vi "Gestore procedure.vi"() -> ()   [LabVIEW 2019]
uses:
  TypeDef/Operazioni.ctl
  TypeDef/PROCEDURE.ctl
  TypeDef/Control 1.ctl
  TypeDef/Impostazioni elettriche.ctl
  TypeDef/Collegamenti_elettrici.ctl
  TypeDef/Control rotore bloccato.ctl
  cDAQ_PLC Folder/cDAQ/SET ARRAY DO.ctl
  cDAQ_PLC Folder/cDAQ/SET SINGLE DO.ctl
  cDAQ_PLC Folder/cDAQ/DO List.ctl
  cDAQ_PLC Folder/cDAQ/SET ARRAY AO.ctl
  cDAQ_PLC Folder/cDAQ/SET SINGLE AO.ctl
  cDAQ_PLC Folder/cDAQ/AO List.ctl
  TypeDef/Cluster INFO.ctl
  TypeDef/WT SELECTION.ctl
  TypeDef/Definizione linea.ctl
  TypeDef/Control Calcoli.ctl
  Stato comandi freno.vi
  Stato alimentatore 1.vi
  Global FINE AVVIO.vi
  SubVI ELETTROTEST60A Folder/Elettrotest60A/Global_bypass_ResMeter.vi
  Global prova in corso.vi
  Global Trampa 0.vi
  Global stato profilo.vi
  Global Fine procedure.vi
  Global_All_Data.vi
  Global allarmi procedure.vi
panel:
  out "Elements In Queue":T1(array[cluster])
  out "Data":T2
  out "RESISTOMAT":T3
  out "PROCEDURA":string="MISURA RESISTENZA..."
  out "Element":T4
  out "OPERAZIONE IN CORSO":T5=enum."FRENO SET RIF PARTENZA"
  out "Message":string
  out "Stato":string
  out "Rami misura":i32
  out "Vi abilita pot":refnum<vi>
  out "Vi chiudi teler pot":refnum<vi>
  out "TEMPO PROVA ROT BLOCC":dbl
  in  "Cluster Colleg/LInea Elettrica":T6
  in  "AGGIUNGI PROCEDURA Abilita potenza":bool
  in  "AGGIUNGI PROCEDURA \nSTOP":bool
  in  "AGGIUNGI PROCEDURA \nSTART":bool
  in  "Cluster":T7={"MODALITA' BANCO"=enum."ALIMENTATORE E FRENO", "MODALITA' AVVIO MOTORE"=enum."AVVIO A TENSIONE RIDOTTA", "MODALITA' AVVIO FRENO"=enum."MARCIA PRIMA AVVIO", "V avvio[V]"=0.0, "F avvio[Hz]"=0.0, "%V ridotta"=0.0, "C avvio [Nm]"=0.0, "RPM avvio"=0.0, "SERVO AVVIO"=FALSE, "SENSO DI ROTAZIONE"=FALSE}
  out "Operazioni in corso":T5[](array[typedef])
  in  "EXIT":bool
  out "Matrice procedure":T5[][](array[typedef])
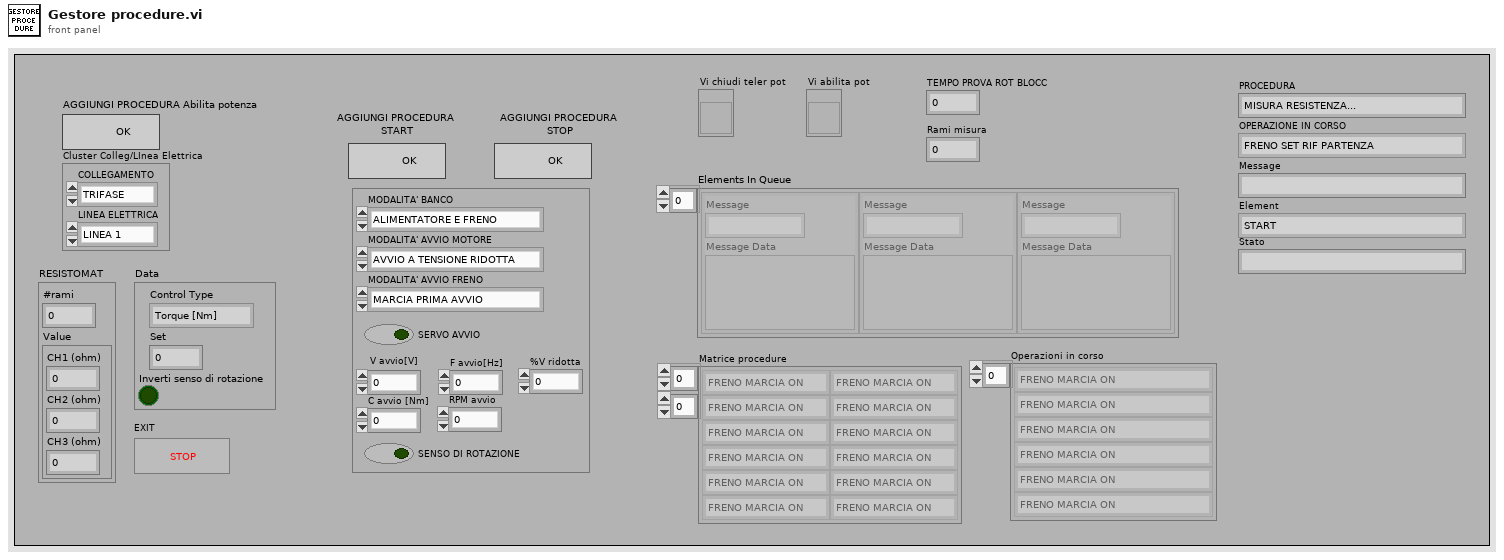
[diagram p1: front panel]
types:
  T1 = cluster{"Message":string, "Message Data":variant}[]
  T2 = cluster{"Control Type":enum32{"Torque [Nm]", "Power [W]", "Speed [RPM]"}, "Set":dbl, "Inverti senso di rotazione":bool}
  T3 = cluster{"#rami":i32, "Value":cluster{"CH1 (ohm)":u16, "CH2 (ohm)":u16, "CH3 (ohm)":u16}}
  T4 = typedef "PROCEDURE.ctl" = enum16{"START", "STOP AUTOMATICO", "STOP FRENO", "ABILITA POTENZA", "DISABILITA POTENZA", "CHIUDI POTENZA", "APRI POTENZA", "MISURA RESISTENZA RESISTOMAT", "PROVA ROTORE BLOCCATO", "MISURA RESISTENZA RES METER", "START AFE ALTERNATORI", "STOP AFE ALTERNATORI", "STOP ALIMENTATORE", "CONFIG CONTROLLO FRENO", "ALLARME", "START PROFILO", "SVUOTA BUFFER PROCEDURE E OPERAZIONI"}
  T5 = typedef "Operazioni.ctl" = enum32{"FINE", "FRENO ABILITA", "FRENO DISABILITA", "FRENO MARCIA ON", "FRENO MARCIA OFF", "FRENO SET RIF PARTENZA", "FRENO FORZA RIF FERMATA", "FRENO SET RIF FERMATA", "FRENO SET RIF A 0", "FRENO FORZA RIF A 0", "FRENO SET CONTROLLO COPPIA", "FRENO SET CONTROLLO VELOCITA'", "FRENO SET SENSO ROTAZIONE", "FRENO SET SENS ROT SEGNO COPPIA", "FRENO CONFIG", "ALIMENTATORE 1 ABILITA", "ALIMENTATORE 1 DISABILITA", "ALIMENTATORE 1 MARCIA ON", "ALIMENTATORE 1 MARCIA OFF", "ALIMENTATORE 1 SET RIF", "ALIMENTATORE 1 SET RIF RIDOTTO", "ALIMENTATORE 1 SET RIF A 0", "ALIMENTATORE 1 RESET ALLARMI", "ALIMENTATORE 1 SCORTA 2", "ALIMENTATORE 1 SCORTA 3", "ALIMENTATORE 2 ABILITA", "ALIMENTATORE 2 DISABILITA", "ALIMENTATORE 2 MARCIA ON", "ALIMENTATORE 2 MARCIA OFF", "ALIMENTATORE 2 SET RIF", "ALIMENTATORE 2 SET RIF RIDOTTO", "ALIMENTATORE 2 SET RIF A 0", "ALIMENTATORE 2 SCORTA 1", "ALIMENTATORE 2 SCORTA 2", "ALIMENTATORE 2 SCORTA 3", "TELERUTTORI CHIUDI POTENZA", "TELERUTTORI APRI POTENZA", "TELERUTTORI ABILITA POTENZA", "TELERUTTORI DISABILITA POTENZA", "TELERUTTORI MISURA RESISTENZA RESISTOMAT", "TELERUTTORI MISURA RESISTENZA RES METER", "PROCEDURA ROTORE BLOCCATO 1", "ATTENDI FERMATA MOTORE", "SEGNALA INIZIO AVVIO", "SEGNALA FINE AVVIO", "SEGNALA INIZIO FERMATA", "SEGNALA FINE FERMATA", "START PROFILO", "ATTENDI FINE RAMPA"}
  T6 = typedef "Control 1.ctl" = cluster{"COLLEGAMENTO":enum16{"TRIFASE", "MONOFASE", "DC MP", "DC"}, "LINEA ELETTRICA":enum16{"LINEA 1", "LINEA 2", "LINEA 3", "LINEA 4", "LINEA 5"}}
  T7 = typedef "Modalità avvio.ctl" = cluster{"MODALITA' BANCO":enum32{"ALIMENTATORE E FRENO", "SOLO ALIMENTATORE", "SOLO FRENO", "GESTIONE MANUALE", "SOLO ACQUISITORE", "VARIAC"}, "MODALITA' AVVIO MOTORE":enum32{"AVVIO A TENSIONE RIDOTTA", "AVVIO IN RAMPA", "AVVIO DIRETTO DA ALIM", "AVVIO DIRETTO DA LINEA"}, "MODALITA' AVVIO FRENO":enum32{"MARCIA DOPO AVVIO MOTORE", "MARCIA PRIMA AVVIO"}, "V avvio[V]":dbl, "F avvio[Hz]":dbl, "%V ridotta":dbl, "C avvio [Nm]":dbl, "RPM avvio":dbl, "SERVO AVVIO":bool, "SENSO DI ROTAZIONE":bool}
  T8 = cluster{"Message":string, "Message Data":variant}
  T9 = typedef "Impostazioni elettriche.ctl" = cluster{"COLLEGAMENTO":T10, "LINEA ELETTRICA":enum16{"LINEA 1", "LINEA 2", "LINEA 3", "LINEA 4", "LINEA 5"}}
  T10 = typedef "Collegamenti_elettrici.ctl" = enum16{"AC TRIFASE", "AC TRIFASE + FRENO", "AC MONOFASE", "DC CON ECCITAZIONE", "DC CON ECCITAZIONE + FRENO", "DC NO ECCITAZIONE", "DC NO ECCITAZIONE + FRENO", "FRENO TRASC + AFE", "SOLO FRENO", "CARICO RESISTIVO", "GENERICO", "SOLO ACQUISITORE", "SCORTA 4", "SCORTA 5", "SCORTA 6"}
  T11 = typedef "Control rotore bloccato.ctl" = cluster{"TEMPO PROVA":dbl}
  T12 = cluster{"Array of elements":cluster{"String":string, "variant":variant}[], "Single element":cluster{"String":string, "variant":variant}, "enque at\nopposite end (F)":bool, "no replications (F)":bool}
  T13 = typedef "SET ARRAY DO.ctl" = T14[]
  T14 = typedef "SET SINGLE DO.ctl" = cluster{"DO":T15, "Value":bool}
  T15 = typedef "DO List.ctl" = enum16{"OFF: ALL DO", "*ABILITA freno 1", "*ABILITA freno 2", "*ABILITA freno 3", "*START freno 1", "*START freno 2", "*START freno 3", "*STOP freno 1", "*STOP freno 3", "*STOP freno 2", "*Senso rot freno 1", "*Senso rot freno 2", "*Senso rot freno 3", "*Ctrl velocità freno 1", "*Ctrl velocità freno 2", "*Ctrl velocità freno 3", "*Ctrl coppia freno 1", "*Ctrl coppia freno 2", "*Ctrl coppia freno 3", "*ABILITA alimentatore 1", "*ABILITA alimentatore 2", "*ABILITA alimentatore 3", "*ABILITA alimentatore 4", "*START alimentatore 1", "*START alimentatore 2", "*START alimentatore 3", "*START alimentatore 4", "*STOP alimentatore 1", "*STOP alimentatore 2", "*STOP alimentatore 3", "*STOP alimentatore 4", "SENSO ROT alimentatore 1", "SENSO ROT alimentatore 2", "Abilita LEM 1000A", "Abilita LEM 300A", "Abilita sensori EXT WT", "B1 Seleziona linea 1", "B1 Seleziona linea 2", "B1 Seleziona linea 3", "B1 Seleziona linea 4", "B1 Seleziona linea 5", "B2 Seleziona linea 1", "B2 Seleziona linea 2", "B2 Seleziona linea 3", "B2 Seleziona linea 4", "B2 Seleziona linea 5", "*Reset allarmi", "*Start potenza AC", "*Stop potenza AC", "*Start potenza DC", "*Stop potenza DC", "*Start potenza DC eccit", "*Stop pontenza DC eccit", "Bypass res meter", "2nd canale res meter", "Enable res meter", "*Abilit teler ramo WT", "*Abil teler ramo princ Resit", "*Abil teler ramo 1 Resist", "*Abil teler ramo 2 Resist", "*Abil teler ramo 3 Resist", "*Abil cortocirc avvolgim", "*Controllo torsiometro B1", "*Controllo Torsiom B2", "*Scala torsiometro B1", "*Scala torsiometro B2", "*Collaudo in corso", "*Allarme presente", "Abilitazione elettroserratura", "Exit", "*Abilita collaudo", "*Abilita potenza trifase", "*Abilita potenza monofase", "*Abilita potenza DC", "*Abilita potenza DC eccit", "*Disabilita teleruttori potenza", "Set teleruttori prova a freddo", "Prova a freddo monofase", "Watchdog", "Forza DO PLC 3", "Forza DO PLC 2", "Forza DO PLC 1", "Forza DO cDAQ", "Scala 2000(T) 200(F) res meter", "Seleziona banco 1", "Seleziona banco 2", "Comando azionam in blocco", "Comando azionam reset", "Sensibilità freno 16 32 nm", "Reset Allarmi", "Carico res - Ramo 1", "Carico res - Ramo 2", "Carico res - Ramo 3", "Carico res - Ramo 4", "Carico res - Ramo 5", "Carico res - Ramo 6", "Carico res - Ramo 7", "Carico res - Ramo 8", "Carico res - Ramo 9", "Carico res - Ramo 10", "Carico res - Ramo 11", "Carico res - Start ventilatore", "Carico res - Stop ventilatore", "Abilita potenza solo freno", "Abilita AFE + freno trasc", "Abilita potenza carico resistivo", "Chiudi potenza AFE", "Apri potenza AFE", "Start AFE", "Config Banco2 TDE", "Misura diretto WT", "Ripristina centralina protezioni", "Abilita Scrittura Dati Keb", "Bench Selection(0-B1,1-B2)", "Select current mode", "Select torque mode", "Select speed mode", "Extenal alarm", "Enable Extenal program ", "Start ", "Stop", "Enable force mode", "Abilita linea 125 A", "Abilita linea 63 A", "Abilita linea 16 A", "Aum Tensione Variac", "Dim Tesnione Variac", "Abilita Ellecto Stractura", "Riprinto Emergenxe ", "Abilita Collaudo", "Disabilita Collaudo", "Abilita Ingresso Variac", "Abilita Uscita Variac", "Abilita ventilatore Variac"}
  T16 = enum32{"Torque [Nm]", "Power [W]", "Speed [RPM]"}
  T17 = typedef "SET ARRAY AO.ctl" = T18[]
  T18 = typedef "SET SINGLE AO.ctl" = cluster{"AO":T19, "Value":dbl}
  T19 = typedef "AO List.ctl" = enum16{"OFF: ALL AO", "RIF VEL FRENO 1", "RIF VEL FRENO 2", "RIF VEL FRENO 3", "RIF COPPIA FRENO", "RIF COPPIA FRENO 1", "RIF COPPIA FRENO 2", "RIF COPPIA FRENO 3", "RIF CORRENTE FRENO 2", "RIF V ALIM 1", "RIF F ALIM 1", "RIF V ALIM 2", "RIF F ALIM 2", "RIF V ALIM 3", "RIF F ALIM 3", "RIF V ALIM 4", "RIF F ALIM 4", "FORZA AO PLC 3", "FORZA AO PLC 2", "FORZA AO PLC 1", "FORZA AO cDAQ", "Configura alimentatore keb", "Tempo rampa keb", "Condensatori", "Exit"}
  T20 = cluster{"N°Acq":i16, "Periodo":dbl, "acq in corso":bool, "Acquisizione":bool, "Slide":u8, "Inserisci Acq.":bool, "Elimina riga":bool, "Acq auto":bool, "Intervallo":dbl}
  T21 = typedef "Cluster INFO.ctl" = cluster{"Scelta wattmetro":cluster{"Wattmetro":T22}, "SET RPM":dbl, "SET TEMP":dbl, "Array banchi":T23[], "Array valvole linee avvio/fermata":cluster{"Valvole avvio":cluster{"Set valvole avvio?":bool, "% valvole avvio":dbl[]}, "Valvole fermata":cluster{"Set valvole fermata?":bool, "% valvole fermata":dbl[]}}[], "banco selezionato":i8, "Nomi valvole prop sistema":string[], "canale-- sensore":string[][], "Attriti B1":dbl[][], "Attriti B2":dbl[][], "Collegamento elettrico":cluster{"ALIMENTAZIONE ELETTRICA":T10, "ID":i16, "#rami freddo\\eq term resmeter":i16, "#rami riscaldamento resmeter":i16, "#rami freddo\\eq term resistomat":i16, "#rami riscaldamento resistomat":i16, "CALCOLI":T24}, "lingua":i16, "Costanti collaudo":cluster{"P [bar]":dbl, "T amb. [°C]":dbl, "Umidità [%]":dbl, "T acqua [°C] 2":dbl}, "OPZIONI MISURE RES":cluster{"MISURA A FREDDO":enum16{"NESSUNO", "RESISTOMAT", "RES METER", "ENTRAMBI"}, "MISURA EQ. TERMICO":enum16{"NESSUNO", "RESISTOMAT", "RES METER", "ENTRAMBI"}, "MISURA DT PROVA IN CORSO":enum16{"NESSUNO", "RESISTOMAT - CON FERMATE", "RES METER - CON FERMATE", "RES METER - CONTINUO"}, "MISURE PRIMA E DOPO":enum16{"NESSUNO", "RESISTOMAT", "RES METER"}, "STRUMENTI PRESENTI":enum16{"NESSUNO", "RESISTOMAT", "RES METER", "ENTRAMBI"}}, "Dati targa motore":cluster{"Vnom":dbl, "Fnom":dbl, "Inom":dbl, "Cnom":dbl, "Npoli":dbl, "Scorta 1":dbl, "Scorta 2":dbl, "Scorta 3":dbl}}
  T22 = typedef "WT SELECTION.ctl" = enum32{"No Selection", "WT230", "WT333", "WT1800", "WT330", "VIW", "APLUS"}
  T23 = typedef "Definizione linea.ctl" = cluster{"Nome":string, "Tors. scala1":i32, "Tors. scala2":i32, "rpm":i32, "TAMB":i32, "Indici Temperature":i16[], "Indice freno":i16, "alimentatore trifase":i16, "alimentatore monofase":i16, "alimentatore dc arm":i16, "alimentatore dc ecc":i16, "alimentatore dc mp":i16}
  T24 = typedef "Control Calcoli.ctl" = enum16{"AC TRIFASE", "AC MONOFASE", "DC ECCITAZIONE", "DC NO ECCITAZIONE", "POMPA TRIFASE", "POMPA MONOFASE", "GENERICO", "TRASFORMATORE", "ALTERNATORE TRASCINATO", "GRUPPO ELETTROGENO"}
  T25 = typedef "Stato inverter selezionato.ctl" = cluster{"Stato comandi freno":T26, "Stato":cluster{"rif C%":dbl, "rif vel%":dbl, "Controllo effettivo":enum32{"Torque [Nm]", "Power [W]", "Speed [RPM]"}, "Controllo desiderato":enum32{"Torque [Nm]", "Power [W]", "Speed [RPM]"}, "Fine rampa C":bool, "Fine rampa RPM":bool, "Senso rotaz":bool, "Start":bool, "C stabile":bool, "P stabile":bool, "RPM stabile":bool}}
  T26 = typedef "Comandi freno.ctl" = cluster{"Control":cluster{"Control Type":enum32{"Torque [Nm]", "Power [W]", "Speed [RPM]", "Corrente [A]"}, "Set":dbl, "Inverti senso di rotazione":bool}, "Start\\stop":cluster{"Start":bool, "STOP":bool}, "Status":cluster{"Ready":bool, "Running":bool, "Regulation":bool}, "PID":bool, "Abilita":cluster{"Abilita":bool}, "Status ref":cluster{"Torque":dbl, "Speed":dbl}}
  T27 = typedef "Comandi_Alimentatore.ctl" = cluster{"RIF 1":dbl, "RIF 2":dbl, "Status":cluster{"Ready":bool, "Running":bool, "Regulation":bool}, "Start\\stop":cluster{"Start":bool, "Stop":bool}, "PID RIF1":bool, "PID RIF2":bool, "Status ref":cluster{"RIF 1":dbl, "RIF 2":dbl}, "Abilita":cluster{"Abilita":bool}}
  T28 = cluster{"RIF 1":dbl, "RIF 2":dbl, "Abilitato":bool, "In marcia":bool, "Fine rampa RIF1":bool, "Fine rampa RIF2":bool, "Vstabile":bool, "F stabile":bool, "PID RIF1":bool, "PID RIF2":bool, "Alimentatore 1":T27}
  T29 = cluster{"rif C%":dbl, "rif vel%":dbl, "Controllo effettivo":enum32{"Torque [Nm]", "Power [W]", "Speed [RPM]"}, "Controllo desiderato":enum32{"Torque [Nm]", "Power [W]", "Speed [RPM]"}, "Fine rampa C":bool, "Fine rampa RPM":bool, "Senso rotaz":bool, "Start":bool, "C stabile":bool, "P stabile":bool, "RPM stabile":bool}
  T30 = enum32{"ALIMENTATORE E FRENO", "SOLO ALIMENTATORE", "SOLO FRENO", "GESTIONE MANUALE", "SOLO ACQUISITORE", "VARIAC"}
  T31 = enum32{"AVVIO A TENSIONE RIDOTTA", "AVVIO IN RAMPA", "AVVIO DIRETTO DA ALIM", "AVVIO DIRETTO DA LINEA"}
  T32 = enum32{"MARCIA DOPO AVVIO MOTORE", "MARCIA PRIMA AVVIO"}
  T33 = cluster{"IN ESECUZIONE":bool, "IN PAUSA":bool, "FINE":bool, "Tstep":dbl}
  T34 = typedef "Cluster MISURE.ctl" = cluster{"MISURE NM":T35, "MISURE ALL":T36}
  T35 = typedef "MISURE NM.ctl" = cluster{"Banco":string, "Anno":string, "Numero":string, "Ntabella":string, "Misura":string, "Tipo Prova":string, "ProgressivoAcq":string, "Descrizione":string, "Data_ora":string, "t. acq [h:m:s]":string, "t. acq [min]":string, "t. acq [s]":string, "n [rpm]":string, "f [Hz]":string, "U1[V]":string, "U2 [V]":string, "U3 [V]":string, "U123_media [V]":string, "I1[A]":string, "I2[A]":string, "I3[A]":string, "I123_media [A]*I":string, "I_123_sbil [%]":string, "Ulin[V]":string, "Uc [V]":string, "Uaux [V]":string, "Ilin[A]*I":string, "Imar[A]":string, "Iaux[A]":string, "Uarm[V]":string, "Uecc[V]":string, "Iarm[A]*I":string, "Iecc[A]":string, "pf":string, "P1 [W]":string, "P1 [kW]":string, "Q [VAR]":string, "Q [kVAR]":string, "S [VA]":string, "S [kVA]":string, "P1arm[W]":string, "P1ecc[W]":string, "Parm[kW]":string, "P1ecc[kW]":string, "Cond[uF]":string, "P1_linea_6fili[W]":string, "P1_linea_6fili[kW]":string, "eta_gr_6fili [%]":string, "eta_inverter_6fili [%]":string, "pf_linea_6fili":string, "U4 [V]":string, "U5 [V]":string, "U6 [V]":string, "U456_media [V]":string, "I4 [A]":string, "I5 [A]":string, "I6 [A]":string, "I456_media [A]":string, "C [Nm]*C":string, "Cric [Nm]":string, "Cric\\Cnom":string, "Iric[A]":string, "Iric\\Inom":string, "P2_mecc [W]":string, "P2_mecc [kW]":string, "eta motore [%]":string, "Scorr[%]":string, "Tamb[°C]":string, "R1[ohm]":string, "R2[ohm]":string, "R3[ohm]":string, "Rmedia[ohm]":string, "DT_R1[°C]":string, "DT_R2[°C]":string, "DT_R3[°C]":string, "DT_media[°C]":string, "R_marcia[ohm]":string, "R_aux[ohm]":string, "DT_marcia[°C]":string, "DT_aux[°C]":string, "R_Arm[ohm]":string, "R_Ecc[ohm]":string, "DT_Arm[°C]":string, "DT_Ecc[°C]":string, "TambFreddo[°C]":string, "R1_freddo[ohm]":string, "R2_freddo[ohm]":string, "R3_freddo[ohm]":string, "Rmedia_freddo[ohm]":string, "R_Marcia_freddo[ohm]":string, "R_Aux_freddo[ohm]":string, "R_Arm_freddo[ohm]":string, "R_Ecc_freddo[ohm]":string, "TC1 [°C]":string, "TC2 [°C]":string, "TC3 [°C]":string, "TC4 [°C]":string, "TC5 [°C]":string, "TC6 [°C]":string, "TC7 [°C]":string, "TC8 [°C]":string, "PT1000_1[°C]":string, "PT1000_2[°C]":string, "PT1000_3[°C]":string, "Vdc eccitatrice[V]":string, "Idc eccitatrice[A]":string, "Vdc rotore[V]":string, "Idc rotore[A]":string, "Vac rotore[V]":string, "Iac rotore[V]":string, "V dinamo[V]":string, "Portata Q":string, "Pressione H":string, "U1'[V]":string, "U2'[V]":string, "U3'[V]":string, "I1'[A]":string, "I2'[A]":string, "I3'[A]":string, "U''R-N":string, "U''S-N":string, "U'' T-N":string, "U''R-S":string, "U''R-T":string, "U''S-T":string, "I1''[A]":string, "I2''[A]":string, "I3''[A]":string, "F''[Hz]":string, "P''[kW]":string, "CosFi''":string, "PT1000_4[°C]":string, "Scorta 3":string}
  T36 = typedef "Cluster misure ALL.ctl" = cluster{"Cluster READ NI":T37, "MISURE WT":T40, "Resistenze Resistomat":T41, "INTERFACCIA":T42, "FREDDO resistomat":cluster{"Res Ch1":dbl, "Res Ch2":dbl, "tAMB":dbl, "Res Ch3":dbl}, "STATO PLC 1":T47, "Res Ch2":dbl, "Res Ch2 2":dbl, "FREDDO res meter":cluster{"Res Ch1":dbl, "Res Ch2":dbl, "tAMB":dbl, "Res Ch3":dbl}, "Resistenze Res Meter":T41, "READ SINUS PENTA":T51, "STATO PLC 2":T52, "STATO PLC 3":T56, "DCREG":T60}
  T37 = typedef "Cluster NI.ctl" = cluster{"AI (0-10V)":cluster{"AI 0":dbl, "AI 1":dbl, "AI 2":dbl, "AI 3":dbl, "AI 4":dbl, "AI 5":dbl, "AI 6":dbl, "AI 7":dbl, "AI 8":dbl, "AI 9":dbl, "AI 10":dbl, "AI 11":dbl, "AI 12":dbl, "AI 13":dbl, "AI 14":dbl, "AI 15":dbl, "AI 16":dbl, "AI 17":dbl, "AI 18":dbl, "AI 19":dbl, "AI 20":dbl, "AI 21":dbl, "AI 22":dbl, "AI 23":dbl, "AI 24":dbl, "AI 25":dbl, "AI 26":dbl, "AI 27":dbl, "AI 28":dbl, "AI 29":dbl, "AI 30":dbl, "AI 31":dbl}, "StatoAO_Cdaq[0-10V]":cluster{"AO 1":dbl, "AO 2":dbl, "AO 3":dbl, "AO 4":dbl}, "Contatori [rpm]":cluster{"RPM 1":dbl, "RPM 2":dbl}, "StatoAO_Cdaq [4-20mA]":T38, "StatoDO_Cdaq":T39, "DI":cluster{"Scorta 0":bool, "Scorta 1":bool, "Scorta 2":bool, "Scorta 3":bool, "Scorta 4":bool, "Scorta 5":bool, "Scorta 6":bool, "Scorta 7":bool, "Scorta 8":bool, "Scorta 9":bool, "Scorta 10":bool, "Scorta 11":bool, "Scorta 12":bool, "Scorta 13":bool, "Scorta 14":bool, "Scorta 15":bool, "Scorta 16":bool, "Scorta 17":bool, "Scorta 18":bool, "Scorta 19":bool, "Scorta 20":bool, "Scorta 21":bool, "Scorta 22":bool, "Scorta 23":bool, "Scorta 24":bool, "Scorta 25":bool, "Scorta 26":bool, "Scorta 27":bool, "Scorta 28":bool, "Scorta 29":bool, "Scorta 30":bool, "Scorta 31":bool}, "AI (4-20mA)":cluster{"AI 0":dbl, "AI 1":dbl, "AI 2":dbl, "AI 3":dbl, "AI 4":dbl, "AI 5":dbl, "AI 6":dbl, "AI 7":dbl, "AI 8":dbl, "AI 9":dbl, "AI 10":dbl, "AI 11":dbl, "AI 12":dbl, "AI 13":dbl, "AI 14":dbl, "AI 15":dbl}, "TC [°C]":cluster{"tc 1":dbl, "tc 2":dbl, "tc 3":dbl, "tc 4":dbl}, "NI Read Values":cluster{"RPM":dbl, "Frequency":dbl, "Mod 1":cluster{"Torsiometro 1":dbl, "Torsiometro 2":dbl, "Strin Gauge 1":dbl, "Strin Gauge 2":dbl}, "Mod 2":cluster{"Termocoppia 1":dbl, "Termocoppia 2":dbl, "Termocoppia 3":dbl, "Termocoppia 4":dbl}, "Mod 3":cluster{"PT 100 1":dbl, "PT 100 2":dbl, "PT 100 3":dbl, "PT 100 4":dbl}}}
  T38 = typedef "StatoAO_cdaq.ctl" = cluster{"Cdaq_AO [0-10V] 0 for Torque":dbl, "Cdaq_AO [0-10V] 1":dbl, "Cdaq_AO [0-10V] 2":dbl, "Cdaq_AO [0-10V] 3":dbl}
  T39 = typedef "statoDO_Cdaq.ctl" = cluster{"Scorta 0":bool, "Scorta 1":bool, "Scorta 2":bool, "Scorta 3":bool, "Scorta 4":bool, "Scorta 5":bool, "Scorta 6":bool, "Scorta 7":bool, "Scorta 8":bool, "Scorta 9":bool, "Scorta 10":bool, "Scorta 11":bool, "Scorta 12":bool, "Scorta 13":bool, "Scorta 14":bool, "Scorta 15":bool, "Scorta 16":bool, "Scorta 17":bool, "Scorta 18":bool, "Scorta 19":bool, "Scorta 20":bool, "Scorta 21":bool, "Scorta 22":bool, "Scorta 23":bool, "Scorta 24":bool, "Scorta 25":bool, "Scorta 26":bool, "Scorta 27":bool, "Scorta 28":bool, "Scorta 29":bool, "Scorta 30":bool, "Scorta 31":bool}
  T40 = typedef "MISURE WT.ctl" = cluster{"URMS 1":dbl, "IRMS 1":dbl, "P 1":dbl, "S 1":dbl, "Q 1":dbl, "LAMBDA 1":dbl, "PHI 1":dbl, "F U 1":dbl, "F I 1":dbl, "NONE 1":dbl, "URMS 2":dbl, "IRMS 2":dbl, "P 2":dbl, "S 2":dbl, "Q 2":dbl, "LAMBDA 2":dbl, "PHI 2":dbl, "F U 2":dbl, "F I 2":dbl, "NONE 2":dbl, "URMS 3":dbl, "IRMS 3":dbl, "P 3":dbl, "S 3":dbl, "Q 3":dbl, "LAMBDA 3":dbl, "PHI 3":dbl, "F U 3":dbl, "F I 3":dbl, "NONE 3":dbl, "URMS SIGMA":dbl, "IRMS SIGMA":dbl, "P SIGMA":dbl, "S SIGMA":dbl, "Q SIGMA":dbl, "LAMBDA SIGMA":dbl, "PHI SIGMA":dbl, "F U SIGMA":dbl, "F I SIGMA":dbl, "NONE 4":dbl}
  T41 = typedef "ClusterRes.ctl" = cluster{"Res Ch1":dbl, "Res Ch2":dbl, "Res Ch3":dbl, "Tamb":dbl}
  T42 = typedef "INTERFACCIA.ctl" = cluster{"AI":cluster{"Portate":T43[], "Pressioni":T43[], "Coppie[Nm]":T43[], "Valvole prop %":T43[], "RPM":T43[], "Livelli":T43[], "Temperature":T43[], "Riferimenti %":T43[], "TENSIONI":T43[], "CORRENTI":T43[]}, "DI (logici)":cluster{"Start da pulsantiera":bool, "Stop da pulsantiera":bool, "Reset da pulsantiera":bool, "Sistema OK":bool, "Collaudo abilitato":bool, "Potenza trifase abilitata":bool, "Potenza monofase abilitata":bool, "Potenza DC abilitata":bool, "Potenza DC ECC abilitata":bool, "Start alimentazione AC":bool, "Start alimentazione DC":bool, "Start DC eccitazione":bool, "Teleruttore WT abilitato":bool, "Teleruttore Resistomat abilitato":bool, "Teleruttore corto fasi":bool, "Ramo 1 resistomat":bool, "Ramo 2 resistomat":bool, "Ramo 3 resistomat":bool, "B1 Scelta linea elettrica 1":bool, "B1 Scelta linea elettrica 2":bool, "B1 Scelta linea elettrica 3":bool, "B1 Scelta linea elettrica 4":bool, "B1 Scelta linea elettrica 5":bool, "B2 Scelta linea elettrica 1":bool, "B2 Scelta linea elettrica 2":bool, "B2 Scelta linea elettrica 3":bool, "B2 Scelta linea elettrica 4":bool, "B2 Scelta linea elettrica 5":bool, "Rotore bloccato 1":bool, "Rotore bloccato 2":bool, "FRENO 1 abilitato":bool, "FRENO 1 run":bool, "FRENO 1 senso rotaz":bool, "FRENO 1 ctrl velocità":bool, "FRENO 2 abilitato":bool, "FRENO 2 run":bool, "FRENO 2 senso rotaz":bool, "FRENO 2 ctrl velocità":bool, "ALIM 1 abilitato":bool, "ALIM 1 run":bool, "ALIM 2 abilitato":bool, "ALIM 2 run":bool, "ALIM 3 abilitato":bool, "ALIM 3 run":bool, "FRENO 1 ctrl coppia":bool, "FRENO 2 ctrl coppia":bool, "FRENO 3 ctrl coppia":bool, "DI (logici) aggiuntivi impianto":cluster{"Solo freno abilitato":bool, "Carico resistivo abilitato":bool, "AFE+freno abilitato":bool, "Protezioni chiuse":bool, "Start potenza AFE":bool, "AFE in marcia":bool}, "Misura corrente diretta WT":bool, "Misura corrente sens ext":bool, "Sens ext abilitati":bool}, "AO non scalati":T45, "AO scalati":T45, "DO (logici)":T46}
  T43 = typedef "ClusterMisura_e_Unità_INPUT.ctl" = cluster{"Misura":dbl, "UM":T44, "Descrizione":string}
  T44 = typedef "UnitàMisura.ctl" = enum16{"V", "mA", "Bar", "RPM", "m3/s", "m3/min", "m3/h", "l/s", "l/min", "in3/min", "ft3/min", "gpm", "igpm", "igph", "%", "°C", "m", "Nm", "A"}
  T45 = typedef "Lista AO sistema.ctl" = cluster{"FRENO1 rif vel":dbl, "FRENO1 rif Coppia":dbl, "FRENO2 rif vel":dbl, "FRENO2 rif Coppia":dbl, "ALIM1 rif V":dbl, "ALIM1 rif F":dbl, "ALIM2 rif V":dbl, "ALIM2 rif F":dbl, "ALIM3 rif V":dbl, "ALIM3 rif F":dbl, "Fnom keb":dbl, "Rpm nom keb":dbl, "Pnom keb":dbl, "Inom keb":dbl, "Vnom keb":dbl, "Rpm max keb":dbl, "Tempo rampa keb":dbl, "Tipo Mot keb":dbl, "FRENO  rif Coppia ":dbl, "FRENO  rif  Corrente":dbl}
  T46 = typedef "DOinterfaccia.ctl" = cluster{"Scelta banco 1":bool, "Scelta banco 2":bool, "Scelta banco 3":bool, "FRENO 1 abilita":bool, "FRENO 1 start":bool, "FRENO 1 senso rotaz":bool, "FRENO 1 ctrl velocità":bool, "FRENO 2 abilita":bool, "FRENO 2 start":bool, "FRENO 2 senso rotaz":bool, "FRENO 2 ctrl velocità":bool, "ALIM 1 abilita":bool, "ALIM 1 start":bool, "ALIM 2 abilita":bool, "ALIM 2 start":bool, "ALIM 3 abilita":bool, "ALIM 3 start":bool, "Abilita linea trifase":bool, "Abilita linea monofase":bool, "Abilita linea dc":bool, "Abilita linea dc eccit":bool, "B1 Linea elettrica 1":bool, "B1 Linea elettrica 2":bool, "B1 Linea elettrica 3":bool, "B1 Linea elettrica 4":bool, "B1 Linea elettrica 5":bool, "B2 Linea elettrica 1":bool, "B2 Linea elettrica 2":bool, "B2 Linea elettrica 3":bool, "B2 Linea elettrica 4":bool, "B2 Linea elettrica 5":bool, "Start potenza AC":bool, "Stop pontenza AC":bool, "Start potenza DC":bool, "Stop potenza DC":bool, "Start potenza eccitaz":bool, "Stop potenza eccitaz":bool, "Reset allarmi":bool, "watchdog":bool, "Scala torsiometro B1":bool, "Controllo torsiom B1":bool, "Scala torsiometro B2":bool, "Controllo torsiom B2":bool, "Teleruttore WT abilita":bool, "Teleruttore Resistomat abilita":bool, "Teleruttore corto fasi":bool, "Ramo 1 resistomat":bool, "Ramo 2 resistomat":bool, "Ramo 3 resistomat":bool, "Collaudo in corso":bool, "Allarme presente":bool, "Enable Res Meter":bool, "Bypass Res Meter":bool, "2nd canale Res Meter":bool, "Scala 200/2000 res meter":bool, "Taratura res meter":bool, "FRENO 1 ctrl coppia":bool, "FRENO 2 ctrl coppia":bool, "FRENO 3 ctrl coppia":bool, "Aggiuntivi impianto":cluster{"Senso rotazione alim 1":bool, "Senso rotazione alim 2":bool}, "ALIM 1 stop":bool, "ALIM 2 stop":bool, "ALIM 3 stop":bool, "FRENO 1 stop":bool, "FRENO 2 stop":bool, "FRENO 3 stop":bool, "B1 configurazione freno B":bool, "B2 configurazione freno B":bool, "Abilita scrittura KEB":bool, "Bench Selection (0-B1,1-B2)":bool, "Select current mode":bool, "Select torque mode":bool, "Select speed mode":bool, "Start":bool, "Stop":bool, "Block":bool, "Enable Force mode":bool, "Abilita linea 125 A":bool, "Abilita linea 63 A":bool, "Abilita linea 16 A":bool, "Aum Tensione Variac":bool, "Dim Tesnione Variac":bool, "Abilita ellectro stractura":bool, "Risprinito Emergence":bool, "Abilita collaudo":bool, "Disabilita collaudo":bool, "External Alaram":bool, "Enable external program":bool, "Reset":bool, "Abilita Ingresso Variac":bool, "Abilita Ventilatore Variac":bool, "Abilita Uscita Variac ":bool}
  T47 = typedef "STATO PLC 1.ctl" = cluster{"USCITE PLC":T48, "Stato DI_PLC":cluster{"Sistema OK":bool, "Rotore bloccato":bool, "Scorta 1":bool, "Prova diretto inverter":bool, "Prova con filtro LC":bool, "Teleruttore WT abilitato":bool, "Alim sinus penta abilitato":bool, "Alim sinus penta in marcia":bool, "Freno abilitato":bool, "Freno in marcia":bool, "Senso rotazione freno":bool, "Potenza abilitata":bool, "Scorta 3":bool, "Scorta 4":bool, "scorta 5":bool, "scorta 6":bool}, "AI plc":cluster{"Allarmi 1":dbl, "Allarmi 2":dbl, "Scorta 1":dbl, "Scorta 2":dbl, "RPM mot prova":dbl, "I mot prova":dbl, "RPM freno":dbl, "I freno":dbl, "Scorta 3":dbl, "Scorta 4":dbl}}
  T48 = typedef "Uscite PLC 1.ctl" = cluster{"AO (real) 2":cluster{"SCORTA 1":dbl, "SCORTA 2":dbl, "SCORTA 3":dbl, "SCORTA 4":dbl, "SCORTA 5":dbl, "SCORTA 6":dbl, "SCORTA 7":dbl, "SCORTA 8":dbl}, "statoAO_PLC out":T49, "DO (bit)":T50}
  T49 = typedef "statoAO_plc_1.ctl" = cluster{"Rif Lim coppia freno [%]":dbl, "Rif rpm freno [%]":dbl, "Rif coppia freno [%]":dbl, "Rif V alimentatore [%]":dbl, "Rif F alimentatore [%]":dbl}
  T50 = typedef "StatoDO_PLC_1.ctl" = cluster{"Scelta banco 1":bool, "Set dati motore freno 2":bool, "Diretto inverter":bool, "Filtro LC":bool, "Marcia ALIM (1s)":bool, "Marcia FRENO (1s)":bool, "Stop AFE (1s)":bool, "Stop freno (1s)":bool, "Reset allarmi":bool, "Watchdog":bool, "Senso rotazione":bool, "Abilita collaudo (1s)":bool, "Disabilita collaudo (1s)":bool, "Abilitazione ALIM":bool, "Abilitazione FRENO":bool, "Teleruttore WT":bool, "Senso rot motore prova":bool, "Scorta 7":bool, "Scorta 8":bool, "Scorta 9":bool, "Scorta 10":bool, "Scorta 11":bool, "Scorta 12":bool, "Scorta 13":bool}
  T51 = typedef "Parametri inverter letti.ctl" = cluster{"Menù Misure motore (M000-M030)":cluster{"Rif vel a regime (int)":u16, "Rif vel a regime (dec)":u16, "Rif vel dopo rampe (int)":u16, "Rif vel dopo rampe (dec)":u16, "RPM motore (int)":u16, "RPM motore (dec)":u16, "FREQout inverter":u16, "Rif coppia a regime(Nm)":u16, "Richiesta di coppia (Nm)":u16, "Coppia generata dal motore(Nm)":u16, "Rif coppia a regime(%)":u16, "Richiesta di coppia (%)":u16, "Coppia generata dal motore(%)":u16, "Coppia max richiesta prima delle rampe(Nm)":u16, "Coppia max richiesta dopo le rampe(Nm)":u16, "Limite di velocità prima delle rampe":u16, "Limite di velocità dopo le rampe":u16, "Coppia max richiesta prima delle rampe(%)":u16, "Coppia max richiesta dopo le rampe(%)":u16, "Rif di flusso":u16, "Corrente di uscita":u16, "Capacità termica del motore":u16, "Tensione di uscita":u16, "Potenza di uscita":u16, "Energia consumata (LSword)":u16, "Energia consumata (MSword)":u16, "Tensione bus DC":u16, "Tensione di rete":u16}, "Menù regolatore PID (M018-M024)":cluster{"Rif PID a regime(%)":u16, "Rif pid dopo rampe(%)":u16, "Retroazione del pid(%)":u16, "Errore del pid(%)":u16, "uscita del pid(%)":u16, "Rif del pid dopo le rampe":u16, "Retroazione del pid":u16}, "Menù ingressi digitali (M031-M036)":cluster{"Ingressi digitali ritardati":u16, "Ingressi digitali istantanei":u16, "Moresettiera comando loc":u16, "Morsett comando da seriale":u16, "Morsett comando bus di campo":u16, "Ing dig ausiliari da morsettiera":u16, "Ing dig ausiliari da seriale":u16}, "Menù riferimenti (M037-M051)":cluster{"Rif analog est REF":u16, "Rif analog est AIN1":u16, "Rif analog est AIN2":u16, "Rif analog est XAIN4":u16, "Rif analog est XAIN5":u16, "Rif velocità da seriale(int)":u16, "Rif velocità bus di campo(int)":u16, "Rif coppia da seriale":u16, "Rif coppia bus di campo":u16, "Rif del PID da seriale":u16, "Rif del PID da bus di campo":u16, "Retroazione del PID da seriale":u16, "Retroazione del PIDda bus di campo":u16, "Rif da encoder":u16, "Rif in frequenza":u16, "Rif velocità da seriale(dec)":u16, "Rif velocità bus di campo(dec)":u16}, "Menù rampe (P009-P033)":cluster{"Tempo di dec rampa di vel 1":u16, "Tempo di acc rampa di vel 2":u16, "Tempo di dec rampa di vel 2":u16, "Tempo di acc rampa di vel 1":u16, "Unità di mis tempi rampe vel 1/2":u16, "Tempo di acc rampa di vel 3":u16, "Tempo di dec rampa di vel 3":u16, "Tempo di acc rampa di vel 4":u16, "Tempo di dec rampa di vel 4":u16, "Unità di mis tempi rampe vel 3/4":u16, "Selettore arrottondam rampe":u16, "Tempo di arrotond iniz rampa acc":u16, "Tempo di arrotond finale rampa acc":u16, "Tempo di arrotond iniz rampa dec":u16, "Tempo di rampa di salita rif coppia":u16, "Tempo di rampa di discesa rif coppia":u16, "Unità di misura rampa coppia":u16, "Tempo rampa acc marcia jog":u16, "Tempo rampa dec marcia jog":u16, "Reset acc ai cambi pendenza":u16, "rampa di acc in fire mode":u16, "rampa di dec in fire mode":u16, "Tempo di arrotond finale rampa dec":u16}, "Menù controllo motore(C008-C128)":cluster{"Numero motori configurati":u16, "Tipo algoritmo di controllo Mot1":u16, "Tipo rif Mot1":u16, "Tensione nominale rete":u16, "Retroaz di vel da encoder Mot1":u16, "Tipo curva V/f Mot1":u16, "Rotazione delle fasi Mot1":u16, "Freq nominale del motore Mot1":u16, "RPM nominali del motore Mot1":u16, "Potenza nominale del motore Mot1":u16, "Corrente nominale del motore Mot1":u16, "Tensione nominale del motore mot1":u16, "Potenza a vuoto del motore Mot1":u16, "Corrente a vuoto del motore Mot1":u16, "Resistenza statorica del motore Mot1":u16, "Induttanza di dispersione Mot1":u16, "Induttanza mutua motore":u16, "Costante di tempo rotorica":u16, "Costante di tempo filtro pb":u16, "Velocità minima motore":u16, "Velocità massima motore":u16}, "Menù configurazione PID":cluster{"Selezione riferimento n.1":u16, "Selezione retroazione n.1":u16, "Modalità di fuzionamento PID":u16, "Termine derivativo calcolato su err o mis":u16, "Proporz moltiplica deriv e integrale":u16, "Azione del PID":u16}, "ID":dbl, "Menù uscite digitali":cluster{"MDO4 Inverter pronto":u16}, "Fcarrier":cluster{"Fcarrier Min (Hz)":u16, "Fcarrier Max (Hz)":u16}, "stato inverter M089":dbl, "Riferimenti":cluster{"Rif tensione":u16, "Rif velocità":u16}, "Comunicazione":bool, "Modalità stop":dbl}
  T52 = typedef "STATO PLC 2.ctl" = cluster{"USCITE PLC":T53, "Stato DI_PLC":cluster{"Sistema ok":bool, "Relè Resistomat abilitato":bool, "Freno abilitato":bool, "Freno in marcia":bool, "scorta b":bool, "scorta a":bool, "scorta 1":bool, "scorta 2":bool, "scorta 3":bool, "scorta 4":bool, "Scorta 5":bool, "Scorta 6":bool, "Scorta 7":bool, "Scorta 8":bool, "Scorta 9":bool, "Scorta 10":bool}, "AI plc":cluster{"Allarmi 1":dbl, "Allarmi 2":dbl, "TC 1":dbl, "TC 2":dbl, "TC 3":dbl, "TC 4":dbl, "TC 5":dbl, "TC 6":dbl, "TC 7":dbl, "TC 8":dbl, "PT1000 1":dbl, "PT1000 2":dbl, "PT1000 3":dbl, "PT1000 4":dbl}}
  T53 = typedef "Uscite PLC 2.ctl" = cluster{"AO (real) 2":cluster{"SCORTA 1":dbl, "SCORTA 2":dbl, "SCORTA 3":dbl, "SCORTA 4":dbl, "SCORTA 5":dbl, "SCORTA 6":dbl, "SCORTA 7":dbl, "SCORTA 8":dbl}, "statoAO_PLC out":T54, "DO (bit)":T55}
  T54 = typedef "statoAO_plc_2.ctl" = cluster{"Condensatori":dbl, "Scorta 1":dbl, "Scorta 2":dbl}
  T55 = typedef "StatoDO_PLC_2.ctl" = cluster{"Relè misura resistomat":bool, "Misura res ramo 1":bool, "Misura res ramo 2":bool, "Misura res ramo 3":bool, "Scelta banco 2":bool, "Scala Torsiometro":bool, "Ctrl torsiometro":bool, "Select current mode":bool, "Select Torque mode":bool, "Select speed mode":bool, "Watchdog":bool, "Scorta":bool, "Scorta 2":bool, "Scorta 3":bool, "Scorta 4":bool, "Scorta 5":bool, "Bench selection":bool, "External alarm":bool, "Enable external program":bool, "Reset allarmi":bool, "Start":bool, "Stop":bool, "Block":bool, "Scorta 6":bool}
  T56 = typedef "STATO PLC 3.ctl" = cluster{"USCITE PLC":T57, "Stato DI_PLC":cluster{"Sistema OK":bool, "Rotore bloccato":bool, "Filtro LC":bool, "Bypass Filtro LC":bool, "Scelta Trasformatore":bool, "Scelta Bypass trasformatore":bool, "Teleruttore wt abilitato":bool, "Alimentatore abilitato":bool, "Alimentatore in marcia":bool, "Scorta 1":bool, "Scorta 2":bool, "Scorta 3":bool, "Potenza abilitata":bool, "Alimentatore in allarme":bool, "Scorta 4":bool, "Conferma dati KEB":bool, "Scorta 5":bool, "Warning Inverter Alimentatore":bool, "Variac Abilitato":bool, "Linea 125 A abilitata":bool, "Linea 63 A abilitata":bool, "Linea 16 A abilitata":bool, "Scorta 6":bool, "Enable force mode":bool}, "AI plc":cluster{"Allarmi 1":dbl, "Allarmi 2":dbl, "RPM motore prova":dbl, "Corrente motore prova":dbl, "RPM freno":dbl, "Corrente freno":dbl, "Tipo motore keb":dbl, "I nom keb":dbl, "RPM nom keb":dbl, "V nom keb":dbl, "F nom keb":dbl, "T rampa keb":dbl, "scorta":dbl, "Scorta 2":dbl}}
  T57 = typedef "Uscite PLC 3.ctl" = cluster{"AO (real) 2":cluster{"SCORTA 1":dbl, "SCORTA 2":dbl, "SCORTA 3":dbl, "SCORTA 4":dbl, "SCORTA 5":dbl, "SCORTA 6":dbl, "SCORTA 7":dbl, "SCORTA 8":dbl}, "statoAO_PLC out":T58, "DO (bit)":T59}
  T58 = typedef "statoAO_plc_3.ctl" = cluster{"Rif velocità alimentatore":dbl, "Scorta":dbl, "Tipo Motore  keb":dbl, "I nom keb":dbl, "RPM nom keb":dbl, "V nom keb":dbl, "F nom keb":dbl, "t rampa keb":dbl}
  T59 = typedef "StatoDO_PLC_3.ctl" = cluster{"Select linea Inverter":bool, "Abilita sense wattmetro":bool, "Bypass filtro LC":bool, "Filtro LC":bool, "Bypass trasformatore":bool, "Trasformatore":bool, "Abilita uscite variac":bool, "Abilita linea 125 A":bool, "Abilita linea 63 A":bool, "Abilita linea 16 A":bool, "Abilita Scrittura Dati Keb":bool, "Abilita alimentatore":bool, "Marcia alimentatore (1s)":bool, "Stop alimentatore (1s)":bool, "Senso rot mot prova":bool, "Watchdog":bool, "Aumenta tensione variac":bool, "Diminuisci tensione variac ":bool, "Blocco elettroserrature":bool, "Ripristino emergence":bool, "Abilita ingresso variac":bool, "Abilita ventilatore variac":bool, "Reset Allarm":bool, "Scorta 1":bool, "Scorta 2":bool, "Scorta 3":bool, "Scorta 4":bool, "Scorta 5":bool, "Scorta 6":bool, "Scorta 7":bool, "Scorta 8":bool, "Scorta 9":bool, "Abilita collaudo":bool, "Disabilita collaudo ":bool, "Scorta 10":bool, "Scorta 11":bool, "Scorta 12":bool, "Scorta 13":bool, "Scorta 14":bool, "Scorta 15":bool}
  T60 = typedef "Parametri DCREG letti.ctl" = cluster{"Parametri di misura":cluster{"M000":dbl, "M001":dbl, "M002":dbl, "M003":dbl, "M004":dbl, "M005":dbl, "M006":dbl, "M007":dbl, "M008":dbl, "M009":dbl, "M010":dbl, "M011":dbl, "M012":dbl, "M013":dbl, "M014":dbl, "M015":dbl, "M016":dbl, "M017":dbl, "M018":dbl, "M019":dbl, "M020":dbl, "M021":dbl, "M022":dbl, "M023":dbl, "M024":dbl, "M025":dbl, "M026":dbl, "M027":dbl, "M028":dbl, "M029":dbl, "M030":dbl, "M031":dbl}, "Parametri di programmazione":cluster{"P000":dbl, "P001":dbl, "P002":dbl, "P003":dbl, "P004":dbl, "P005":dbl, "P006":dbl, "P010":dbl, "P011":dbl, "P012":dbl, "P013":dbl, "P014":dbl, "P015":dbl, "P016":dbl, "P030":dbl, "P031":dbl, "P032":dbl, "P033":dbl, "P034":dbl, "P035":dbl, "P036":dbl, "P037":dbl, "P038":dbl, "P039":dbl, "P040":dbl, "P050":dbl, "P051":dbl, "P052":dbl, "P053":dbl, "P054":dbl, "P055":dbl, "P056":dbl, "P057":dbl, "P058":dbl, "P059":dbl, "P060":dbl, "P061":dbl, "P062":dbl, "P070":dbl, "P071":dbl, "P073":dbl, "P074":dbl, "P076":dbl, "P077":dbl, "P079":dbl, "P080":dbl, "P082":dbl, "P083":dbl, "P084":dbl, "P085":dbl, "P086":dbl, "P087":dbl, "P088":dbl, "P100":dbl, "P101":dbl, "P102":dbl, "P103":dbl, "P104":dbl, "P110":dbl, "P111":dbl, "P120":dbl, "P121":dbl, "P122":dbl, "P123":dbl, "P124":dbl, "P125":dbl, "P126":dbl, "P127":dbl, "P128":dbl, "P129":dbl, "P130":dbl, "P131":dbl, "P132":dbl, "P133":dbl, "P134":dbl, "P150":dbl, "P151":dbl, "P152":dbl, "P153":dbl, "P154":dbl, "P155":dbl, "P156":dbl, "P157":dbl, "P158":dbl, "P170":dbl, "P171":dbl, "P172":dbl, "P173":dbl, "P174":dbl, "P175":dbl, "P176":dbl, "P177":dbl, "P178":dbl, "P179":dbl, "P180":dbl, "P181":dbl, "P182":dbl, "P183":dbl, "P184":dbl, "P185":dbl, "P186":dbl, "P187":dbl, "P188":dbl, "P189":dbl, "P190":dbl, "P191":dbl, "P192":dbl, "P193":dbl, "P194":dbl, "P195":dbl, "P196":dbl, "P197":dbl, "P198":dbl, "P199":dbl, "P211":dbl, "P212":dbl, "P213":dbl, "P214":dbl, "P215":dbl, "P216":dbl, "P217":dbl, "P221":dbl, "P222":dbl, "P223":dbl, "P224":dbl, "P230":dbl, "P231":dbl, "P240":dbl, "P250":dbl, "P251":dbl}, "Parametri di configurazione":cluster{"C000":dbl, "C001":dbl, "C002":dbl, "C010":dbl, "C011":dbl, "C012":dbl, "C014":dbl, "C015":dbl, "C016":dbl, "C017":dbl, "C018":dbl, "C030":dbl, "C050":dbl, "C051":dbl, "C052":dbl, "C060":dbl, "C061":dbl, "C062":dbl, "C063":dbl, "C070":dbl, "C072":dbl, "C074":dbl, "C090":dbl, "C091":dbl, "C092":dbl, "C093":dbl, "C094":dbl, "C100":dbl, "C101":dbl, "C102":dbl, "C103":dbl, "C105":dbl, "C106":dbl, "C107":dbl, "C108":dbl, "C110":dbl, "C111":dbl, "C112":dbl, "C120":dbl, "C121":dbl, "C122":dbl, "C130":dbl, "C131":dbl, "C132":dbl, "C133":dbl, "C134":dbl, "C135":dbl, "C141":dbl, "C142":dbl, "C143":dbl, "C150":dbl, "C151":dbl, "C153":dbl, "C154":dbl, "C155":dbl, "C156":dbl, "C157":dbl, "C158":dbl, "C159":dbl, "C160":dbl, "C161":dbl, "C162":dbl, "C163":dbl, "C164":dbl, "C165":dbl, "C170":dbl}, "Codice allarme":dbl, "Comunicazione":bool}
  T61 = enum32{"Torque [Nm]", "Power [W]", "Speed [RPM]", "Corrente [A]"}
  T62 = enum16{"LINEA 1", "LINEA 2", "LINEA 3", "LINEA 4", "LINEA 5"}
  T63 = cluster{"Start da pulsantiera":bool, "Stop da pulsantiera":bool, "Reset da pulsantiera":bool, "Sistema OK":bool, "Collaudo abilitato":bool, "Potenza trifase abilitata":bool, "Potenza monofase abilitata":bool, "Potenza DC abilitata":bool, "Potenza DC ECC abilitata":bool, "Start alimentazione AC":bool, "Start alimentazione DC":bool, "Start DC eccitazione":bool, "Teleruttore WT abilitato":bool, "Teleruttore Resistomat abilitato":bool, "Teleruttore corto fasi":bool, "Ramo 1 resistomat":bool, "Ramo 2 resistomat":bool, "Ramo 3 resistomat":bool, "B1 Scelta linea elettrica 1":bool, "B1 Scelta linea elettrica 2":bool, "B1 Scelta linea elettrica 3":bool, "B1 Scelta linea elettrica 4":bool, "B1 Scelta linea elettrica 5":bool, "B2 Scelta linea elettrica 1":bool, "B2 Scelta linea elettrica 2":bool, "B2 Scelta linea elettrica 3":bool, "B2 Scelta linea elettrica 4":bool, "B2 Scelta linea elettrica 5":bool, "Rotore bloccato 1":bool, "Rotore bloccato 2":bool, "FRENO 1 abilitato":bool, "FRENO 1 run":bool, "FRENO 1 senso rotaz":bool, "FRENO 1 ctrl velocità":bool, "FRENO 2 abilitato":bool, "FRENO 2 run":bool, "FRENO 2 senso rotaz":bool, "FRENO 2 ctrl velocità":bool, "ALIM 1 abilitato":bool, "ALIM 1 run":bool, "ALIM 2 abilitato":bool, "ALIM 2 run":bool, "ALIM 3 abilitato":bool, "ALIM 3 run":bool, "FRENO 1 ctrl coppia":bool, "FRENO 2 ctrl coppia":bool, "FRENO 3 ctrl coppia":bool, "DI (logici) aggiuntivi impianto":cluster{"Solo freno abilitato":bool, "Carico resistivo abilitato":bool, "AFE+freno abilitato":bool, "Protezioni chiuse":bool, "Start potenza AFE":bool, "AFE in marcia":bool}, "Misura corrente diretta WT":bool, "Misura corrente sens ext":bool, "Sens ext abilitati":bool}
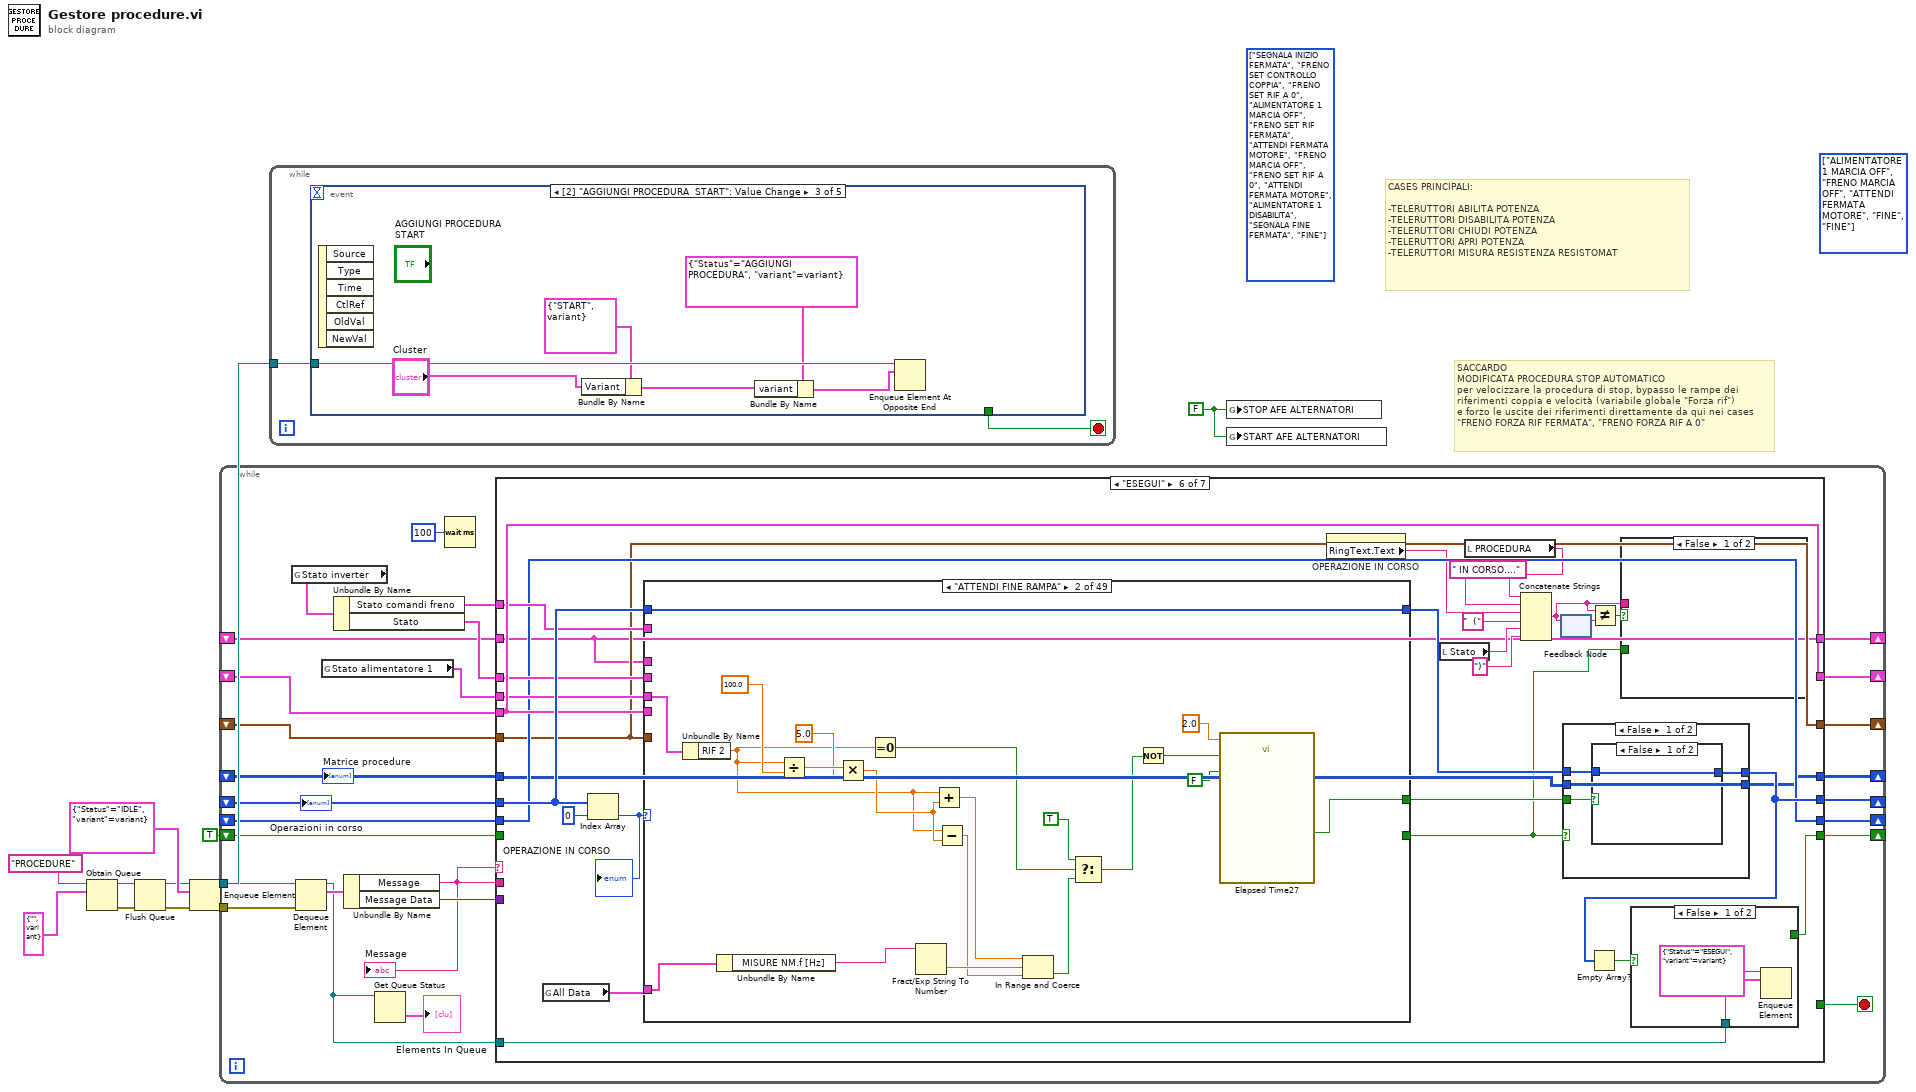
[diagram p0: block diagram]
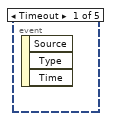
[diagram p2: hidden frame]
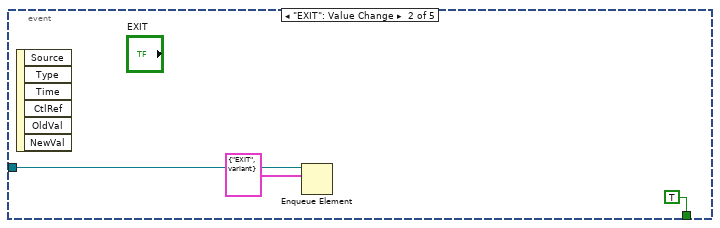
[diagram p3: hidden frame]
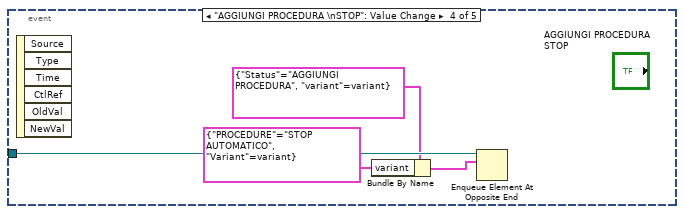
[diagram p4: hidden frame]
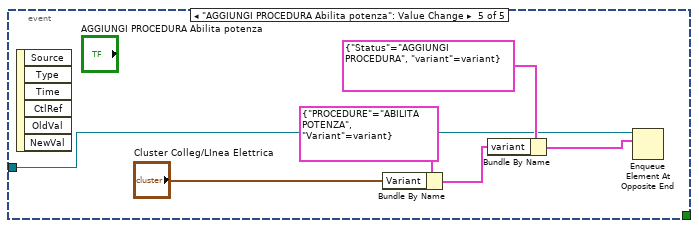
[diagram p5: hidden frame]
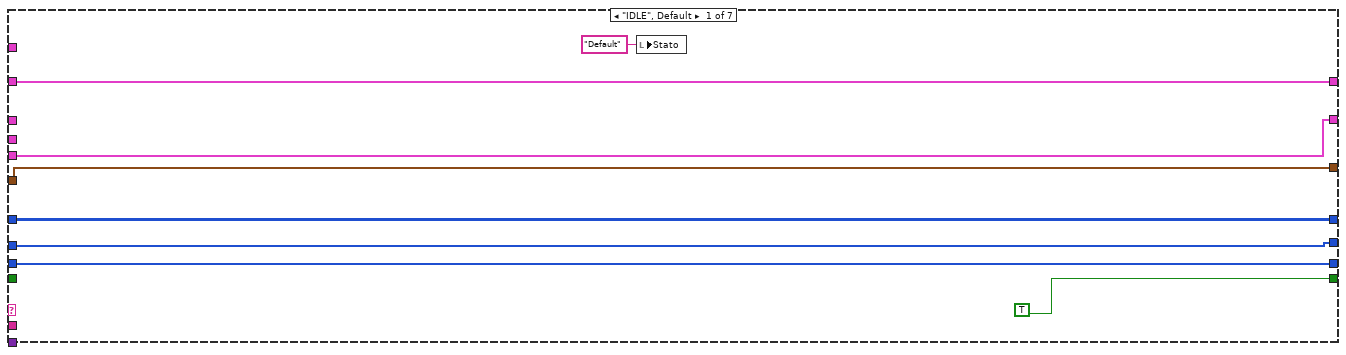
[diagram p6: hidden frame]
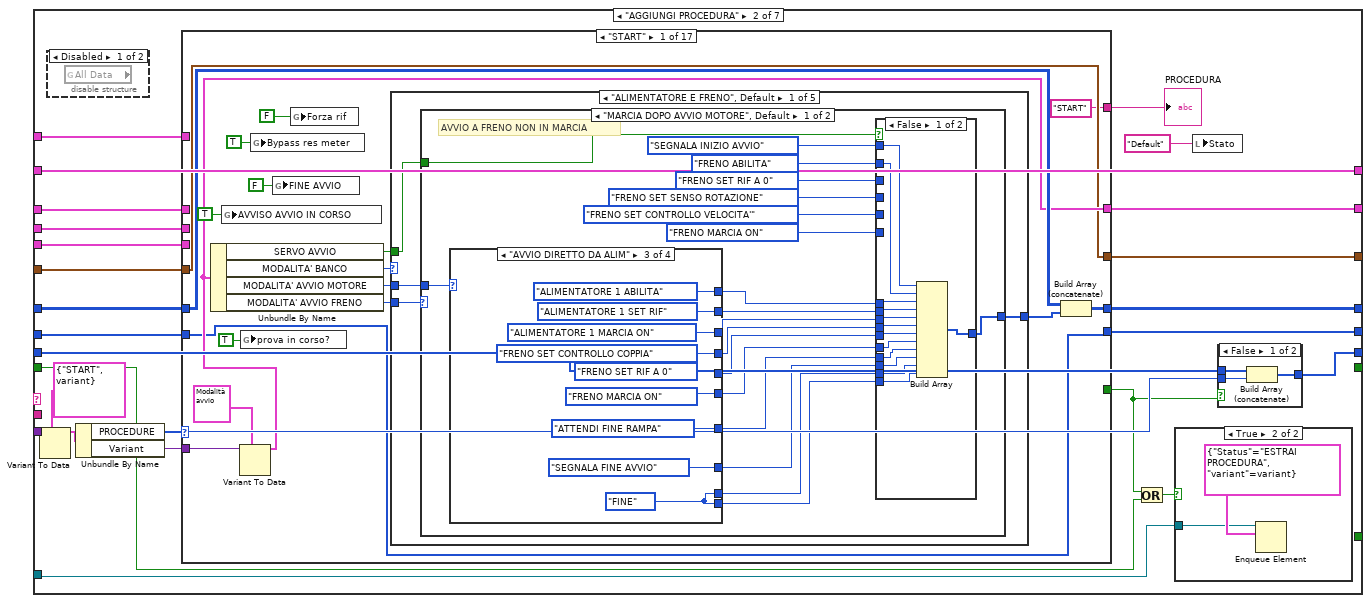
[diagram p7: hidden frame]
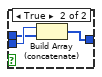
[diagram p9: hidden frame]
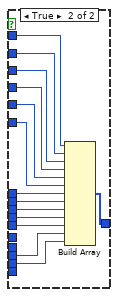
[diagram p11: hidden frame]
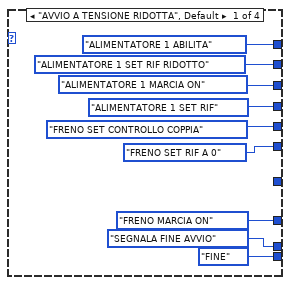
[diagram p12: hidden frame]
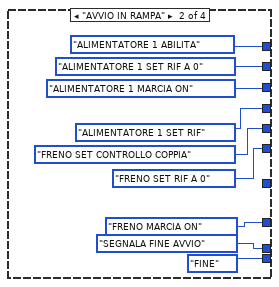
[diagram p13: hidden frame]
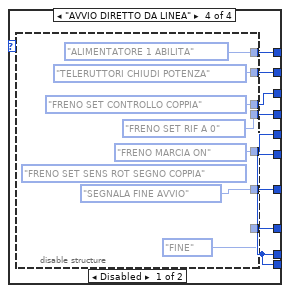
[diagram p14: hidden frame]
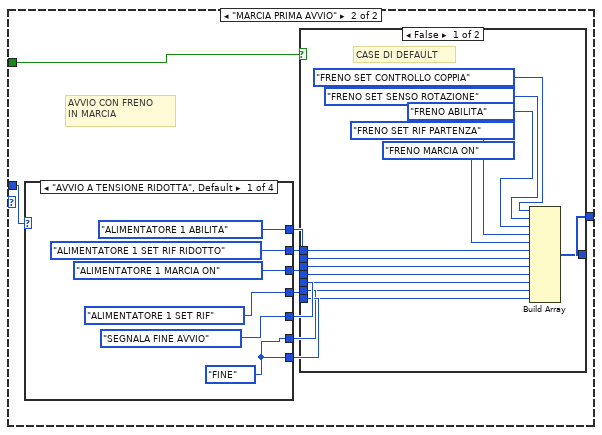
[diagram p16: hidden frame]
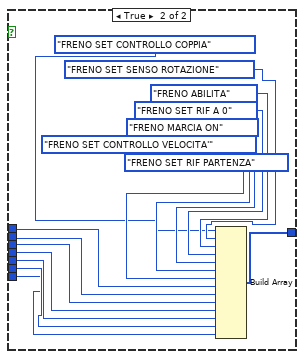
[diagram p17: hidden frame]
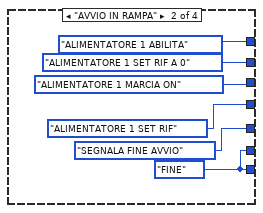
[diagram p18: hidden frame]
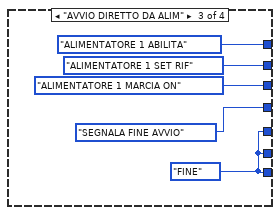
[diagram p19: hidden frame]
diagram:
  (unwired) T5[] [enum."SEGNALA INIZIO FERMATA", enum."FRENO SET CONTROLLO COPPIA", enum."FRENO SET RIF A 0", enum."ALIMENTATORE 1 MARCIA OFF", enum."FRENO SET RIF FERMATA", enum."ATTENDI FERMATA MOTORE", enum."FRENO MARCIA OFF", enum."FRENO SET RIF A 0", enum."ATTENDI FERMATA MOTORE", enum."ALIMENTATORE 1 DISABILITA", enum."SEGNALA FINE FERMATA", enum."FINE"] items=["FINE", "FRENO ABILITA", "FRENO DISABILITA", "FRENO MARCIA ON", "FRENO MARCIA OFF", "FRENO SET RIF PARTENZA", "FRENO FORZA RIF FERMATA", "FRENO SET RIF FERMATA", "FRENO SET RIF A 0", "FRENO FORZA RIF A 0", "FRENO SET CONTROLLO COPPIA", "FRENO SET CONTROLLO VELOCITA'", "FRENO SET SENSO ROTAZIONE", "FRENO SET SENS ROT SEGNO COPPIA", "FRENO CONFIG", "ALIMENTATORE 1 ABILITA", "ALIMENTATORE 1 DISABILITA", "ALIMENTATORE 1 MARCIA ON", "ALIMENTATORE 1 MARCIA OFF", "ALIMENTATORE 1 SET RIF", "ALIMENTATORE 1 SET RIF RIDOTTO", "ALIMENTATORE 1 SET RIF A 0", "ALIMENTATORE 1 RESET ALLARMI", "ALIMENTATORE 1 SCORTA 2", "ALIMENTATORE 1 SCORTA 3", "ALIMENTATORE 2 ABILITA", "ALIMENTATORE 2 DISABILITA", "ALIMENTATORE 2 MARCIA ON", "ALIMENTATORE 2 MARCIA OFF", "ALIMENTATORE 2 SET RIF", "ALIMENTATORE 2 SET RIF RIDOTTO", "ALIMENTATORE 2 SET RIF A 0", "ALIMENTATORE 2 SCORTA 1", "ALIMENTATORE 2 SCORTA 2", "ALIMENTATORE 2 SCORTA 3", "TELERUTTORI CHIUDI POTENZA", "TELERUTTORI APRI POTENZA", "TELERUTTORI ABILITA POTENZA", "TELERUTTORI DISABILITA POTENZA", "TELERUTTORI MISURA RESISTENZA RESISTOMAT", "TELERUTTORI MISURA RESISTENZA RES METER", "PROCEDURA ROTORE BLOCCATO 1", "ATTENDI FERMATA MOTORE", "SEGNALA INIZIO AVVIO", "SEGNALA FINE AVVIO", "SEGNALA INIZIO FERMATA", "SEGNALA FINE FERMATA", "START PROFILO", "ATTENDI FINE RAMPA"] ("appended array")
  (unwired) T5[] [enum."ALIMENTATORE 1 MARCIA OFF", enum."FRENO MARCIA OFF", enum."ATTENDI FERMATA MOTORE", enum."FINE", enum."FINE"] items=["FINE", "FRENO ABILITA", "FRENO DISABILITA", "FRENO MARCIA ON", "FRENO MARCIA OFF", "FRENO SET RIF PARTENZA", "FRENO FORZA RIF FERMATA", "FRENO SET RIF FERMATA", "FRENO SET RIF A 0", "FRENO FORZA RIF A 0", "FRENO SET CONTROLLO COPPIA", "FRENO SET CONTROLLO VELOCITA'", "FRENO SET SENSO ROTAZIONE", "FRENO SET SENS ROT SEGNO COPPIA", "FRENO CONFIG", "ALIMENTATORE 1 ABILITA", "ALIMENTATORE 1 DISABILITA", "ALIMENTATORE 1 MARCIA ON", "ALIMENTATORE 1 MARCIA OFF", "ALIMENTATORE 1 SET RIF", "ALIMENTATORE 1 SET RIF RIDOTTO", "ALIMENTATORE 1 SET RIF A 0", "ALIMENTATORE 1 RESET ALLARMI", "ALIMENTATORE 1 SCORTA 2", "ALIMENTATORE 1 SCORTA 3", "ALIMENTATORE 2 ABILITA", "ALIMENTATORE 2 DISABILITA", "ALIMENTATORE 2 MARCIA ON", "ALIMENTATORE 2 MARCIA OFF", "ALIMENTATORE 2 SET RIF", "ALIMENTATORE 2 SET RIF RIDOTTO", "ALIMENTATORE 2 SET RIF A 0", "ALIMENTATORE 2 SCORTA 1", "ALIMENTATORE 2 SCORTA 2", "ALIMENTATORE 2 SCORTA 3", "TELERUTTORI CHIUDI POTENZA", "TELERUTTORI APRI POTENZA", "TELERUTTORI ABILITA POTENZA", "TELERUTTORI DISABILITA POTENZA", "TELERUTTORI MISURA RESISTENZA RESISTOMAT", "TELERUTTORI MISURA RESISTENZA RES METER", "PROCEDURA ROTORE BLOCCATO 1", "ATTENDI FERMATA MOTORE", "SEGNALA INIZIO AVVIO", "SEGNALA FINE AVVIO", "SEGNALA INIZIO FERMATA", "SEGNALA FINE FERMATA", "START PROFILO", "ATTENDI FINE RAMPA"] ("appended array")
  w1 = FALSE ("AVVISO AVVIO IN CORSO")
  # "SACCARDO\nMODIFICATA PROCEDURA STOP AUTOMATICO\nper velocizzare la procedura di stop, bypasso le rampe dei\nriferimenti coppia e velocità (variabile globale \"Forza rif\")\ne forzo le uscite dei riferimenti direttamente da qui nei cases\n\"FRENO FORZA RIF FERMATA\", \"FRENO FORZA RIF A 0\""
  # "CASES PRINCIPALI:\n\n-TELERUTTORI ABILITA POTENZA\n-TELERUTTORI DISABILITA POTENZA\n-TELERUTTORI CHIUDI POTENZA\n-TELERUTTORI APRI POTENZA\n-TELERUTTORI MISURA RESISTENZA RESISTOMAT"
  n1 = Obtain Queue(name (unnamed)="PROCEDURE", element data type=T8 {"Message"="", "Message Data"=variant} ("Message Cluster")) -> (queue out=w5:refnum<queue>, error out=w3:errorcluster)  [unwired: 3 in, 1 out]
  n2 = Flush Queue(queue=w5, error in (no error)=w3) -> (queue out=w4:refnum<queue>, error out=w2:errorcluster)  [unwired: 1 out]
  n3 = Enqueue Element(queue=w4, element=cluster{"Status":string, "variant":variant} {"Status"="IDLE", "variant"=variant}, error in (no error)=w2) -> (queue out=w7:refnum<queue>, error out=w8:errorcluster)  [unwired: 1 in, 1 out]
  n4 = while {
    shift-right: [w26] -> _
    shift-left: _ -> [w25]
    tunnel: w7 -> [w38]
    tunnel: w8 -> [w37]
    shift-right: [w33] -> _
    shift-left: _ -> [w34]
    shift-right: [w30] -> _
    shift-left: _ -> [w29]
    shift-right: [w28] -> _
    shift-left: TRUE -> [w27]
    shift-right: [w20] -> _
    shift-left: _ -> [w21]
    shift-right: [w19] -> _
    shift-left: _ -> [w18]
    shift-right: [w17] -> _
    shift-left: _ -> [w16]
    stop <- w32 stop-if-true
    n5 = global read "Stato comandi freno.vi" "Stato inverter"() -> (w24:T25)
    n6 = Dequeue Element(queue=w38, error in (no error)=w37) -> (queue out=w14:refnum<queue>, element=w36:T8)  [unwired: 1 in, 2 out]
    n7 = global read "Stato alimentatore 1.vi" "Stato alimentatore 1"() -> (w22:T28)
    n8 = Unbundle By Name(w24) -> ("Stato comandi freno"=w15:T26, "Stato"=w23:T29)
    n9 = Unbundle By Name(w36) -> ("Message"=w31:string, "Message Data"=w35:variant)
    "Message" <- w31
    n10 = Get Queue Status(queue=w14) -> (elements=→"Elements In Queue":T1)  [unwired: 2 in, 7 out]
    n11 = Wait (ms)(milliseconds to wait=u32 100) -> ()  [unwired: 1 out]
    n12 = case shown="\"ESEGUI\"" w31 {
      tunnel: w31 -> [_ _ _ _ _ _ _]
      tunnel: w35 -> [_ w70 _ _ _ _ w1634]
      tunnel: w34 -> [w46 w71 w479 w486 w501 w509 w1631]
      tunnel: [w46 w69 w479 w486 w504 w508 w1631] -> w33
      tunnel: [_ _ _ w481 _ _ _] -> w32
      tunnel: [w45 w47 w478 w485 w502 w532 w1630] -> w30
      tunnel: w29 -> [w45 w50 w478 w485 _ w533 w1630]
      tunnel: w14 -> [_ w49 _ _ w500 w531 _]
      tunnel: [TRUE _ _ _ _ w529 w1628] -> w28
      tunnel: w27 -> [_ w68 _ _ _ _ w1628]
      tunnel: [w44 w63 w477 w484 w496 w528 w1632] -> w26
      tunnel: w25 -> [w44 w62 w477 w484 w496 w528 w1632]
      tunnel: w15 -> [_ w57 _ _ _ w527 _]
      tunnel: w23 -> [_ w54 _ _ _ w525 _]
      tunnel: w22 -> [_ w56 _ _ _ w524 _]
      tunnel: w21 -> [w43 w51 w476 w483 w495 w523 w1629]
      tunnel: [w43 w60 w476 w483 w494 w523 w1629] -> w20
      tunnel: [w42 w59 w475 w482 w489 w520 w1635] -> w19
      tunnel: w18 -> [w42 w58 w475 w482 w489 w520 w1635]
      tunnel: [w40 w53 w474 w480 w487 w510 w1627] -> w17
      tunnel: w16 -> [w40 w53 w474 w480 w487 w510 _]
      frame "IDLE", Default {
        n13 = local write "Stato"("Default" ("Stato")) -> ()
      }
      frame "AGGIUNGI PROCEDURA" {
        n14 = Variant To Data(type=cluster{"PROCEDURE":T4, "Variant":variant} {"PROCEDURE"=enum."START", "Variant"=variant}, Variant=w70) -> (data=w65:cluster{"PROCEDURE":T4, "Variant":variant})  [unwired: 1 in, 1 out]
        n15 = disable-structure shown="Disabled" {
          frame Disabled {
            n16 = global read "Global_All_Data.vi" "All Data"() -> ()  [unwired: 1 out]
          }
          frame Enabled {
          }
        }
        n17 = Unbundle By Name(w65) -> ("PROCEDURE"=w61:T4, "Variant"=w64:variant)
        n18 = case shown="\"START\"" w61 {
          tunnel: w71 -> [w95 w301 w333 w341 w347 w358 w363 w381 w390 w398 _ w420 w434 w444 w452 w462 _]
          tunnel: [w96 w302 w332 w340 w346 w357 w362 w380 w389 w397 w409 w428 w438 w445 w454 w466 _] -> w69
          tunnel: [_ w286 _ _ _ _ _ _ _ _ w411 _ _ _ _ _ _] -> w48
          tunnel: w64 -> [w91 _ _ w342 _ w355 w367 w376 _ _ _ _ _ _ _ w464 _]
          tunnel: [w90 w300 w334 w343 w350 w360 w370 w385 w394 w403 w416 w432 w442 w450 w459 w471 w473] -> w63
          tunnel: w62 -> [_ w300 w334 w343 w350 w360 w370 w385 w394 w403 w416 w432 w442 w450 w459 w471 w473]
          tunnel: [w87 w299 w330 w338 w349 w356 w369 w384 w393 w402 w415 w431 w441 w449 w458 w470 w472] -> w59
          tunnel: w58 -> [w87 w299 w330 _ w349 w356 w369 w384 w393 w402 w415 w431 w441 w449 w458 w470 w472]
          tunnel: w57 -> [_ _ _ _ _ _ _ _ _ _ _ _ _ _ _ _ _]
          tunnel: w56 -> [_ _ _ _ _ _ _ _ _ _ _ _ _ _ _ _ _]
          tunnel: ["START" "STOP AUTOMATICO SISTEMA..." "STOP FRENO..." "ABILITAZIONE POTENZA..." "DISABILITAZIONE POTENZA..." "MISURA RESISTENZA RESISTOMAT..." "MISURA RESISTENZA RES METER..." _ "CHIUSURA TELERUTTORI POTENZA..." "APERTURA TELERUTTORI POTENZA..." "--ALLARME--" _ _ _ "START PROFILO" "CONFIG FRENO" _] -> w55
          tunnel: w54 -> [_ _ _ _ _ _ _ _ _ _ _ _ _ _ _ _ _]
          tunnel: w50 -> [w81 w287 w328 w335 w344 w351 w361 w371 w386 w395 w404 w419 w433 w443 w451 w460 _]
          tunnel: [w81 w287 w328 w335 w344 w351 w361 w371 w386 w395 w404 w419 w433 w443 w451 w460 _] -> w47
          frame "START" {
            n19 = global write "Global FINE AVVIO.vi" "AVVISO AVVIO IN CORSO"(TRUE ("AVVISO AVVIO IN CORSO")) -> ()
            n20 = Variant To Data(type=T7 {"MODALITA' BANCO"=enum."SOLO FRENO", "MODALITA' AVVIO MOTORE"=enum."AVVIO DIRETTO DA LINEA", "MODALITA' AVVIO FRENO"=enum."MARCIA DOPO AVVIO MOTORE", "V avvio[V]"=0.0, "F avvio[Hz]"=0.0, "%V ridotta"=0.0, "C avvio [Nm]"=0.0, "RPM avvio"=0.0, "SERVO AVVIO"=FALSE, "SENSO DI ROTAZIONE"=FALSE} ("Modalità avvio"), Variant=w91) -> (data=w90:T7)  [unwired: 1 in, 1 out]
            n21 = Unbundle By Name(w90) -> ("SERVO AVVIO"=w89:bool, "MODALITA' BANCO"=w94:T30, "MODALITA' AVVIO MOTORE"=w93:T31, "MODALITA' AVVIO FRENO"=w92:T32)
            n22 = global write "Global prova in corso.vi" "prova in corso?"(TRUE ("prova in corso?")) -> ()
            n23 = global write "Global_bypass_ResMeter.vi" "Bypass res meter"(TRUE ("Bypass res meter")) -> ()
            n24 = global write "Global FINE AVVIO.vi" "FINE AVVIO"(FALSE ("FINE AVVIO")) -> ()
            n25 = global write "Global Trampa 0.vi" "Forza rif"(FALSE ("Rampa a 0")) -> ()
            n26 = case shown="\"ALIMENTATORE E FRENO\", Default" w94 {
              tunnel: w93 -> [w101 w254 _ _ _]
              tunnel: w92 -> [w100 _ _ _ _]
              tunnel: [w99 w253 w282 w283 w284] -> w97
              tunnel: w89 -> [w98 _ _ _ _]
              frame "ALIMENTATORE E FRENO", Default {
                n27 = case shown="\"MARCIA DOPO AVVIO MOTORE\", Default" w100 {
                  tunnel: w101 -> [w116 w198]
                  tunnel: [w115 w196] -> w99
                  tunnel: w98 -> [w113 w189]
                  frame "MARCIA DOPO AVVIO MOTORE", Default {
                    # "AVVIO A FRENO NON IN MARCIA"
                    n28 = case shown="\"AVVIO DIRETTO DA ALIM\"" w116 {
                      tunnel: [Operazioni."ALIMENTATORE 1 SET RIF RIDOTTO" ("OPERAZIONI") Operazioni."ALIMENTATORE 1 SET RIF A 0" ("OPERAZIONI") Operazioni."ALIMENTATORE 1 SET RIF" ("OPERAZIONI") w181] -> w120
                      tunnel: [Operazioni."ALIMENTATORE 1 MARCIA ON" ("OPERAZIONI") Operazioni."ALIMENTATORE 1 MARCIA ON" ("OPERAZIONI") Operazioni."ALIMENTATORE 1 MARCIA ON" ("OPERAZIONI") w180] -> w119
                      tunnel: [Operazioni."ALIMENTATORE 1 SET RIF" ("OPERAZIONI") Operazioni."ALIMENTATORE 1 SET RIF" ("OPERAZIONI") Operazioni."FRENO SET CONTROLLO COPPIA" ("OPERAZIONI") w179] -> w118
                      tunnel: [Operazioni."FRENO SET CONTROLLO COPPIA" ("OPERAZIONI") Operazioni."FRENO SET CONTROLLO COPPIA" ("OPERAZIONI") Operazioni."FRENO SET RIF A 0" ("OPERAZIONI") w178] -> w117
                      tunnel: [Operazioni."FRENO MARCIA ON" ("OPERAZIONI") Operazioni."FRENO MARCIA ON" ("OPERAZIONI") Operazioni."SEGNALA FINE AVVIO" ("OPERAZIONI") w176] -> w114
                      tunnel: [Operazioni."SEGNALA FINE AVVIO" ("OPERAZIONI") Operazioni."SEGNALA FINE AVVIO" ("OPERAZIONI") w169 w176] -> w108
                      tunnel: [Operazioni."ALIMENTATORE 1 ABILITA" ("OPERAZIONI") Operazioni."ALIMENTATORE 1 ABILITA" ("OPERAZIONI") Operazioni."ALIMENTATORE 1 ABILITA" ("OPERAZIONI") w177] -> w107
                      tunnel: [Operazioni."FINE" ("OPERAZIONI") Operazioni."FINE" ("OPERAZIONI") w169 w176] -> w105
                      tunnel: [Operazioni."FRENO SET RIF A 0" ("OPERAZIONI") Operazioni."FRENO SET RIF A 0" ("OPERAZIONI") Operazioni."FRENO MARCIA ON" ("OPERAZIONI") w176] -> w104
                      tunnel: [_ _ Operazioni."ATTENDI FINE RAMPA" ("OPERAZIONI") w175] -> w102
                      frame "AVVIO A TENSIONE RIDOTTA", Default {
                      }
                      frame "AVVIO IN RAMPA" {
                      }
                      frame "AVVIO DIRETTO DA ALIM" {
                        w169 = Operazioni."FINE" ("OPERAZIONI")
                      }
                      frame "AVVIO DIRETTO DA LINEA" {
                        n29 = disable-structure shown="Disabled" {
                          disable-tunnel: [Operazioni."TELERUTTORI CHIUDI POTENZA" ("OPERAZIONI") _] -> w181
                          disable-tunnel: [Operazioni."FRENO SET CONTROLLO COPPIA" ("OPERAZIONI") _] -> w180
                          disable-tunnel: [Operazioni."FRENO SET RIF A 0" ("OPERAZIONI") _] -> w179
                          disable-tunnel: [Operazioni."FRENO MARCIA ON" ("OPERAZIONI") _] -> w178
                          disable-tunnel: [Operazioni."ALIMENTATORE 1 ABILITA" ("OPERAZIONI") _] -> w177
                          disable-tunnel: [Operazioni."FINE" ("OPERAZIONI") _] -> w176
                          disable-tunnel: [Operazioni."SEGNALA FINE AVVIO" ("OPERAZIONI") _] -> w175
                          frame Disabled {
                            (unwired) Operazioni."FRENO SET SENS ROT SEGNO COPPIA" ("OPERAZIONI")
                          }
                          frame Enabled {
                          }
                        }
                      }
                    }
                    n30 = case shown="False" w113 {
                      tunnel: w120 -> [w130 w147]
                      tunnel: w119 -> [w131 w146]
                      tunnel: w118 -> [w132 w145]
                      tunnel: w117 -> [w133 w144]
                      tunnel: [w129 w143] -> w115
                      tunnel: w114 -> [w122 w136]
                      tunnel: Operazioni."FRENO MARCIA ON" ("OPERAZIONI") -> [_ w142]
                      tunnel: Operazioni."FRENO SET CONTROLLO VELOCITA'" ("OPERAZIONI") -> [_ w141]
                      tunnel: Operazioni."FRENO SET SENSO ROTAZIONE" ("OPERAZIONI") -> [_ w140]
                      tunnel: Operazioni."FRENO SET RIF A 0" ("OPERAZIONI") -> [_ w139]
                      tunnel: w108 -> [w123 w135]
                      tunnel: w107 -> [w128 w138]
                      tunnel: Operazioni."FRENO ABILITA" ("OPERAZIONI") -> [w125 w137]
                      tunnel: w105 -> [w124 _]
                      tunnel: w104 -> [w127 _]
                      tunnel: Operazioni."SEGNALA INIZIO AVVIO" ("OPERAZIONI") -> [w126 w134]
                      tunnel: w102 -> [w121 _]
                      frame False {
                        n31 = Build Array(w126, w125, w128, w130, w131, w132, w133, w127, w121, w122, w123, w124) -> (w129:T5[])
                      }
                      frame True {
                        n32 = Build Array(w134, w137, w139, w140, w141, w142, w138, w147, w146, w145, w144, w136, w135) -> (w143:T5[])
                      }
                    }
                  }
                  frame "MARCIA PRIMA AVVIO" {
                    # "AVVIO CON FRENO \nIN MARCIA"
                    n33 = case shown="\"AVVIO A TENSIONE RIDOTTA\", Default" w198 {
                      tunnel: [Operazioni."ALIMENTATORE 1 SET RIF RIDOTTO" ("OPERAZIONI") Operazioni."ALIMENTATORE 1 SET RIF A 0" ("OPERAZIONI") Operazioni."ALIMENTATORE 1 SET RIF" ("OPERAZIONI") w244] -> w193
                      tunnel: [Operazioni."ALIMENTATORE 1 MARCIA ON" ("OPERAZIONI") Operazioni."ALIMENTATORE 1 MARCIA ON" ("OPERAZIONI") Operazioni."ALIMENTATORE 1 MARCIA ON" ("OPERAZIONI") w245] -> w197
                      tunnel: [Operazioni."ALIMENTATORE 1 SET RIF" ("OPERAZIONI") Operazioni."ALIMENTATORE 1 SET RIF" ("OPERAZIONI") Operazioni."SEGNALA FINE AVVIO" ("OPERAZIONI") w245] -> w195
                      tunnel: [Operazioni."SEGNALA FINE AVVIO" ("OPERAZIONI") Operazioni."SEGNALA FINE AVVIO" ("OPERAZIONI") w239 w245] -> w194
                      tunnel: [w227 w233 w239 w245] -> w191
                      tunnel: [Operazioni."ALIMENTATORE 1 ABILITA" ("OPERAZIONI") Operazioni."ALIMENTATORE 1 ABILITA" ("OPERAZIONI") Operazioni."ALIMENTATORE 1 ABILITA" ("OPERAZIONI") w246] -> w192
                      tunnel: [w227 w233 w239 w245] -> w190
                      frame "AVVIO A TENSIONE RIDOTTA", Default {
                        w227 = Operazioni."FINE" ("OPERAZIONI")
                      }
                      frame "AVVIO IN RAMPA" {
                        w233 = Operazioni."FINE" ("OPERAZIONI")
                      }
                      frame "AVVIO DIRETTO DA ALIM" {
                        w239 = Operazioni."FINE" ("OPERAZIONI")
                      }
                      frame "AVVIO DIRETTO DA LINEA" {
                        n34 = disable-structure shown="Enabled" {
                          disable-tunnel: [Operazioni."TELERUTTORI CHIUDI POTENZA" ("OPERAZIONI") _] -> w246
                          disable-tunnel: [Operazioni."FINE" ("OPERAZIONI") _] -> w245
                          disable-tunnel: [Operazioni."SEGNALA FINE AVVIO" ("OPERAZIONI") _] -> w244
                          frame Disabled {
                          }
                          frame Enabled {
                          }
                        }
                      }
                    }
                    n35 = case shown="False" w189 {
                      tunnel: w197 -> [w211 w226]
                      tunnel: [w210 w224] -> w196
                      tunnel: w195 -> [w209 w215]
                      tunnel: w194 -> [w208 w214]
                      tunnel: w193 -> [w207 w225]
                      tunnel: w192 -> [w206 w218]
                      tunnel: w191 -> [w205 w212]
                      tunnel: w190 -> [w204 w213]
                      frame False {
                        # "CASE DI DEFAULT"
                        n36 = Build Array(Operazioni."FRENO SET CONTROLLO COPPIA" ("OPERAZIONI"), Operazioni."FRENO SET SENSO ROTAZIONE" ("OPERAZIONI"), Operazioni."FRENO ABILITA" ("OPERAZIONI"), Operazioni."FRENO SET RIF PARTENZA" ("OPERAZIONI"), Operazioni."FRENO MARCIA ON" ("OPERAZIONI"), w206, w207, w211, w209, w208, w204, w205) -> (w210:T5[])
                      }
                      frame True {
                        n37 = Build Array(Operazioni."FRENO SET CONTROLLO COPPIA" ("OPERAZIONI"), Operazioni."FRENO SET SENSO ROTAZIONE" ("OPERAZIONI"), Operazioni."FRENO ABILITA" ("OPERAZIONI"), Operazioni."FRENO SET RIF A 0" ("OPERAZIONI"), Operazioni."FRENO MARCIA ON" ("OPERAZIONI"), Operazioni."FRENO SET CONTROLLO VELOCITA'" ("OPERAZIONI"), Operazioni."FRENO SET RIF PARTENZA" ("OPERAZIONI"), w218, w225, w226, w215, w214, w213, w212) -> (w224:T5[])
                      }
                    }
                  }
                }
              }
              frame "SOLO ALIMENTATORE" {
                n38 = case shown="\"AVVIO A TENSIONE RIDOTTA\", Default" w254 {
                  tunnel: [Operazioni."ALIMENTATORE 1 SET RIF RIDOTTO" ("OPERAZIONI") Operazioni."ALIMENTATORE 1 SET RIF A 0" ("OPERAZIONI") Operazioni."ALIMENTATORE 1 SET RIF" ("OPERAZIONI") w276] -> w258
                  tunnel: [Operazioni."ALIMENTATORE 1 MARCIA ON" ("OPERAZIONI") Operazioni."ALIMENTATORE 1 MARCIA ON" ("OPERAZIONI") Operazioni."ALIMENTATORE 1 MARCIA ON" ("OPERAZIONI") w277] -> w257
                  tunnel: [Operazioni."ALIMENTATORE 1 SET RIF" ("OPERAZIONI") Operazioni."ALIMENTATORE 1 SET RIF" ("OPERAZIONI") Operazioni."SEGNALA FINE AVVIO" ("OPERAZIONI") w277] -> w256
                  tunnel: [Operazioni."SEGNALA FINE AVVIO" ("OPERAZIONI") Operazioni."SEGNALA FINE AVVIO" ("OPERAZIONI") w271 w277] -> w255
                  tunnel: [w259 w265 w271 w277] -> w251
                  tunnel: [Operazioni."ALIMENTATORE 1 ABILITA" ("OPERAZIONI") Operazioni."ALIMENTATORE 1 ABILITA" ("OPERAZIONI") Operazioni."ALIMENTATORE 1 ABILITA" ("OPERAZIONI") w278] -> w252
                  tunnel: [w259 w265 w271 w277] -> w250
                  frame "AVVIO A TENSIONE RIDOTTA", Default {
                    w259 = Operazioni."FINE" ("OPERAZIONI")
                  }
                  frame "AVVIO IN RAMPA" {
                    w265 = Operazioni."FINE" ("OPERAZIONI")
                  }
                  frame "AVVIO DIRETTO DA ALIM" {
                    w271 = Operazioni."FINE" ("OPERAZIONI")
                  }
                  frame "AVVIO DIRETTO DA LINEA" {
                    n39 = disable-structure shown="Disabled" {
                      disable-tunnel: [Operazioni."TELERUTTORI CHIUDI POTENZA" ("OPERAZIONI") _] -> w278
                      disable-tunnel: [Operazioni."FINE" ("OPERAZIONI") _] -> w277
                      disable-tunnel: [Operazioni."SEGNALA FINE AVVIO" ("OPERAZIONI") _] -> w276
                      frame Disabled {
                      }
                      frame Enabled {
                      }
                    }
                  }
                }
                n40 = Build Array(w252, w258, w257, w256, w255, w250, w251) -> (w253:T5[])
              }
              frame "SOLO FRENO" {
                w282 = T5[] [enum."FRENO ABILITA", enum."FRENO SET RIF A 0", enum."FRENO SET CONTROLLO COPPIA", enum."FRENO SET RIF PARTENZA", enum."FRENO MARCIA ON", enum."SEGNALA FINE AVVIO", enum."FINE"] items=["FINE", "FRENO ABILITA", "FRENO DISABILITA", "FRENO MARCIA ON", "FRENO MARCIA OFF", "FRENO SET RIF PARTENZA", "FRENO FORZA RIF FERMATA", "FRENO SET RIF FERMATA", "FRENO SET RIF A 0", "FRENO FORZA RIF A 0", "FRENO SET CONTROLLO COPPIA", "FRENO SET CONTROLLO VELOCITA'", "FRENO SET SENSO ROTAZIONE", "FRENO SET SENS ROT SEGNO COPPIA", "FRENO CONFIG", "ALIMENTATORE 1 ABILITA", "ALIMENTATORE 1 DISABILITA", "ALIMENTATORE 1 MARCIA ON", "ALIMENTATORE 1 MARCIA OFF", "ALIMENTATORE 1 SET RIF", "ALIMENTATORE 1 SET RIF RIDOTTO", "ALIMENTATORE 1 SET RIF A 0", "ALIMENTATORE 1 RESET ALLARMI", "ALIMENTATORE 1 SCORTA 2", "ALIMENTATORE 1 SCORTA 3", "ALIMENTATORE 2 ABILITA", "ALIMENTATORE 2 DISABILITA", "ALIMENTATORE 2 MARCIA ON", "ALIMENTATORE 2 MARCIA OFF", "ALIMENTATORE 2 SET RIF", "ALIMENTATORE 2 SET RIF RIDOTTO", "ALIMENTATORE 2 SET RIF A 0", "ALIMENTATORE 2 SCORTA 1", "ALIMENTATORE 2 SCORTA 2", "ALIMENTATORE 2 SCORTA 3", "TELERUTTORI CHIUDI POTENZA", "TELERUTTORI APRI POTENZA", "TELERUTTORI ABILITA POTENZA", "TELERUTTORI DISABILITA POTENZA", "TELERUTTORI MISURA RESISTENZA RESISTOMAT", "TELERUTTORI MISURA RESISTENZA RES METER", "PROCEDURA ROTORE BLOCCATO 1", "ATTENDI FERMATA MOTORE", "SEGNALA INIZIO AVVIO", "SEGNALA FINE AVVIO", "SEGNALA INIZIO FERMATA", "SEGNALA FINE FERMATA", "START PROFILO", "ATTENDI FINE RAMPA"] ("appended array")
              }
              frame "SOLO ACQUISITORE" {
                w283 = T5[] [enum."FINE"] items=["FINE", "FRENO ABILITA", "FRENO DISABILITA", "FRENO MARCIA ON", "FRENO MARCIA OFF", "FRENO SET RIF PARTENZA", "FRENO FORZA RIF FERMATA", "FRENO SET RIF FERMATA", "FRENO SET RIF A 0", "FRENO FORZA RIF A 0", "FRENO SET CONTROLLO COPPIA", "FRENO SET CONTROLLO VELOCITA'", "FRENO SET SENSO ROTAZIONE", "FRENO SET SENS ROT SEGNO COPPIA", "FRENO CONFIG", "ALIMENTATORE 1 ABILITA", "ALIMENTATORE 1 DISABILITA", "ALIMENTATORE 1 MARCIA ON", "ALIMENTATORE 1 MARCIA OFF", "ALIMENTATORE 1 SET RIF", "ALIMENTATORE 1 SET RIF RIDOTTO", "ALIMENTATORE 1 SET RIF A 0", "ALIMENTATORE 1 RESET ALLARMI", "ALIMENTATORE 1 SCORTA 2", "ALIMENTATORE 1 SCORTA 3", "ALIMENTATORE 2 ABILITA", "ALIMENTATORE 2 DISABILITA", "ALIMENTATORE 2 MARCIA ON", "ALIMENTATORE 2 MARCIA OFF", "ALIMENTATORE 2 SET RIF", "ALIMENTATORE 2 SET RIF RIDOTTO", "ALIMENTATORE 2 SET RIF A 0", "ALIMENTATORE 2 SCORTA 1", "ALIMENTATORE 2 SCORTA 2", "ALIMENTATORE 2 SCORTA 3", "TELERUTTORI CHIUDI POTENZA", "TELERUTTORI APRI POTENZA", "TELERUTTORI ABILITA POTENZA", "TELERUTTORI DISABILITA POTENZA", "TELERUTTORI MISURA RESISTENZA RESISTOMAT", "TELERUTTORI MISURA RESISTENZA RES METER", "PROCEDURA ROTORE BLOCCATO 1", "ATTENDI FERMATA MOTORE", "SEGNALA INIZIO AVVIO", "SEGNALA FINE AVVIO", "SEGNALA INIZIO FERMATA", "SEGNALA FINE FERMATA", "START PROFILO", "ATTENDI FINE RAMPA"] ("appended array")
                # "SOLO ACQUISITORE\nNESSUNA PROCEDURA DI START"
              }
              frame "GESTIONE MANUALE" {
                w284 = T5[] [enum."FINE"] items=["FINE", "FRENO ABILITA", "FRENO DISABILITA", "FRENO MARCIA ON", "FRENO MARCIA OFF", "FRENO SET RIF PARTENZA", "FRENO FORZA RIF FERMATA", "FRENO SET RIF FERMATA", "FRENO SET RIF A 0", "FRENO FORZA RIF A 0", "FRENO SET CONTROLLO COPPIA", "FRENO SET CONTROLLO VELOCITA'", "FRENO SET SENSO ROTAZIONE", "FRENO SET SENS ROT SEGNO COPPIA", "FRENO CONFIG", "ALIMENTATORE 1 ABILITA", "ALIMENTATORE 1 DISABILITA", "ALIMENTATORE 1 MARCIA ON", "ALIMENTATORE 1 MARCIA OFF", "ALIMENTATORE 1 SET RIF", "ALIMENTATORE 1 SET RIF RIDOTTO", "ALIMENTATORE 1 SET RIF A 0", "ALIMENTATORE 1 RESET ALLARMI", "ALIMENTATORE 1 SCORTA 2", "ALIMENTATORE 1 SCORTA 3", "ALIMENTATORE 2 ABILITA", "ALIMENTATORE 2 DISABILITA", "ALIMENTATORE 2 MARCIA ON", "ALIMENTATORE 2 MARCIA OFF", "ALIMENTATORE 2 SET RIF", "ALIMENTATORE 2 SET RIF RIDOTTO", "ALIMENTATORE 2 SET RIF A 0", "ALIMENTATORE 2 SCORTA 1", "ALIMENTATORE 2 SCORTA 2", "ALIMENTATORE 2 SCORTA 3", "TELERUTTORI CHIUDI POTENZA", "TELERUTTORI APRI POTENZA", "TELERUTTORI ABILITA POTENZA", "TELERUTTORI DISABILITA POTENZA", "TELERUTTORI MISURA RESISTENZA RESISTOMAT", "TELERUTTORI MISURA RESISTENZA RES METER", "PROCEDURA ROTORE BLOCCATO 1", "ATTENDI FERMATA MOTORE", "SEGNALA INIZIO AVVIO", "SEGNALA FINE AVVIO", "SEGNALA INIZIO FERMATA", "SEGNALA FINE FERMATA", "START PROFILO", "ATTENDI FINE RAMPA"]
              }
            }
            n41 = Build Array (concatenate)(w95, w97) -> (w96:T5[][])
          }
          frame "STOP AUTOMATICO", Default {
            w286 = TRUE  # Priorità
            # "STOP GENERICO"
            n42 = global read "Stato comandi freno.vi" "Stato inverter"() -> (w289:T25)
            n43 = global read "Stato alimentatore 1.vi" "Stato alimentatore 1"() -> (w290:T28)
            n44 = Unbundle By Name(w289) -> ("Stato.Controllo effettivo"=w285:T16, "Stato.Start"=w296:bool)
            n45 = flat-sequence {
              tunnel: [w304] -> w288
              frame #0 {
                n46 = global read "Global stato profilo.vi" "STATO PROFILO"() -> (w305:T33)
                n47 = Unbundle By Name(w305) -> ("IN ESECUZIONE"=w303:bool)
                n48 = case shown="True" w303 {
                  tunnel: [_ w306] -> w304
                  frame False {
                  }
                  frame True {
                    n49 = Obtain Queue(name (unnamed)="GESTORE PROFILI", element data type=T8 {"Message"="", "Message Data"=variant} ("Message Cluster")) -> (queue out=w309:refnum<queue>, error out=w308:errorcluster)  [unwired: 3 in, 1 out]
                    n50 = Enqueue Element(queue=w309, element=cluster{"Status":string, "variant":variant} {"Status"="PAUSA PROFILO", "variant"=variant}, error in (no error)=w308) -> (error out=w306:errorcluster)  [unwired: 1 in, 2 out]
                  }
                }
              }
            }
            n51 = Unbundle By Name(w290) -> ("In marcia"=w295:bool)
            n52 = Build Array(w296, w295) -> (w294:bool[])
            n53 = Boolean Array To Number(Boolean array=w294) -> (number=w293:u32)
            n54 = case shown="3" w293 {
              tunnel: [w312 w313 w314 w316] -> w292
              tunnel: w288 -> [_ _ _ _]
              tunnel: w285 -> [_ _ _ w315]
              frame 0, Default {
                w312 = T5[] [enum."SEGNALA INIZIO FERMATA", enum."ALIMENTATORE 1 MARCIA OFF", enum."FRENO MARCIA OFF", enum."SEGNALA FINE FERMATA", enum."FINE"] items=["FINE", "FRENO ABILITA", "FRENO DISABILITA", "FRENO MARCIA ON", "FRENO MARCIA OFF", "FRENO SET RIF PARTENZA", "FRENO FORZA RIF FERMATA", "FRENO SET RIF FERMATA", "FRENO SET RIF A 0", "FRENO FORZA RIF A 0", "FRENO SET CONTROLLO COPPIA", "FRENO SET CONTROLLO VELOCITA'", "FRENO SET SENSO ROTAZIONE", "FRENO SET SENS ROT SEGNO COPPIA", "FRENO CONFIG", "ALIMENTATORE 1 ABILITA", "ALIMENTATORE 1 DISABILITA", "ALIMENTATORE 1 MARCIA ON", "ALIMENTATORE 1 MARCIA OFF", "ALIMENTATORE 1 SET RIF", "ALIMENTATORE 1 SET RIF RIDOTTO", "ALIMENTATORE 1 SET RIF A 0", "ALIMENTATORE 1 RESET ALLARMI", "ALIMENTATORE 1 SCORTA 2", "ALIMENTATORE 1 SCORTA 3", "ALIMENTATORE 2 ABILITA", "ALIMENTATORE 2 DISABILITA", "ALIMENTATORE 2 MARCIA ON", "ALIMENTATORE 2 MARCIA OFF", "ALIMENTATORE 2 SET RIF", "ALIMENTATORE 2 SET RIF RIDOTTO", "ALIMENTATORE 2 SET RIF A 0", "ALIMENTATORE 2 SCORTA 1", "ALIMENTATORE 2 SCORTA 2", "ALIMENTATORE 2 SCORTA 3", "TELERUTTORI CHIUDI POTENZA", "TELERUTTORI APRI POTENZA", "TELERUTTORI ABILITA POTENZA", "TELERUTTORI DISABILITA POTENZA", "TELERUTTORI MISURA RESISTENZA RESISTOMAT", "TELERUTTORI MISURA RESISTENZA RES METER", "PROCEDURA ROTORE BLOCCATO 1", "ATTENDI FERMATA MOTORE", "SEGNALA INIZIO AVVIO", "SEGNALA FINE AVVIO", "SEGNALA INIZIO FERMATA", "SEGNALA FINE FERMATA", "START PROFILO", "ATTENDI FINE RAMPA"] ("appended array")
                # "nessuno in marcia"
              }
              frame 1 {
                w313 = T5[] [enum."SEGNALA INIZIO FERMATA", enum."FRENO SET CONTROLLO COPPIA", enum."FRENO SET RIF FERMATA", enum."ATTENDI FERMATA MOTORE", enum."FRENO MARCIA OFF", enum."ATTENDI FERMATA MOTORE", enum."SEGNALA FINE FERMATA", enum."FRENO SET RIF A 0", enum."FINE"] items=["FINE", "FRENO ABILITA", "FRENO DISABILITA", "FRENO MARCIA ON", "FRENO MARCIA OFF", "FRENO SET RIF PARTENZA", "FRENO FORZA RIF FERMATA", "FRENO SET RIF FERMATA", "FRENO SET RIF A 0", "FRENO FORZA RIF A 0", "FRENO SET CONTROLLO COPPIA", "FRENO SET CONTROLLO VELOCITA'", "FRENO SET SENSO ROTAZIONE", "FRENO SET SENS ROT SEGNO COPPIA", "FRENO CONFIG", "ALIMENTATORE 1 ABILITA", "ALIMENTATORE 1 DISABILITA", "ALIMENTATORE 1 MARCIA ON", "ALIMENTATORE 1 MARCIA OFF", "ALIMENTATORE 1 SET RIF", "ALIMENTATORE 1 SET RIF RIDOTTO", "ALIMENTATORE 1 SET RIF A 0", "ALIMENTATORE 1 RESET ALLARMI", "ALIMENTATORE 1 SCORTA 2", "ALIMENTATORE 1 SCORTA 3", "ALIMENTATORE 2 ABILITA", "ALIMENTATORE 2 DISABILITA", "ALIMENTATORE 2 MARCIA ON", "ALIMENTATORE 2 MARCIA OFF", "ALIMENTATORE 2 SET RIF", "ALIMENTATORE 2 SET RIF RIDOTTO", "ALIMENTATORE 2 SET RIF A 0", "ALIMENTATORE 2 SCORTA 1", "ALIMENTATORE 2 SCORTA 2", "ALIMENTATORE 2 SCORTA 3", "TELERUTTORI CHIUDI POTENZA", "TELERUTTORI APRI POTENZA", "TELERUTTORI ABILITA POTENZA", "TELERUTTORI DISABILITA POTENZA", "TELERUTTORI MISURA RESISTENZA RESISTOMAT", "TELERUTTORI MISURA RESISTENZA RES METER", "PROCEDURA ROTORE BLOCCATO 1", "ATTENDI FERMATA MOTORE", "SEGNALA INIZIO AVVIO", "SEGNALA FINE AVVIO", "SEGNALA INIZIO FERMATA", "SEGNALA FINE FERMATA", "START PROFILO", "ATTENDI FINE RAMPA"] ("appended array")
                # "solo freno in marcia"
              }
              frame 2 {
                w314 = T5[] [enum."SEGNALA INIZIO FERMATA", enum."ALIMENTATORE 1 MARCIA OFF", enum."ATTENDI FERMATA MOTORE", enum."ATTENDI FERMATA MOTORE", enum."ALIMENTATORE 1 DISABILITA", enum."SEGNALA FINE FERMATA", enum."FINE"] items=["FINE", "FRENO ABILITA", "FRENO DISABILITA", "FRENO MARCIA ON", "FRENO MARCIA OFF", "FRENO SET RIF PARTENZA", "FRENO FORZA RIF FERMATA", "FRENO SET RIF FERMATA", "FRENO SET RIF A 0", "FRENO FORZA RIF A 0", "FRENO SET CONTROLLO COPPIA", "FRENO SET CONTROLLO VELOCITA'", "FRENO SET SENSO ROTAZIONE", "FRENO SET SENS ROT SEGNO COPPIA", "FRENO CONFIG", "ALIMENTATORE 1 ABILITA", "ALIMENTATORE 1 DISABILITA", "ALIMENTATORE 1 MARCIA ON", "ALIMENTATORE 1 MARCIA OFF", "ALIMENTATORE 1 SET RIF", "ALIMENTATORE 1 SET RIF RIDOTTO", "ALIMENTATORE 1 SET RIF A 0", "ALIMENTATORE 1 RESET ALLARMI", "ALIMENTATORE 1 SCORTA 2", "ALIMENTATORE 1 SCORTA 3", "ALIMENTATORE 2 ABILITA", "ALIMENTATORE 2 DISABILITA", "ALIMENTATORE 2 MARCIA ON", "ALIMENTATORE 2 MARCIA OFF", "ALIMENTATORE 2 SET RIF", "ALIMENTATORE 2 SET RIF RIDOTTO", "ALIMENTATORE 2 SET RIF A 0", "ALIMENTATORE 2 SCORTA 1", "ALIMENTATORE 2 SCORTA 2", "ALIMENTATORE 2 SCORTA 3", "TELERUTTORI CHIUDI POTENZA", "TELERUTTORI APRI POTENZA", "TELERUTTORI ABILITA POTENZA", "TELERUTTORI DISABILITA POTENZA", "TELERUTTORI MISURA RESISTENZA RESISTOMAT", "TELERUTTORI MISURA RESISTENZA RES METER", "PROCEDURA ROTORE BLOCCATO 1", "ATTENDI FERMATA MOTORE", "SEGNALA INIZIO AVVIO", "SEGNALA FINE AVVIO", "SEGNALA INIZIO FERMATA", "SEGNALA FINE FERMATA", "START PROFILO", "ATTENDI FINE RAMPA"] ("appended array")
                # "solo alimentatore in marcia"
              }
              frame 3 {
                # "alimentatore e freno in marcia"
                n55 = disable-structure shown="Enabled" {
                  disable-tunnel: [w317 w319] -> w316
                  disable-tunnel: w315 -> [_ w318]
                  frame Disabled {
                    w317 = T5[] [enum."SEGNALA INIZIO FERMATA", enum."ALIMENTATORE 1 MARCIA OFF", enum."FRENO SET CONTROLLO COPPIA", enum."FRENO SET RIF FERMATA", enum."ATTENDI FERMATA MOTORE", enum."FRENO MARCIA OFF", enum."FRENO SET RIF A 0", enum."ATTENDI FERMATA MOTORE", enum."ALIMENTATORE 1 DISABILITA", enum."SEGNALA FINE FERMATA", enum."FINE"] items=["FINE", "FRENO ABILITA", "FRENO DISABILITA", "FRENO MARCIA ON", "FRENO MARCIA OFF", "FRENO SET RIF PARTENZA", "FRENO FORZA RIF FERMATA", "FRENO SET RIF FERMATA", "FRENO SET RIF A 0", "FRENO FORZA RIF A 0", "FRENO SET CONTROLLO COPPIA", "FRENO SET CONTROLLO VELOCITA'", "FRENO SET SENSO ROTAZIONE", "FRENO SET SENS ROT SEGNO COPPIA", "FRENO CONFIG", "ALIMENTATORE 1 ABILITA", "ALIMENTATORE 1 DISABILITA", "ALIMENTATORE 1 MARCIA ON", "ALIMENTATORE 1 MARCIA OFF", "ALIMENTATORE 1 SET RIF", "ALIMENTATORE 1 SET RIF RIDOTTO", "ALIMENTATORE 1 SET RIF A 0", "ALIMENTATORE 1 RESET ALLARMI", "ALIMENTATORE 1 SCORTA 2", "ALIMENTATORE 1 SCORTA 3", "ALIMENTATORE 2 ABILITA", "ALIMENTATORE 2 DISABILITA", "ALIMENTATORE 2 MARCIA ON", "ALIMENTATORE 2 MARCIA OFF", "ALIMENTATORE 2 SET RIF", "ALIMENTATORE 2 SET RIF RIDOTTO", "ALIMENTATORE 2 SET RIF A 0", "ALIMENTATORE 2 SCORTA 1", "ALIMENTATORE 2 SCORTA 2", "ALIMENTATORE 2 SCORTA 3", "TELERUTTORI CHIUDI POTENZA", "TELERUTTORI APRI POTENZA", "TELERUTTORI ABILITA POTENZA", "TELERUTTORI DISABILITA POTENZA", "TELERUTTORI MISURA RESISTENZA RESISTOMAT", "TELERUTTORI MISURA RESISTENZA RES METER", "PROCEDURA ROTORE BLOCCATO 1", "ATTENDI FERMATA MOTORE", "SEGNALA INIZIO AVVIO", "SEGNALA FINE AVVIO", "SEGNALA INIZIO FERMATA", "SEGNALA FINE FERMATA", "START PROFILO", "ATTENDI FINE RAMPA"] ("appended array")
                  }
                  frame Enabled {
                    n56 = case shown="\"Torque [Nm]\", \"Power [W]\", Default" w318 {
                      tunnel: [w320 w321] -> w319
                      frame "Torque [Nm]", "Power [W]", Default {
                        w320 = T5[] [enum."SEGNALA INIZIO FERMATA", enum."FRENO FORZA RIF A 0", enum."ALIMENTATORE 1 MARCIA OFF", enum."FRENO FORZA RIF FERMATA", enum."ATTENDI FERMATA MOTORE", enum."FRENO SET CONTROLLO COPPIA", enum."FRENO SET RIF A 0", enum."FRENO MARCIA OFF", enum."ALIMENTATORE 1 DISABILITA", enum."FRENO SET RIF A 0", enum."SEGNALA FINE FERMATA", enum."FINE"] items=["FINE", "FRENO ABILITA", "FRENO DISABILITA", "FRENO MARCIA ON", "FRENO MARCIA OFF", "FRENO SET RIF PARTENZA", "FRENO FORZA RIF FERMATA", "FRENO SET RIF FERMATA", "FRENO SET RIF A 0", "FRENO FORZA RIF A 0", "FRENO SET CONTROLLO COPPIA", "FRENO SET CONTROLLO VELOCITA'", "FRENO SET SENSO ROTAZIONE", "FRENO SET SENS ROT SEGNO COPPIA", "FRENO CONFIG", "ALIMENTATORE 1 ABILITA", "ALIMENTATORE 1 DISABILITA", "ALIMENTATORE 1 MARCIA ON", "ALIMENTATORE 1 MARCIA OFF", "ALIMENTATORE 1 SET RIF", "ALIMENTATORE 1 SET RIF RIDOTTO", "ALIMENTATORE 1 SET RIF A 0", "ALIMENTATORE 1 RESET ALLARMI", "ALIMENTATORE 1 SCORTA 2", "ALIMENTATORE 1 SCORTA 3", "ALIMENTATORE 2 ABILITA", "ALIMENTATORE 2 DISABILITA", "ALIMENTATORE 2 MARCIA ON", "ALIMENTATORE 2 MARCIA OFF", "ALIMENTATORE 2 SET RIF", "ALIMENTATORE 2 SET RIF RIDOTTO", "ALIMENTATORE 2 SET RIF A 0", "ALIMENTATORE 2 SCORTA 1", "ALIMENTATORE 2 SCORTA 2", "ALIMENTATORE 2 SCORTA 3", "TELERUTTORI CHIUDI POTENZA", "TELERUTTORI APRI POTENZA", "TELERUTTORI ABILITA POTENZA", "TELERUTTORI DISABILITA POTENZA", "TELERUTTORI MISURA RESISTENZA RESISTOMAT", "TELERUTTORI MISURA RESISTENZA RES METER", "PROCEDURA ROTORE BLOCCATO 1", "ATTENDI FERMATA MOTORE", "SEGNALA INIZIO AVVIO", "SEGNALA FINE AVVIO", "SEGNALA INIZIO FERMATA", "SEGNALA FINE FERMATA", "START PROFILO", "ATTENDI FINE RAMPA"] ("appended array")
                      }
                      frame "Speed [RPM]" {
                        w321 = T5[] [enum."SEGNALA INIZIO FERMATA", enum."ALIMENTATORE 1 MARCIA OFF", enum."FRENO FORZA RIF A 0", enum."FRENO FORZA RIF FERMATA", enum."ATTENDI FERMATA MOTORE", enum."FRENO SET CONTROLLO COPPIA", enum."FRENO SET RIF A 0", enum."FRENO MARCIA OFF", enum."ALIMENTATORE 1 DISABILITA", enum."FRENO SET RIF A 0", enum."SEGNALA FINE FERMATA", enum."FINE"] items=["FINE", "FRENO ABILITA", "FRENO DISABILITA", "FRENO MARCIA ON", "FRENO MARCIA OFF", "FRENO SET RIF PARTENZA", "FRENO FORZA RIF FERMATA", "FRENO SET RIF FERMATA", "FRENO SET RIF A 0", "FRENO FORZA RIF A 0", "FRENO SET CONTROLLO COPPIA", "FRENO SET CONTROLLO VELOCITA'", "FRENO SET SENSO ROTAZIONE", "FRENO SET SENS ROT SEGNO COPPIA", "FRENO CONFIG", "ALIMENTATORE 1 ABILITA", "ALIMENTATORE 1 DISABILITA", "ALIMENTATORE 1 MARCIA ON", "ALIMENTATORE 1 MARCIA OFF", "ALIMENTATORE 1 SET RIF", "ALIMENTATORE 1 SET RIF RIDOTTO", "ALIMENTATORE 1 SET RIF A 0", "ALIMENTATORE 1 RESET ALLARMI", "ALIMENTATORE 1 SCORTA 2", "ALIMENTATORE 1 SCORTA 3", "ALIMENTATORE 2 ABILITA", "ALIMENTATORE 2 DISABILITA", "ALIMENTATORE 2 MARCIA ON", "ALIMENTATORE 2 MARCIA OFF", "ALIMENTATORE 2 SET RIF", "ALIMENTATORE 2 SET RIF RIDOTTO", "ALIMENTATORE 2 SET RIF A 0", "ALIMENTATORE 2 SCORTA 1", "ALIMENTATORE 2 SCORTA 2", "ALIMENTATORE 2 SCORTA 3", "TELERUTTORI CHIUDI POTENZA", "TELERUTTORI APRI POTENZA", "TELERUTTORI ABILITA POTENZA", "TELERUTTORI DISABILITA POTENZA", "TELERUTTORI MISURA RESISTENZA RESISTOMAT", "TELERUTTORI MISURA RESISTENZA RES METER", "PROCEDURA ROTORE BLOCCATO 1", "ATTENDI FERMATA MOTORE", "SEGNALA INIZIO AVVIO", "SEGNALA FINE AVVIO", "SEGNALA INIZIO FERMATA", "SEGNALA FINE FERMATA", "START PROFILO", "ATTENDI FINE RAMPA"] ("appended array")
                      }
                    }
                  }
                }
              }
            }
            n57 = global write "Global FINE AVVIO.vi" "FINE AVVIO"(FALSE ("FINE AVVIO")) -> ()
            n58 = global write "Global prova in corso.vi" "prova in corso?"(FALSE ("prova in corso?")) -> ()
            n59 = case shown="True" w286 {
              tunnel: [w324 w326] -> w302
              tunnel: w301 -> [w323 _]
              tunnel: w292 -> [w322 w327]
              frame False {
                n60 = Build Array (concatenate)(w323, w322) -> (w324:T5[][])
              }
              frame True {
                w325 = T5[] [] items=["FINE", "FRENO ABILITA", "FRENO DISABILITA", "FRENO MARCIA ON", "FRENO MARCIA OFF", "FRENO SET RIF PARTENZA", "FRENO FORZA RIF FERMATA", "FRENO SET RIF FERMATA", "FRENO SET RIF A 0", "FRENO FORZA RIF A 0", "FRENO SET CONTROLLO COPPIA", "FRENO SET CONTROLLO VELOCITA'", "FRENO SET SENSO ROTAZIONE", "FRENO SET SENS ROT SEGNO COPPIA", "FRENO CONFIG", "ALIMENTATORE 1 ABILITA", "ALIMENTATORE 1 DISABILITA", "ALIMENTATORE 1 MARCIA ON", "ALIMENTATORE 1 MARCIA OFF", "ALIMENTATORE 1 SET RIF", "ALIMENTATORE 1 SET RIF RIDOTTO", "ALIMENTATORE 1 SET RIF A 0", "ALIMENTATORE 1 RESET ALLARMI", "ALIMENTATORE 1 SCORTA 2", "ALIMENTATORE 1 SCORTA 3", "ALIMENTATORE 2 ABILITA", "ALIMENTATORE 2 DISABILITA", "ALIMENTATORE 2 MARCIA ON", "ALIMENTATORE 2 MARCIA OFF", "ALIMENTATORE 2 SET RIF", "ALIMENTATORE 2 SET RIF RIDOTTO", "ALIMENTATORE 2 SET RIF A 0", "ALIMENTATORE 2 SCORTA 1", "ALIMENTATORE 2 SCORTA 2", "ALIMENTATORE 2 SCORTA 3", "TELERUTTORI CHIUDI POTENZA", "TELERUTTORI APRI POTENZA", "TELERUTTORI ABILITA POTENZA", "TELERUTTORI DISABILITA POTENZA", "TELERUTTORI MISURA RESISTENZA RESISTOMAT", "TELERUTTORI MISURA RESISTENZA RES METER", "PROCEDURA ROTORE BLOCCATO 1", "ATTENDI FERMATA MOTORE", "SEGNALA INIZIO AVVIO", "SEGNALA FINE AVVIO", "SEGNALA INIZIO FERMATA", "SEGNALA FINE FERMATA", "START PROFILO", "ATTENDI FINE RAMPA"] ("element")
                n61 = Build Array(w327, w325) -> (w326:T5[][])
              }
            }
          }
          frame "STOP FRENO" {
            w331 = T5[] [enum."FRENO SET CONTROLLO COPPIA", enum."FRENO SET RIF A 0", enum."FRENO MARCIA OFF", enum."FINE"] items=["FINE", "FRENO ABILITA", "FRENO DISABILITA", "FRENO MARCIA ON", "FRENO MARCIA OFF", "FRENO SET RIF PARTENZA", "FRENO FORZA RIF FERMATA", "FRENO SET RIF FERMATA", "FRENO SET RIF A 0", "FRENO FORZA RIF A 0", "FRENO SET CONTROLLO COPPIA", "FRENO SET CONTROLLO VELOCITA'", "FRENO SET SENSO ROTAZIONE", "FRENO SET SENS ROT SEGNO COPPIA", "FRENO CONFIG", "ALIMENTATORE 1 ABILITA", "ALIMENTATORE 1 DISABILITA", "ALIMENTATORE 1 MARCIA ON", "ALIMENTATORE 1 MARCIA OFF", "ALIMENTATORE 1 SET RIF", "ALIMENTATORE 1 SET RIF RIDOTTO", "ALIMENTATORE 1 SET RIF A 0", "ALIMENTATORE 1 RESET ALLARMI", "ALIMENTATORE 1 SCORTA 2", "ALIMENTATORE 1 SCORTA 3", "ALIMENTATORE 2 ABILITA", "ALIMENTATORE 2 DISABILITA", "ALIMENTATORE 2 MARCIA ON", "ALIMENTATORE 2 MARCIA OFF", "ALIMENTATORE 2 SET RIF", "ALIMENTATORE 2 SET RIF RIDOTTO", "ALIMENTATORE 2 SET RIF A 0", "ALIMENTATORE 2 SCORTA 1", "ALIMENTATORE 2 SCORTA 2", "ALIMENTATORE 2 SCORTA 3", "TELERUTTORI CHIUDI POTENZA", "TELERUTTORI APRI POTENZA", "TELERUTTORI ABILITA POTENZA", "TELERUTTORI DISABILITA POTENZA", "TELERUTTORI MISURA RESISTENZA RESISTOMAT", "TELERUTTORI MISURA RESISTENZA RES METER", "PROCEDURA ROTORE BLOCCATO 1", "ATTENDI FERMATA MOTORE", "SEGNALA INIZIO AVVIO", "SEGNALA FINE AVVIO", "SEGNALA INIZIO FERMATA", "SEGNALA FINE FERMATA", "START PROFILO", "ATTENDI FINE RAMPA"] ("appended array")
            # "STOP SOLO FRENO, SE L'ALIMENTATORE IN PROVA è ALIMENTATO"
            n62 = Build Array (concatenate)(w333, w331) -> (w332:T5[][])
          }
          frame "ABILITA POTENZA" {
            w339 = T5[] [enum."TELERUTTORI ABILITA POTENZA", enum."FINE"] items=["FINE", "FRENO ABILITA", "FRENO DISABILITA", "FRENO MARCIA ON", "FRENO MARCIA OFF", "FRENO SET RIF PARTENZA", "FRENO FORZA RIF FERMATA", "FRENO SET RIF FERMATA", "FRENO SET RIF A 0", "FRENO FORZA RIF A 0", "FRENO SET CONTROLLO COPPIA", "FRENO SET CONTROLLO VELOCITA'", "FRENO SET SENSO ROTAZIONE", "FRENO SET SENS ROT SEGNO COPPIA", "FRENO CONFIG", "ALIMENTATORE 1 ABILITA", "ALIMENTATORE 1 DISABILITA", "ALIMENTATORE 1 MARCIA ON", "ALIMENTATORE 1 MARCIA OFF", "ALIMENTATORE 1 SET RIF", "ALIMENTATORE 1 SET RIF RIDOTTO", "ALIMENTATORE 1 SET RIF A 0", "ALIMENTATORE 1 RESET ALLARMI", "ALIMENTATORE 1 SCORTA 2", "ALIMENTATORE 1 SCORTA 3", "ALIMENTATORE 2 ABILITA", "ALIMENTATORE 2 DISABILITA", "ALIMENTATORE 2 MARCIA ON", "ALIMENTATORE 2 MARCIA OFF", "ALIMENTATORE 2 SET RIF", "ALIMENTATORE 2 SET RIF RIDOTTO", "ALIMENTATORE 2 SET RIF A 0", "ALIMENTATORE 2 SCORTA 1", "ALIMENTATORE 2 SCORTA 2", "ALIMENTATORE 2 SCORTA 3", "TELERUTTORI CHIUDI POTENZA", "TELERUTTORI APRI POTENZA", "TELERUTTORI ABILITA POTENZA", "TELERUTTORI DISABILITA POTENZA", "TELERUTTORI MISURA RESISTENZA RESISTOMAT", "TELERUTTORI MISURA RESISTENZA RES METER", "PROCEDURA ROTORE BLOCCATO 1", "ATTENDI FERMATA MOTORE", "SEGNALA INIZIO AVVIO", "SEGNALA FINE AVVIO", "SEGNALA INIZIO FERMATA", "SEGNALA FINE FERMATA", "START PROFILO", "ATTENDI FINE RAMPA"] ("appended array")
            n63 = Variant To Data(type=T9 {"COLLEGAMENTO"=enum."AC TRIFASE", "LINEA ELETTRICA"=enum."LINEA 1"} ("Impostazioni elettriche 2"), Variant=w342) -> (data=w338:T9)  [unwired: 1 in, 1 out]
            n64 = Build Array (concatenate)(w341, w339) -> (w340:T5[][])
          }
          frame "DISABILITA POTENZA" {
            w348 = T5[] [enum."TELERUTTORI DISABILITA POTENZA", enum."FINE"] items=["FINE", "FRENO ABILITA", "FRENO DISABILITA", "FRENO MARCIA ON", "FRENO MARCIA OFF", "FRENO SET RIF PARTENZA", "FRENO FORZA RIF FERMATA", "FRENO SET RIF FERMATA", "FRENO SET RIF A 0", "FRENO FORZA RIF A 0", "FRENO SET CONTROLLO COPPIA", "FRENO SET CONTROLLO VELOCITA'", "FRENO SET SENSO ROTAZIONE", "FRENO SET SENS ROT SEGNO COPPIA", "FRENO CONFIG", "ALIMENTATORE 1 ABILITA", "ALIMENTATORE 1 DISABILITA", "ALIMENTATORE 1 MARCIA ON", "ALIMENTATORE 1 MARCIA OFF", "ALIMENTATORE 1 SET RIF", "ALIMENTATORE 1 SET RIF RIDOTTO", "ALIMENTATORE 1 SET RIF A 0", "ALIMENTATORE 1 RESET ALLARMI", "ALIMENTATORE 1 SCORTA 2", "ALIMENTATORE 1 SCORTA 3", "ALIMENTATORE 2 ABILITA", "ALIMENTATORE 2 DISABILITA", "ALIMENTATORE 2 MARCIA ON", "ALIMENTATORE 2 MARCIA OFF", "ALIMENTATORE 2 SET RIF", "ALIMENTATORE 2 SET RIF RIDOTTO", "ALIMENTATORE 2 SET RIF A 0", "ALIMENTATORE 2 SCORTA 1", "ALIMENTATORE 2 SCORTA 2", "ALIMENTATORE 2 SCORTA 3", "TELERUTTORI CHIUDI POTENZA", "TELERUTTORI APRI POTENZA", "TELERUTTORI ABILITA POTENZA", "TELERUTTORI DISABILITA POTENZA", "TELERUTTORI MISURA RESISTENZA RESISTOMAT", "TELERUTTORI MISURA RESISTENZA RES METER", "PROCEDURA ROTORE BLOCCATO 1", "ATTENDI FERMATA MOTORE", "SEGNALA INIZIO AVVIO", "SEGNALA FINE AVVIO", "SEGNALA INIZIO FERMATA", "SEGNALA FINE FERMATA", "START PROFILO", "ATTENDI FINE RAMPA"] ("appended array")
            n65 = Build Array (concatenate)(w347, w348) -> (w346:T5[][])
          }
          frame "MISURA RESISTENZA RESISTOMAT" {
            w359 = T5[] [enum."TELERUTTORI MISURA RESISTENZA RESISTOMAT", enum."FINE"] items=["FINE", "FRENO ABILITA", "FRENO DISABILITA", "FRENO MARCIA ON", "FRENO MARCIA OFF", "FRENO SET RIF PARTENZA", "FRENO FORZA RIF FERMATA", "FRENO SET RIF FERMATA", "FRENO SET RIF A 0", "FRENO FORZA RIF A 0", "FRENO SET CONTROLLO COPPIA", "FRENO SET CONTROLLO VELOCITA'", "FRENO SET SENSO ROTAZIONE", "FRENO SET SENS ROT SEGNO COPPIA", "FRENO CONFIG", "ALIMENTATORE 1 ABILITA", "ALIMENTATORE 1 DISABILITA", "ALIMENTATORE 1 MARCIA ON", "ALIMENTATORE 1 MARCIA OFF", "ALIMENTATORE 1 SET RIF", "ALIMENTATORE 1 SET RIF RIDOTTO", "ALIMENTATORE 1 SET RIF A 0", "ALIMENTATORE 1 RESET ALLARMI", "ALIMENTATORE 1 SCORTA 2", "ALIMENTATORE 1 SCORTA 3", "ALIMENTATORE 2 ABILITA", "ALIMENTATORE 2 DISABILITA", "ALIMENTATORE 2 MARCIA ON", "ALIMENTATORE 2 MARCIA OFF", "ALIMENTATORE 2 SET RIF", "ALIMENTATORE 2 SET RIF RIDOTTO", "ALIMENTATORE 2 SET RIF A 0", "ALIMENTATORE 2 SCORTA 1", "ALIMENTATORE 2 SCORTA 2", "ALIMENTATORE 2 SCORTA 3", "TELERUTTORI CHIUDI POTENZA", "TELERUTTORI APRI POTENZA", "TELERUTTORI ABILITA POTENZA", "TELERUTTORI DISABILITA POTENZA", "TELERUTTORI MISURA RESISTENZA RESISTOMAT", "TELERUTTORI MISURA RESISTENZA RES METER", "PROCEDURA ROTORE BLOCCATO 1", "ATTENDI FERMATA MOTORE", "SEGNALA INIZIO AVVIO", "SEGNALA FINE AVVIO", "SEGNALA INIZIO FERMATA", "SEGNALA FINE FERMATA", "START PROFILO", "ATTENDI FINE RAMPA"] ("appended array")
            n66 = Variant To Data(type=T3 {"#rami"=0, "Value"={"CH1 (ohm)"=0, "CH2 (ohm)"=0, "CH3 (ohm)"=0}} ("output cluster"), Variant=w355) -> (data=→"RESISTOMAT":T3)  [unwired: 1 in, 1 out]
            n67 = Build Array (concatenate)(w358, w359) -> (w357:T5[][])
          }
          frame "MISURA RESISTENZA RES METER" {
            w364 = T5[] [enum."TELERUTTORI MISURA RESISTENZA RES METER", enum."FINE"] items=["FINE", "FRENO ABILITA", "FRENO DISABILITA", "FRENO MARCIA ON", "FRENO MARCIA OFF", "FRENO SET RIF PARTENZA", "FRENO FORZA RIF FERMATA", "FRENO SET RIF FERMATA", "FRENO SET RIF A 0", "FRENO FORZA RIF A 0", "FRENO SET CONTROLLO COPPIA", "FRENO SET CONTROLLO VELOCITA'", "FRENO SET SENSO ROTAZIONE", "FRENO SET SENS ROT SEGNO COPPIA", "FRENO CONFIG", "ALIMENTATORE 1 ABILITA", "ALIMENTATORE 1 DISABILITA", "ALIMENTATORE 1 MARCIA ON", "ALIMENTATORE 1 MARCIA OFF", "ALIMENTATORE 1 SET RIF", "ALIMENTATORE 1 SET RIF RIDOTTO", "ALIMENTATORE 1 SET RIF A 0", "ALIMENTATORE 1 RESET ALLARMI", "ALIMENTATORE 1 SCORTA 2", "ALIMENTATORE 1 SCORTA 3", "ALIMENTATORE 2 ABILITA", "ALIMENTATORE 2 DISABILITA", "ALIMENTATORE 2 MARCIA ON", "ALIMENTATORE 2 MARCIA OFF", "ALIMENTATORE 2 SET RIF", "ALIMENTATORE 2 SET RIF RIDOTTO", "ALIMENTATORE 2 SET RIF A 0", "ALIMENTATORE 2 SCORTA 1", "ALIMENTATORE 2 SCORTA 2", "ALIMENTATORE 2 SCORTA 3", "TELERUTTORI CHIUDI POTENZA", "TELERUTTORI APRI POTENZA", "TELERUTTORI ABILITA POTENZA", "TELERUTTORI DISABILITA POTENZA", "TELERUTTORI MISURA RESISTENZA RESISTOMAT", "TELERUTTORI MISURA RESISTENZA RES METER", "PROCEDURA ROTORE BLOCCATO 1", "ATTENDI FERMATA MOTORE", "SEGNALA INIZIO AVVIO", "SEGNALA FINE AVVIO", "SEGNALA INIZIO FERMATA", "SEGNALA FINE FERMATA", "START PROFILO", "ATTENDI FINE RAMPA"] ("appended array")
            n68 = Variant To Data(type=0 ("#rami misura"), Variant=w367) -> (data=→"Rami misura":i32)  [unwired: 1 in, 1 out]
            n69 = Build Array (concatenate)(w363, w364) -> (w362:T5[][])
          }
          frame "PROVA ROTORE BLOCCATO" {
            n70 = Variant To Data(type=T11 {"TEMPO PROVA"=3.0} ("Rotore bloccato"), Variant=w376) -> (data=w374:T11)  [unwired: 1 in, 1 out]
            n71 = Unbundle By Name(w374) -> ("TEMPO PROVA"=→"TEMPO PROVA ROT BLOCC":dbl)
            n72 = global write "Global prova in corso.vi" "prova in corso?"(TRUE ("prova in corso?")) -> ()
            n73 = Build Array(Operazioni."ALIMENTATORE 1 MARCIA ON" ("OPERAZIONI"), Operazioni."PROCEDURA ROTORE BLOCCATO 1" ("OPERAZIONI"), Operazioni."ALIMENTATORE 1 MARCIA OFF" ("OPERAZIONI"), Operazioni."FINE" ("element")) -> (w379:T5[])
            n74 = Build Array (concatenate)(w381, w379) -> (w380:T5[][])
          }
          frame "CHIUDI POTENZA" {
            n75 = Build Array(Operazioni."TELERUTTORI CHIUDI POTENZA" ("OPERAZIONI"), Operazioni."FINE" ("OPERAZIONI")) -> (w388:T5[])
            n76 = Build Array (concatenate)(w390, w388) -> (w389:T5[][])
          }
          frame "APRI POTENZA" {
            n77 = Build Array(Operazioni."TELERUTTORI APRI POTENZA" ("OPERAZIONI"), Operazioni."FINE" ("OPERAZIONI")) -> (w399:T5[])
            n78 = Build Array (concatenate)(w398, w399) -> (w397:T5[][])
          }
          frame "ALLARME" {
            w411 = TRUE  # Priorità
            n79 = local read "Vi chiudi teler pot"() -> (w407:refnum<vi>)
            n80 = local read "Vi abilita pot"() -> (w406:refnum<vi>)
            n81 = Build Array(w406, w407) -> (w408:refnum<vi>[])
            n82 = for {
              tunnel: w408 -> [w418] mode=indexing
              n83 = invoke class="VI" method="FP.Close"(reference=w418) -> (error out=w417:errorcluster)  [unwired: 2 in, 2 out]
              n84 = call <vilib>:"Clear Errors.vi"("error in (no error)"=w417) -> ()  [unwired: 5 in, 2 out]
            }
            n85 = Build Array(Operazioni."ALIMENTATORE 1 MARCIA OFF" ("OPERAZIONI"), Operazioni."FRENO MARCIA OFF" ("OPERAZIONI"), Operazioni."FINE" ("element")) -> (w410:T5[])
            n86 = Build Array(w410) -> (w409:T5[][])
          }
          frame "START AFE ALTERNATORI" {
            n87 = global write "Global FINE AVVIO.vi" "START AFE ALTERNATORI"(TRUE ("AVVISO AVVIO IN CORSO")) -> ()
            n88 = Build Array(Operazioni."ALIMENTATORE 1 DISABILITA" ("OPERAZIONI"), Operazioni."ALIMENTATORE 1 SET RIF A 0" ("OPERAZIONI"), Operazioni."ALIMENTATORE 1 RESET ALLARMI" ("OPERAZIONI"), Operazioni."ALIMENTATORE 1 ABILITA" ("OPERAZIONI"), Operazioni."ALIMENTATORE 1 RESET ALLARMI" ("element"), Operazioni."ALIMENTATORE 1 MARCIA ON" ("element"), Operazioni."FINE" ("element")) -> (w429:T5[])
            n89 = Build Array (concatenate)(w420, w429) -> (w428:T5[][])
          }
          frame "STOP AFE ALTERNATORI" {
            n90 = Build Array(Operazioni."ALIMENTATORE 1 SET RIF A 0" ("OPERAZIONI"), Operazioni."ALIMENTATORE 1 MARCIA OFF" ("OPERAZIONI"), Operazioni."FINE" ("element")) -> (w440:T5[])
            n91 = global write "Global FINE AVVIO.vi" "STOP AFE ALTERNATORI"(TRUE ("AVVISO AVVIO IN CORSO")) -> ()
            n92 = Build Array (concatenate)(w434, w440) -> (w438:T5[][])
          }
          frame "STOP ALIMENTATORE" {
            n93 = Build Array(Operazioni."ALIMENTATORE 1 MARCIA OFF" ("OPERAZIONI"), Operazioni."FINE" ("element")) -> (w448:T5[])
            n94 = Build Array (concatenate)(w444, w448) -> (w445:T5[][])
          }
          frame "START PROFILO" {
            n95 = Build Array(Operazioni."START PROFILO" ("OPERAZIONI"), Operazioni."FINE" ("element")) -> (w457:T5[])
            n96 = Build Array (concatenate)(w452, w457) -> (w454:T5[][])
          }
          frame "CONFIG CONTROLLO FRENO" {
            n97 = Variant To Data(type=T2 {"Control Type"=enum."Torque [Nm]", "Set"=0.0, "Inverti senso di rotazione"=FALSE} ("Stato comandi freno.Control"), Variant=w464) -> (data=→"Data":T2)  [unwired: 1 in, 1 out]
            n98 = Build Array(Operazioni."FRENO CONFIG" ("OPERAZIONI"), Operazioni."FINE" ("element")) -> (w469:T5[])
            n99 = Build Array (concatenate)(w462, w469) -> (w466:T5[][])
          }
          frame "SVUOTA BUFFER PROCEDURE E OPERAZIONI" {
          }
        }
        "PROCEDURA" <- w55
        n100 = Or(x=w48, y=w68) -> (x .or. y?=w67:bool)
        n101 = case shown="True" w67 {
          tunnel: w49 -> [_ w78]
          frame False {
          }
          frame True {
            n102 = Enqueue Element(queue=w78, element=cluster{"Status":string, "variant":variant} {"Status"="ESTRAI PROCEDURA", "variant"=variant}) -> ()  [unwired: 2 in, 3 out]
          }
        }
        n103 = local write "Stato"("Default" ("Stato")) -> ()
        n104 = case shown="False" w48 {
          tunnel: w61 -> [w74 w77]
          tunnel: [w73 w75] -> w60
          tunnel: w51 -> [w72 w76]
          frame False {
            n105 = Build Array (concatenate)(w72, w74) -> (w73:T4[])
          }
          frame True {
            n106 = Build Array (concatenate)(w77, w76) -> (w75:T4[])
          }
        }
      }
      frame "AGGIORNA CONDIZIONI DI AVVIO" {
      }
      frame "EXIT" {
        w481 = TRUE
        n107 = property on="EXIT" class="Bool (strict)"("Val(Sgnl)"=w481) -> ()  [unwired: 2 in, 2 out]
      }
      frame "ESTRAI PROCEDURA" {
        n108 = Empty Array?(array=w501) -> (empty?=w488:bool)
        n109 = Select(t=T8 {"Message"="IDLE", "Message Data"=variant} ("element"), s=w488, f=T8 {"Message"="ESEGUI", "Message Data"=variant} ("element")) -> (s? t:f=w497:T8)
        n110 = case shown="True" w488 {
          frame False {
          }
          frame True {
            n111 = flat-sequence {
              frame #0 {
                n112 = global write "Global Fine procedure.vi" "Fine procedure?"(TRUE ("Fine procedure?")) -> ()
              }
              frame #1 {
                n113 = Wait (ms)(milliseconds to wait=u32 1000) -> ()  [unwired: 1 out]
              }
            }
          }
        }
        n114 = Enqueue Element(queue=w500, element=w497) -> ()  [unwired: 2 in, 3 out]
        n115 = Delete From Array(array=w501, index (row)=0) -> (deleted portion=w502:T5[], array with subset deleted=w504:T5[][])  [unwired: 2 in]
        n116 = Delete From Array(array=w495, length=1, index=0) -> (deleted portion=w491:T4[], array with subset deleted=w494:T4[])
        n117 = Index Array(array=w491) -> (element=→"Element":T4)  [unwired: 1 in]
      }
      frame "ESEGUI" {
        n118 = global read "Global_All_Data.vi" "All Data"() -> (w522:T34)
        n119 = Index Array(array=w533, index=0) -> (element=w534:T5)
        "OPERAZIONE IN CORSO" <- w534
        n120 = case shown="\"ATTENDI FINE RAMPA\"" w534 {
          tunnel: [w565 w616 w621 w652 w684 w717 w771 w814 w867 w899 w933 w964 w1013 w1085 w1116 w1146 w1177 TRUE w1216 w1245 w1278 w1307 _ _ w1328 w1334 w1455 w1473 w1526 _ _ _ _ _ _ _ _ _ w1546 _ _ TRUE TRUE TRUE TRUE w1571 w1609 TRUE ("Time has Elapsed") TRUE] -> w526
          tunnel: w533 -> [w568 w620 w624 w655 w687 w721 w774 w817 w869 w902 w936 w965 w1017 w1087 w1118 w1148 w1179 w1210 w1221 w1254 w1280 w1310 w1322 w1323 w1330 w1340 w1458 w1475 w1530 _ w1535 w1536 w1537 w1538 w1539 w1540 w1541 w1542 w1549 w1550 w1551 w1556 w1561 w1566 w1570 w1572 w1615 w1622 w1624]
          tunnel: [w568 w620 w624 w655 w687 w721 w774 w817 w869 w902 w936 w965 w1017 w1087 w1118 w1148 w1179 w1210 w1221 w1254 w1280 w1310 w1322 w1323 w1330 w1340 w1458 w1475 w1530 w1534 w1535 w1536 w1537 w1538 w1539 w1540 w1541 w1542 w1549 w1550 w1551 w1556 w1561 w1566 w1570 w1572 w1615 w1622 w1624] -> w521
          tunnel: w528 -> [_ _ _ _ _ w718 _ _ _ _ w932 _ _ _ _ _ _ _ w1220 w1253 _ _ _ _ _ _ _ _ _ _ _ _ _ _ _ _ _ _ _ _ _ _ _ _ _ _ _ _ _]
          tunnel: w527 -> [w567 _ w623 w654 w686 w720 w773 w816 w866 w901 w935 _ w1016 _ _ _ _ _ _ _ _ _ _ _ _ w1332 _ _ w1528 _ _ _ _ _ _ _ _ _ w1547 _ _ _ _ _ _ _ _ _ _]
          tunnel: w525 -> [w566 _ w622 w653 w685 w719 w772 w815 w868 w900 w934 _ w1015 _ _ _ _ _ _ _ _ _ _ _ _ _ _ _ _ _ _ _ _ _ _ _ _ _ _ _ _ _ _ _ _ _ _ _ _]
          tunnel: w524 -> [_ w614 _ _ _ _ _ _ _ _ _ _ _ w1086 w1117 w1147 w1178 _ w1219 w1248 w1279 _ _ _ _ w1331 _ _ w1527 _ _ _ _ _ _ _ _ _ w1548 _ _ _ _ _ _ _ _ _ _]
          tunnel: w520 -> [_ _ _ _ _ _ _ _ _ _ _ _ _ _ _ _ _ _ _ _ _ _ _ _ w1329 w1336 w1457 _ _ _ _ _ _ _ _ _ _ _ _ _ _ _ _ _ _ _ _ _ _]
          tunnel: w522 -> [_ w615 _ _ _ _ _ _ _ _ _ _ _ _ _ _ _ _ _ _ _ _ _ _ w1327 w1335 w1456 w1474 w1529 _ _ _ _ _ _ _ _ _ _ _ _ _ _ _ _ _ w1614 _ _]
          tunnel: w510 -> [_ _ _ _ _ _ _ _ _ _ _ _ _ _ _ _ _ _ _ _ _ _ _ _ _ _ w1453 w1472 _ _ _ _ _ _ _ _ _ _ _ _ _ _ _ _ _ _ w1603 _ _]
          tunnel: [_ _ _ _ _ _ _ _ _ _ _ _ _ _ _ _ _ _ _ _ _ _ _ _ _ _ _ _ w1522 _ _ _ _ _ _ _ _ _ _ _ _ _ _ _ _ _ _ _ _] -> w507
          frame "FRENO MARCIA ON", Default {
            n121 = while {
              tunnel: [w575] -> w565
              tunnel: w566 -> [w574]
              shift-right: [w571] -> _
              shift-left: _ -> [w570]
              tunnel: w567 -> [w569]
              stop <- TRUE stop-if-true
              n122 = local read "Stato"() -> (w573:string)
              n123 = case shown="\"Marcia\"" w573 {
                selector: w573 -> [w580 _ _ _]
                tunnel: [w579 "Reset OFF" ("t") "Marcia" ("t") "wait"] -> w572
                tunnel: [w577 _ _ _] -> w575
                tunnel: w574 -> [w585 _ _ _]
                tunnel: [_ _ _ TRUE] -> w571
                tunnel: w570 -> [w584 _ _ _]
                tunnel: w569 -> [_ _ _ w592]
                frame "wait" {
                  n124 = Unbundle By Name(w585) -> ("Start"=w577:bool)
                  n125 = call "Elapsed Time2"("Time Target (s)"=5.0, "Reset"=w584, "Auto Reset"=FALSE) -> ("Time has Elapsed"=w581:bool)  [unwired: 9 in, 7 out]
                  n126 = Select(t="Default", s=w581, f=w580) -> (s? t:f=w579:string)
                }
                frame "Reset ON", Default {
                  n127 = disable-structure shown="Disabled" {
                    frame Disabled {
                      n128 = call "Set DO.vi"("Cluster SET DO"=T13 [{"DO"=enum."Comando azionam in blocco", "Value"=FALSE}, {"DO"=enum."Comando azionam reset", "Value"=TRUE}]) -> ()  [unwired: 10 in, 1 out]
                    }
                    frame Enabled {
                    }
                  }
                }
                frame "Reset OFF" {
                  n129 = disable-structure shown="Disabled" {
                    frame Disabled {
                      n130 = call "Set DO.vi"("Cluster SET DO"=T13 [{"DO"=enum."Comando azionam in blocco", "Value"=FALSE}, {"DO"=enum."Comando azionam reset", "Value"=FALSE}]) -> ()  [unwired: 10 in, 1 out]
                    }
                    frame Enabled {
                    }
                  }
                }
                frame "Marcia" {
                  n131 = Bundle By Name(cluster=w592, "Start\\stop.Start"=TRUE ("Command.Start"), "Start\\stop.STOP"=FALSE ("Start\\stop.Stop")) -> (w595:T26)
                  n132 = Obtain Queue(name (unnamed)="FRENI", element data type=T8 {"Message"="", "Message Data"=variant} ("Message Cluster")) -> (queue out=w599:refnum<queue>)  [unwired: 3 in, 2 out]
                  n133 = Bundle By Name(cluster=cluster{"Status":string, "variant":variant} {"Status"="AGGIORNA COMANDI FRENO", "variant"=variant}, "variant"=w595) -> (w596:cluster{"Status":string, "variant":variant})
                  n134 = Enqueue Element(queue=w599, element=w596) -> ()  [unwired: 2 in, 3 out]
                }
              }
              n135 = local write "Stato"(w572) -> ()
            }
          }
          frame "ATTENDI FINE RAMPA" {
            n136 = Unbundle By Name(w614) -> ("RIF 2"=w605:dbl)
            n137 = Unbundle By Name(w615) -> ("MISURE NM.f [Hz]"=w613:string)
            n138 = Divide(x=w605, y=100.0) -> (x/y=w610:dbl)
            n139 = Multiply(x=w610, y=5.0) -> (x*y=w608:dbl)
            n140 = Equal To 0?(x=w605) -> (x = 0?=w604:bool)
            n141 = Fract/Exp String To Number(string=w613) -> (number=w612:dbl)  [unwired: 3 in, 1 out]
            n142 = Add(x=w605, y=w608) -> (x+y=w607:dbl)
            n143 = Subtract(x=w605, y=w608) -> (x-y=w606:dbl)
            n144 = In Range and Coerce(upper limit=w607, x=w612, lower limit=w606) -> (In Range?=w602:bool)  [unwired: 1 out]
            n145 = Select(t=TRUE ("Auto Reset"), s=w604, f=w602) -> (s? t:f=w601:bool)
            n146 = Not(x=w601) -> (.not. x?=w619:bool)
            n147 = call "Elapsed Time27"("Time Target (s)"=2.0, "Reset"=w619, "Auto Reset"=FALSE) -> ("Time has Elapsed"=w616:bool)  [unwired: 9 in, 7 out]
          }
          frame "FRENO ABILITA" {
            n148 = while {
              tunnel: [w631] -> w621
              tunnel: w622 -> [w630]
              shift-right: [w627] -> _
              shift-left: _ -> [w626]
              tunnel: w623 -> [w625]
              stop <- TRUE stop-if-true
              n149 = local read "Stato"() -> (w629:string)
              n150 = case shown="\"True\", Default" w629 {
                selector: w629 -> [w637 _]
                tunnel: [w636 "wait"] -> w628
                tunnel: [w634 _] -> w631
                tunnel: w630 -> [_ _]
                tunnel: [_ TRUE] -> w627
                tunnel: w626 -> [w641 _]
                tunnel: w625 -> [w633 w643]
                frame "wait" {
                  n151 = Unbundle By Name(w633) -> ("Status.Ready"=w634:bool)
                  n152 = call "Elapsed Time14"("Time Target (s)"=5.0, "Reset"=w641, "Auto Reset"=FALSE) -> ("Time has Elapsed"=w638:bool)  [unwired: 9 in, 7 out]
                  n153 = Select(t="Default", s=w638, f=w637) -> (s? t:f=w636:string)
                }
                frame "True", Default {
                  n154 = Bundle By Name(cluster=w643, "Abilita.Abilita"=TRUE ("Command.Start")) -> (w646:T26)
                  n155 = Obtain Queue(name (unnamed)="FRENI", element data type=T8 {"Message"="", "Message Data"=variant} ("Message Cluster")) -> (queue out=w650:refnum<queue>)  [unwired: 3 in, 2 out]
                  n156 = Bundle By Name(cluster=cluster{"Status":string, "variant":variant} {"Status"="AGGIORNA COMANDI FRENO", "variant"=variant}, "variant"=w646) -> (w647:cluster{"Status":string, "variant":variant})
                  n157 = Enqueue Element(queue=w650, element=w647) -> ()  [unwired: 2 in, 3 out]
                }
              }
              n158 = local write "Stato"(w628) -> ()
            }
          }
          frame "FRENO DISABILITA" {
            n159 = while {
              tunnel: [w662] -> w652
              tunnel: w653 -> [w661]
              shift-right: [w658] -> _
              shift-left: _ -> [w657]
              tunnel: w654 -> [w656]
              stop <- TRUE stop-if-true
              n160 = local read "Stato"() -> (w660:string)
              n161 = case shown="\"True\", Default" w660 {
                selector: w660 -> [w669 _]
                tunnel: [w668 "wait"] -> w659
                tunnel: [w664 _] -> w662
                tunnel: w661 -> [_ _]
                tunnel: [_ TRUE] -> w658
                tunnel: w657 -> [w673 _]
                tunnel: w656 -> [w665 w675]
                frame "wait" {
                  n162 = Unbundle By Name(w665) -> ("Status.Ready"=w666:bool)
                  n163 = call "Elapsed Time15"("Time Target (s)"=5.0, "Reset"=w673, "Auto Reset"=FALSE) -> ("Time has Elapsed"=w670:bool)  [unwired: 9 in, 7 out]
                  n164 = Not(x=w666) -> (.not. x?=w664:bool)
                  n165 = Select(t="Default", s=w670, f=w669) -> (s? t:f=w668:string)
                }
                frame "True", Default {
                  n166 = Bundle By Name(cluster=w675, "Abilita.Abilita"=FALSE ("Command.Start")) -> (w678:T26)
                  n167 = Obtain Queue(name (unnamed)="FRENI", element data type=T8 {"Message"="", "Message Data"=variant} ("Message Cluster")) -> (queue out=w682:refnum<queue>)  [unwired: 3 in, 2 out]
                  n168 = Bundle By Name(cluster=cluster{"Status":string, "variant":variant} {"Status"="AGGIORNA COMANDI FRENO", "variant"=variant}, "variant"=w678) -> (w679:cluster{"Status":string, "variant":variant})
                  n169 = Enqueue Element(queue=w682, element=w679) -> ()  [unwired: 2 in, 3 out]
                }
              }
              n170 = local write "Stato"(w659) -> ()
            }
          }
          frame "FRENO MARCIA OFF" {
            n171 = while {
              tunnel: [w694] -> w684
              tunnel: w685 -> [w693]
              shift-right: [w690] -> _
              shift-left: _ -> [w689]
              tunnel: w686 -> [w688]
              stop <- TRUE stop-if-true
              n172 = local read "Stato"() -> (w692:string)
              n173 = case shown="\"True\", Default" w692 {
                selector: w692 -> [w700 _]
                tunnel: [w699 "wait"] -> w691
                tunnel: [w696 _] -> w694
                tunnel: w693 -> [w705 _]
                tunnel: [_ TRUE] -> w690
                tunnel: w689 -> [w704 _]
                tunnel: w688 -> [_ w708]
                frame "wait" {
                  n174 = Unbundle By Name(w705) -> ("Start"=w697:bool)
                  n175 = call "Elapsed Time3"("Time Target (s)"=5.0, "Reset"=w704, "Auto Reset"=FALSE) -> ("Time has Elapsed"=w701:bool)  [unwired: 9 in, 7 out]
                  n176 = Not(x=w697) -> (.not. x?=w696:bool)
                  n177 = Select(t="Default", s=w701, f=w700) -> (s? t:f=w699:string)
                }
                frame "True", Default {
                  n178 = Bundle By Name(cluster=w708, "Start\\stop.Start"=FALSE ("Command.Start"), "Start\\stop.STOP"=TRUE ("Start\\stop.Stop")) -> (w711:T26)
                  n179 = Obtain Queue(name (unnamed)="FRENI", element data type=T8 {"Message"="", "Message Data"=variant} ("Message Cluster")) -> (queue out=w715:refnum<queue>)  [unwired: 3 in, 2 out]
                  n180 = Bundle By Name(cluster=cluster{"Status":string, "variant":variant} {"Status"="AGGIORNA COMANDI FRENO", "variant"=variant}, "variant"=w711) -> (w712:cluster{"Status":string, "variant":variant})
                  n181 = Enqueue Element(queue=w715, element=w712) -> ()  [unwired: 2 in, 3 out]
                }
              }
              n182 = local write "Stato"(w691) -> ()
            }
          }
          frame "FRENO SET RIF PARTENZA" {
            n183 = while {
              tunnel: [w729] -> w717
              tunnel: w719 -> [w728]
              shift-right: [w725] -> _
              shift-left: _ -> [w724]
              tunnel: w720 -> [w723]
              tunnel: w718 -> [w722]
              stop <- TRUE stop-if-true
              n184 = local read "Stato"() -> (w727:string)
              n185 = case shown="\"True\", Default" w727 {
                selector: w727 -> [w736 _]
                tunnel: [w735 "wait"] -> w726
                tunnel: [w731 _] -> w729
                tunnel: w728 -> [w741 _]
                tunnel: [_ TRUE] -> w725
                tunnel: w724 -> [w740 _]
                tunnel: w723 -> [w733 w749]
                tunnel: w722 -> [_ w748]
                frame "wait" {
                  n186 = Unbundle By Name(w733) -> ("Control.Control Type"=w732:T61)
                  n187 = case shown="\"Torque [Nm]\", Default" w732 {
                    tunnel: w741 -> [w743 w745 w747]
                    tunnel: [w742 w744 w746] -> w731
                    frame "Torque [Nm]", Default {
                      n188 = Unbundle By Name(w743) -> ("Fine rampa C"=w742:bool)
                    }
                    frame "Power [W]" {
                      n189 = Unbundle By Name(w745) -> ("Fine rampa C"=w744:bool)
                    }
                    frame "Speed [RPM]" {
                      n190 = Unbundle By Name(w747) -> ("Fine rampa RPM"=w746:bool)
                    }
                  }
                  n191 = call "Elapsed Time4"("Time Target (s)"=5.0, "Reset"=w740, "Auto Reset"=FALSE) -> ("Time has Elapsed"=w737:bool)  [unwired: 9 in, 7 out]
                  n192 = Select(t="Default", s=w737, f=w736) -> (s? t:f=w735:string)
                }
                frame "True", Default {
                  n193 = Unbundle By Name(w749) -> ("Control.Control Type"=w750:T61)
                  n194 = Unbundle By Name(w748) -> ("C avvio [Nm]"=w751:dbl, "RPM avvio"=w752:dbl)
                  n195 = case shown="\"Torque [Nm]\", Default" w750 {
                    tunnel: w751 -> [w755 _ _]
                    tunnel: w752 -> [_ w763 _]
                    tunnel: w749 -> [w757 w765 _]
                    frame "Torque [Nm]", Default {
                      n196 = Bundle By Name(cluster=w757, "Control.Set"=w755) -> (w756:T26)
                      n197 = Obtain Queue(name (unnamed)="FRENI", element data type=T8 {"Message"="", "Message Data"=variant} ("Message Cluster")) -> (queue out=w761:refnum<queue>)  [unwired: 3 in, 2 out]
                      n198 = Bundle By Name(cluster=cluster{"Status":string, "variant":variant} {"Status"="AGGIORNA COMANDI FRENO", "variant"=variant}, "variant"=w756) -> (w758:cluster{"Status":string, "variant":variant})
                      n199 = Enqueue Element(queue=w761, element=w758) -> ()  [unwired: 2 in, 3 out]
                    }
                    frame "Speed [RPM]" {
                      n200 = Bundle By Name(cluster=w765, "Control.Set"=w763) -> (w764:T26)
                      n201 = Obtain Queue(name (unnamed)="FRENI", element data type=T8 {"Message"="", "Message Data"=variant} ("Message Cluster")) -> (queue out=w769:refnum<queue>)  [unwired: 3 in, 2 out]
                      n202 = Bundle By Name(cluster=cluster{"Status":string, "variant":variant} {"Status"="AGGIORNA COMANDI FRENO", "variant"=variant}, "variant"=w764) -> (w766:cluster{"Status":string, "variant":variant})
                      n203 = Enqueue Element(queue=w769, element=w766) -> ()  [unwired: 2 in, 3 out]
                    }
                    frame "Power [W]" {
                    }
                  }
                }
              }
              n204 = local write "Stato"(w726) -> ()
            }
          }
          frame "FRENO SET RIF FERMATA" {
            # "QUI IL FRENO è GIà IN CONTROL TYPE \"COPPIA\" (PROCEDURA \"STOP AUTOMATICO\"). in caso contrario esci"
            n205 = while {
              tunnel: [w781] -> w771
              tunnel: w772 -> [w780]
              shift-right: [w777] -> _
              shift-left: _ -> [w776]
              tunnel: w773 -> [w775]
              stop <- TRUE stop-if-true
              n206 = local read "Stato"() -> (w779:string)
              n207 = case shown="\"True\", Default" w779 {
                selector: w779 -> [w788 _]
                tunnel: [w787 "wait"] -> w778
                tunnel: [w783 _] -> w781
                tunnel: w780 -> [w793 _]
                tunnel: [_ TRUE] -> w777
                tunnel: w776 -> [w792 _]
                tunnel: w775 -> [w785 w799]
                frame "wait" {
                  n208 = Unbundle By Name(w785) -> ("Control.Control Type"=w784:T61)
                  n209 = case shown="\"Power [W]\"" w784 {
                    tunnel: w793 -> [w795 _ _]
                    tunnel: [w794 TRUE TRUE ("Fine rampa C")] -> w783
                    frame "Torque [Nm]", Default {
                      n210 = Unbundle By Name(w795) -> ("Fine rampa C"=w794:bool)
                    }
                    frame "Power [W]" {
                    }
                    frame "Speed [RPM]" {
                    }
                  }
                  n211 = call "Elapsed Time10"("Time Target (s)"=5.0, "Reset"=w792, "Auto Reset"=FALSE) -> ("Time has Elapsed"=w789:bool)  [unwired: 9 in, 7 out]
                  n212 = Select(t="Default", s=w789, f=w788) -> (s? t:f=w787:string)
                }
                frame "True", Default {
                  w798 = 10.0  # C FERMATA [Nm]
                  n213 = Unbundle By Name(w799) -> ("Control.Control Type"=w800:T61)
                  n214 = case shown="\"Torque [Nm]\", Default" w800 {
                    tunnel: w798 -> [w803 _ _]
                    tunnel: w799 -> [w804 _ _]
                    frame "Torque [Nm]", Default {
                      n215 = stacked-sequence {
                        tunnel: w804 -> [w807 _]
                        tunnel: w803 -> [w805 _]
                        frame #0 {
                          n216 = Bundle By Name(cluster=w807, "Control.Set"=w805) -> (w806:T26)
                          n217 = Obtain Queue(name (unnamed)="FRENI", element data type=T8 {"Message"="", "Message Data"=variant} ("Message Cluster")) -> (queue out=w811:refnum<queue>)  [unwired: 3 in, 2 out]
                          n218 = Bundle By Name(cluster=cluster{"Status":string, "variant":variant} {"Status"="AGGIORNA COMANDI FRENO", "variant"=variant}, "variant"=w806) -> (w808:cluster{"Status":string, "variant":variant})
                          n219 = Enqueue Element(queue=w811, element=w808) -> ()  [unwired: 2 in, 3 out]
                        }
                        frame #1 {
                          n220 = Wait (ms)(milliseconds to wait=u32 3000) -> ()  [unwired: 1 out]
                        }
                      }
                    }
                    frame "Speed [RPM]" {
                    }
                    frame "Power [W]" {
                    }
                  }
                }
              }
              n221 = local write "Stato"(w778) -> ()
            }
          }
          frame "FRENO SET RIF A 0" {
            n222 = while {
              tunnel: [w824] -> w814
              tunnel: w815 -> [w823]
              shift-right: [w820] -> _
              shift-left: _ -> [w819]
              tunnel: w816 -> [w818]
              stop <- TRUE stop-if-true
              n223 = local read "Stato"() -> (w822:string)
              n224 = case shown="\"True\", Default" w822 {
                selector: w822 -> [w831 _]
                tunnel: [w830 "wait"] -> w821
                tunnel: [w826 _] -> w824
                tunnel: w823 -> [w836 _]
                tunnel: [_ TRUE] -> w820
                tunnel: w819 -> [w835 _]
                tunnel: w818 -> [w828 w843]
                frame "wait" {
                  n225 = Unbundle By Name(w828) -> ("Control.Control Type"=w827:T61)
                  n226 = case shown="\"Torque [Nm]\", Default" w827 {
                    tunnel: w836 -> [w838 w840 w842]
                    tunnel: [TRUE w839 w841] -> w826
                    frame "Torque [Nm]", Default {
                      (unwired) FALSE ("Fine rampa RPM")
                      n227 = Unbundle By Name(w838) -> ()  [unwired: 1 out]
                    }
                    frame "Power [W]" {
                      n228 = Unbundle By Name(w840) -> ("Fine rampa C"=w839:bool)
                    }
                    frame "Speed [RPM]" {
                      n229 = Unbundle By Name(w842) -> ("Fine rampa RPM"=w841:bool)
                    }
                  }
                  n230 = call "Elapsed Time5"("Time Target (s)"=5.0, "Reset"=w835, "Auto Reset"=FALSE) -> ("Time has Elapsed"=w832:bool)  [unwired: 9 in, 7 out]
                  n231 = Select(t="Default", s=w832, f=w831) -> (s? t:f=w830:string)
                }
                frame "True", Default {
                  n232 = flat-sequence {
                    tunnel: w843 -> [w847]
                    frame #0 {
                      n233 = Unbundle By Name(w847) -> ("Control.Control Type"=w848:T61)
                      n234 = case shown="\"Torque [Nm]\", Default" w848 {
                        tunnel: w847 -> [w851 w859 _]
                        tunnel: 0.0 -> [w849 w857 _]
                        frame "Torque [Nm]", Default {
                          n235 = Bundle By Name(cluster=w851, "Control.Set"=w849) -> (w850:T26)
                          n236 = Obtain Queue(name (unnamed)="FRENI", element data type=T8 {"Message"="", "Message Data"=variant} ("Message Cluster")) -> (queue out=w855:refnum<queue>)  [unwired: 3 in, 2 out]
                          n237 = Bundle By Name(cluster=cluster{"Status":string, "variant":variant} {"Status"="AGGIORNA COMANDI FRENO", "variant"=variant}, "variant"=w850) -> (w852:cluster{"Status":string, "variant":variant})
                          n238 = Enqueue Element(queue=w855, element=w852) -> ()  [unwired: 2 in, 3 out]
                        }
                        frame "Speed [RPM]" {
                          n239 = Bundle By Name(cluster=w859, "Control.Set"=w857) -> (w858:T26)
                          n240 = Obtain Queue(name (unnamed)="FRENI", element data type=T8 {"Message"="", "Message Data"=variant} ("Message Cluster")) -> (queue out=w863:refnum<queue>)  [unwired: 3 in, 2 out]
                          n241 = Bundle By Name(cluster=cluster{"Status":string, "variant":variant} {"Status"="AGGIORNA COMANDI FRENO", "variant"=variant}, "variant"=w858) -> (w860:cluster{"Status":string, "variant":variant})
                          n242 = Enqueue Element(queue=w863, element=w860) -> ()  [unwired: 2 in, 3 out]
                        }
                        frame "Power [W]" {
                        }
                      }
                    }
                    frame #1 {
                      n243 = Wait (ms)(milliseconds to wait=u32 500) -> ()  [unwired: 1 out]
                    }
                  }
                }
              }
              n244 = local write "Stato"(w821) -> ()
            }
          }
          frame "FRENO SET CONTROLLO COPPIA" {
            n245 = while {
              tunnel: [w876] -> w867
              tunnel: w868 -> [w875]
              shift-right: [w872] -> _
              shift-left: _ -> [w871]
              tunnel: w866 -> [w870]
              stop <- TRUE stop-if-true
              n246 = local read "Stato"() -> (w874:string)
              n247 = case shown="\"True\", Default" w874 {
                selector: w874 -> [w880 _]
                tunnel: [w879 "wait"] -> w873
                tunnel: [w886 _] -> w876
                tunnel: w875 -> [w885 _]
                tunnel: [_ TRUE] -> w872
                tunnel: w871 -> [w884 _]
                tunnel: w870 -> [_ w889]
                frame "wait" {
                  n248 = Unbundle By Name(w885) -> ("Controllo effettivo"=w887:T16)
                  n249 = call "Elapsed Time"("Time Target (s)"=5.0, "Reset"=w884, "Auto Reset"=FALSE) -> ("Time has Elapsed"=w881:bool)  [unwired: 9 in, 7 out]
                  n250 = Equal?(x=w887, y=T16."Torque [Nm]") -> (x = y?=w886:bool)
                  n251 = Select(t="Default", s=w881, f=w880) -> (s? t:f=w879:string)
                }
                frame "True", Default {
                  n252 = Bundle By Name(cluster=w889, "Control.Control Type"=T16."Torque [Nm]") -> (w892:T26)
                  n253 = Obtain Queue(name (unnamed)="FRENI", element data type=T8 {"Message"="", "Message Data"=variant} ("Message Cluster")) -> (queue out=w896:refnum<queue>)  [unwired: 3 in, 2 out]
                  n254 = Bundle By Name(cluster=cluster{"Status":string, "variant":variant} {"Status"="AGGIORNA COMANDI FRENO", "variant"=variant}, "variant"=w892) -> (w893:cluster{"Status":string, "variant":variant})
                  n255 = Enqueue Element(queue=w896, element=w893) -> ()  [unwired: 2 in, 3 out]
                }
              }
              n256 = local write "Stato"(w873) -> ()
            }
          }
          frame "FRENO SET CONTROLLO VELOCITA'" {
            n257 = while {
              tunnel: [w909] -> w899
              tunnel: w900 -> [w908]
              shift-right: [w905] -> _
              shift-left: _ -> [w904]
              tunnel: w901 -> [w903]
              stop <- TRUE stop-if-true
              n258 = local read "Stato"() -> (w907:string)
              n259 = case shown="\"wait\"" w907 {
                selector: w907 -> [w913 _]
                tunnel: [w912 "wait"] -> w906
                tunnel: [w919 _] -> w909
                tunnel: w908 -> [w918 _]
                tunnel: [_ TRUE] -> w905
                tunnel: w904 -> [w917 _]
                tunnel: w903 -> [_ w922]
                frame "wait" {
                  n260 = Unbundle By Name(w918) -> ("Controllo effettivo"=w920:T16)
                  n261 = call "Elapsed Time6"("Time Target (s)"=5.0, "Reset"=w917, "Auto Reset"=FALSE) -> ("Time has Elapsed"=w914:bool)  [unwired: 9 in, 7 out]
                  n262 = Equal?(x=w920, y=T16."Speed [RPM]") -> (x = y?=w919:bool)
                  n263 = Select(t="Default", s=w914, f=w913) -> (s? t:f=w912:string)
                }
                frame "True", Default {
                  n264 = Bundle By Name(cluster=w922, "Control.Control Type"=T16."Speed [RPM]") -> (w925:T26)
                  n265 = Obtain Queue(name (unnamed)="FRENI", element data type=T8 {"Message"="", "Message Data"=variant} ("Message Cluster")) -> (queue out=w929:refnum<queue>)  [unwired: 3 in, 2 out]
                  n266 = Bundle By Name(cluster=cluster{"Status":string, "variant":variant} {"Status"="AGGIORNA COMANDI FRENO", "variant"=variant}, "variant"=w925) -> (w926:cluster{"Status":string, "variant":variant})
                  n267 = Enqueue Element(queue=w929, element=w926) -> ()  [unwired: 2 in, 3 out]
                }
              }
              n268 = local write "Stato"(w906) -> ()
            }
          }
          frame "FRENO SET SENSO ROTAZIONE" {
            n269 = while {
              tunnel: [w944] -> w933
              tunnel: w934 -> [w943]
              shift-right: [w940] -> _
              shift-left: _ -> [w939]
              tunnel: w935 -> [w938]
              tunnel: w932 -> [w937]
              stop <- TRUE stop-if-true
              n270 = local read "Stato"() -> (w942:string)
              n271 = case shown="\"wait\"" w942 {
                selector: w942 -> [w955 _]
                tunnel: [w954 "wait"] -> w941
                tunnel: [w946 _] -> w944
                tunnel: w943 -> [_ _]
                tunnel: [_ TRUE] -> w940
                tunnel: w939 -> [w947 _]
                tunnel: w938 -> [_ _]
                tunnel: w937 -> [w951 w959]
                frame "wait" {
                  n272 = global read "Global_All_Data.vi" "All Data"() -> (w952:T34)
                  n273 = Unbundle By Name(w952) -> ("MISURE ALL.STATO PLC 1.USCITE PLC.DO (bit).Senso rotazione"=w949:bool)
                  n274 = Unbundle By Name(w951) -> ("SENSO DI ROTAZIONE"=w950:bool)
                  n275 = call "Elapsed Time7"("Time Target (s)"=5.0, "Reset"=w947, "Auto Reset"=FALSE) -> ("Time has Elapsed"=w948:bool)  [unwired: 9 in, 7 out]
                  n276 = Equal?(x=w950, y=w949) -> (x = y?=w946:bool)
                  n277 = Select(t="Default", s=w948, f=w955) -> (s? t:f=w954:string)
                }
                frame "True", Default {
                  n278 = Unbundle By Name(w959) -> ("SENSO DI ROTAZIONE"=w958:bool)
                  n279 = case shown="True" w958 {
                    frame False {
                      n280 = call "Set DO.vi"("Cluster SET DO"=T13 [{"DO"=enum."*Senso rot freno 1", "Value"=FALSE}]) -> ()  [unwired: 10 in, 1 out]
                    }
                    frame True {
                      n281 = call "Set DO.vi"("Cluster SET DO"=T13 [{"DO"=enum."*Senso rot freno 1", "Value"=TRUE}]) -> ()  [unwired: 10 in, 1 out]
                    }
                  }
                }
              }
              n282 = local write "Stato"(w941) -> ()
            }
          }
          frame "FRENO SET SENS ROT SEGNO COPPIA" {
            n283 = while {
              shift-right: [w972] -> _
              shift-left: _ -> [w971]
              shift-right: [w970] -> _
              shift-left: _ -> [w969]
              shift-right: [w968] -> _
              shift-left: _ -> [w967]
              tunnel: [w966] -> w964
              stop <- TRUE stop-if-true
              n284 = local read "Stato"() -> (w974:string)
              n285 = case shown="\"Leggi segno coppia\"" w974 {
                selector: w974 -> [w988 _ w1000 _]
                tunnel: [w987 "Leggi segno coppia" ("t") w999 "wait" ("t")] -> w973
                tunnel: [_ _ TRUE TRUE] -> w972
                tunnel: w971 -> [w976 _ _ _]
                tunnel: [w984 FALSE w997 w1009] -> w970
                tunnel: w969 -> [w984 _ _ w1009]
                tunnel: [_ TRUE _ _] -> w968
                tunnel: w967 -> [_ _ w1003 _]
                tunnel: [w978 _ _ _] -> w966
                frame "wait" {
                  n286 = global read "Global_All_Data.vi" "All Data"() -> (w985:T34)
                  n287 = Unbundle By Name(w985) -> ("MISURE ALL.STATO PLC 1.USCITE PLC.DO (bit).Senso rotazione"=w983:bool)
                  n288 = call "Elapsed Time18"("Time Target (s)"=5.0, "Reset"=w976, "Auto Reset"=FALSE) -> ("Time has Elapsed"=w989:bool)  [unwired: 9 in, 7 out]
                  n289 = Select(t="Default", s=w989, f=w988) -> (s? t:f=w987:string)
                  n290 = Equal?(x=w984, y=w983) -> (x = y?=w980:bool)
                  n291 = Not(x=w980) -> (.not. x?=w979:bool)
                  n292 = Or(x=w976, y=w979) -> (x .or. y?=w977:bool)
                  n293 = call "Elapsed Time20"("Time Target (s)"=3.0, "Reset"=w977, "Auto Reset"=FALSE) -> ("Time has Elapsed"=w978:bool)  [unwired: 9 in, 7 out]
                }
                frame "True", Default {
                }
                frame "Leggi segno coppia" {
                  # "SENSO ROTAZIONE"
                  # "ai coppia"
                  n294 = global read "Global_All_Data.vi" "All Data"() -> (w1005:T34)
                  n295 = Unbundle By Name(w1005) -> ("MISURE ALL.Cluster READ NI.AI (0-10V).AI 0"=w1006:dbl)
                  n296 = call "Elapsed Time19"("Time Target (s)"=2.0, "Reset"=w1003) -> ("Time has Elapsed"=w1001:bool)  [unwired: 10 in, 7 out]
                  n297 = Greater Or Equal To 0?(x=w1006) -> (x >= 0?=w998:bool)
                  n298 = Select(t="Set senso rot coppia", s=w1001, f=w1000) -> (s? t:f=w999:string)
                  n299 = Select(t=FALSE, s=w998, f=TRUE) -> (s? t:f=w997:bool)
                }
                frame "Set senso rot coppia" {
                  n300 = case shown="True" w1009 {
                    frame False {
                      n301 = call "Set DO.vi"("Cluster SET DO"=T13 [{"DO"=enum."*Senso rot freno 1", "Value"=FALSE}]) -> ()  [unwired: 10 in, 1 out]
                    }
                    frame True {
                      n302 = call "Set DO.vi"("Cluster SET DO"=T13 [{"DO"=enum."*Senso rot freno 1", "Value"=TRUE}]) -> ()  [unwired: 10 in, 1 out]
                    }
                  }
                }
              }
              n303 = local write "Stato"(w973) -> ()
            }
          }
          frame "FRENO CONFIG" {
            # "imposta prima il tipo di controllo e poi il setpoint"
            n304 = local read "Data"() -> (w1014:T2)
            n305 = while {
              tunnel: [w1025] -> w1013
              tunnel: w1015 -> [w1024]
              shift-right: [w1021] -> _
              shift-left: _ -> [w1020]
              tunnel: w1016 -> [w1019]
              tunnel: w1014 -> [w1018]
              stop <- TRUE stop-if-true
              n306 = local read "Stato"() -> (w1023:string)
              n307 = case shown="\"Attendi setpoint\"" w1023 {
                selector: w1023 -> [_ _ w1044 _ w1077 w1083]
                tunnel: ["Set tipo controllo" "Attendi tipo controllo" ("t") w1041 "Attendi setpoint" ("t") w1075 w1083] -> w1022
                tunnel: [_ _ _ _ _ TRUE] -> w1025
                tunnel: w1024 -> [_ _ w1049 _ _ _]
                tunnel: [TRUE TRUE _ TRUE _ _] -> w1021
                tunnel: w1020 -> [_ _ w1046 _ w1074 _]
                tunnel: w1019 -> [_ w1033 _ w1058 w1073 _]
                tunnel: w1018 -> [_ w1032 w1048 w1057 w1072 _]
                frame "True", Default {
                }
                frame "Set tipo controllo" {
                  n308 = Unbundle By Name(w1032) -> ("Control Type"=w1031:T16)
                  n309 = Bundle By Name(cluster=w1033, "Control.Control Type"=w1031) -> (w1034:T26)
                  n310 = Obtain Queue(name (unnamed)="FRENI", element data type=T8 {"Message"="", "Message Data"=variant} ("Message Cluster")) -> (queue out=w1038:refnum<queue>)  [unwired: 3 in, 2 out]
                  n311 = Bundle By Name(cluster=cluster{"Status":string, "variant":variant} {"Status"="AGGIORNA COMANDI FRENO", "variant"=variant}, "variant"=w1034) -> (w1035:cluster{"Status":string, "variant":variant})
                  n312 = Enqueue Element(queue=w1038, element=w1035) -> ()  [unwired: 2 in, 3 out]
                }
                frame "Attendi tipo controllo" {
                  n313 = Unbundle By Name(w1049) -> ("Controllo desiderato"=w1053:T16)
                  n314 = Unbundle By Name(w1048) -> ("Control Type"=w1047:T16)
                  n315 = call "Elapsed Time24"("Time Target (s)"=5.0, "Reset"=w1046, "Auto Reset"=FALSE) -> ("Time has Elapsed"=w1042:bool)  [unwired: 9 in, 7 out]
                  n316 = Equal?(x=w1053, y=w1047) -> (x = y?=w1045:bool)
                  n317 = Select(t="Imposta setpoint", s=w1045, f=w1044) -> (s? t:f=w1043:string)
                  n318 = Select(t="Set tipo controllo", s=w1042, f=w1043) -> (s? t:f=w1041:string)
                }
                frame "Imposta setpoint" {
                  n319 = Unbundle By Name(w1057) -> ("Set"=w1056:dbl)
                  n320 = Bundle By Name(cluster=w1058, "Control.Set"=w1056) -> (w1059:T26)
                  n321 = Obtain Queue(name (unnamed)="FRENI", element data type=T8 {"Message"="", "Message Data"=variant} ("Message Cluster")) -> (queue out=w1063:refnum<queue>)  [unwired: 3 in, 2 out]
                  n322 = Bundle By Name(cluster=cluster{"Status":string, "variant":variant} {"Status"="AGGIORNA COMANDI FRENO", "variant"=variant}, "variant"=w1059) -> (w1060:cluster{"Status":string, "variant":variant})
                  n323 = Enqueue Element(queue=w1063, element=w1060) -> ()  [unwired: 2 in, 3 out]
                }
                frame "Attendi setpoint" {
                  n324 = Unbundle By Name(w1073) -> ("Control.Set"=w1071:dbl)
                  n325 = Unbundle By Name(w1072) -> ("Set"=w1068:dbl)
                  n326 = call "Elapsed Time25"("Time Target (s)"=5.0, "Reset"=w1074, "Auto Reset"=FALSE) -> ("Time has Elapsed"=w1078:bool)  [unwired: 9 in, 7 out]
                  n327 = Multiply(x=w1068, y=0.9) -> (x*y=w1067:dbl)
                  n328 = Multiply(x=w1068, y=1.1) -> (x*y=w1069:dbl)
                  n329 = In Range and Coerce(upper limit=w1069, x=w1071, lower limit=w1067) -> (In Range?=w1065:bool)  [unwired: 1 out]
                  n330 = Select(t="Fine", s=w1065, f=w1077) -> (s? t:f=w1079:string)
                  n331 = Select(t="Imposta setpoint", s=w1078, f=w1079) -> (s? t:f=w1075:string)
                }
                frame "Fine" {
                }
              }
              n332 = local write "Stato"(w1022) -> ()
            }
          }
          frame "ALIMENTATORE 1 MARCIA ON" {
            n333 = while {
              tunnel: [w1093] -> w1085
              shift-right: [w1090] -> _
              shift-left: _ -> [w1089]
              tunnel: w1086 -> [w1088]
              stop <- TRUE stop-if-true
              n334 = local read "Stato"() -> (w1092:string)
              n335 = case shown="\"wait\"" w1092 {
                selector: w1092 -> [w1099 _]
                tunnel: [w1098 "wait"] -> w1091
                tunnel: [w1096 _] -> w1093
                tunnel: [_ TRUE] -> w1090
                tunnel: w1089 -> [w1103 _]
                tunnel: w1088 -> [w1095 w1107]
                frame "wait" {
                  n336 = Unbundle By Name(w1095) -> ("In marcia"=w1096:bool)
                  n337 = call "Elapsed Time8"("Time Target (s)"=5.0, "Reset"=w1103, "Auto Reset"=FALSE) -> ("Time has Elapsed"=w1100:bool)  [unwired: 9 in, 7 out]
                  n338 = Select(t="Default", s=w1100, f=w1099) -> (s? t:f=w1098:string)
                }
                frame "True", Default {
                  n339 = Unbundle By Name(w1107) -> ("Alimentatore 1"=w1105:T27)
                  n340 = Bundle By Name(cluster=w1105, "Start\\stop.Start"=TRUE ("Alimentatore 1.Command.Start"), "Start\\stop.Stop"=FALSE ("Command.Stop")) -> (w1108:T27)
                  n341 = Obtain Queue(name (unnamed)="ALIMENTATORE 1", element data type=T8 {"Message"="", "Message Data"=variant} ("Message Cluster")) -> (queue out=w1110:refnum<queue>)  [unwired: 3 in, 2 out]
                  n342 = Bundle By Name(cluster=cluster{"Status":string, "variant":variant} {"Status"="AGGIORNA COMANDI ALIMENTATORE", "variant"=variant}, "variant"=w1108) -> (w1113:cluster{"Status":string, "variant":variant})
                  n343 = Enqueue Element(queue=w1110, element=w1113) -> ()  [unwired: 2 in, 3 out]
                }
              }
              n344 = local write "Stato"(w1091) -> ()
            }
          }
          frame "ALIMENTATORE 1 ABILITA" {
            n345 = while {
              tunnel: [w1124] -> w1116
              shift-right: [w1121] -> _
              shift-left: _ -> [w1120]
              tunnel: w1117 -> [w1119]
              stop <- TRUE stop-if-true
              n346 = local read "Stato"() -> (w1123:string)
              n347 = case shown="\"True\", Default" w1123 {
                selector: w1123 -> [w1130 _]
                tunnel: [w1129 "wait"] -> w1122
                tunnel: [w1127 _] -> w1124
                tunnel: [_ TRUE] -> w1121
                tunnel: w1120 -> [w1134 _]
                tunnel: w1119 -> [w1126 w1137]
                frame "wait" {
                  n348 = Unbundle By Name(w1126) -> ("Abilitato"=w1127:bool)
                  n349 = call "Elapsed Time16"("Time Target (s)"=5.0, "Reset"=w1134, "Auto Reset"=FALSE) -> ("Time has Elapsed"=w1131:bool)  [unwired: 9 in, 7 out]
                  n350 = Select(t="Default", s=w1131, f=w1130) -> (s? t:f=w1129:string)
                }
                frame "True", Default {
                  n351 = Unbundle By Name(w1137) -> ("Alimentatore 1"=w1135:T27)
                  n352 = Bundle By Name(cluster=w1135, "Abilita.Abilita"=TRUE ("Alimentatore 1.Command.Start")) -> (w1138:T27)
                  n353 = Obtain Queue(name (unnamed)="ALIMENTATORE 1", element data type=T8 {"Message"="", "Message Data"=variant} ("Message Cluster")) -> (queue out=w1140:refnum<queue>)  [unwired: 3 in, 2 out]
                  n354 = Bundle By Name(cluster=cluster{"Status":string, "variant":variant} {"Status"="AGGIORNA COMANDI ALIMENTATORE", "variant"=variant}, "variant"=w1138) -> (w1143:cluster{"Status":string, "variant":variant})
                  n355 = Enqueue Element(queue=w1140, element=w1143) -> ()  [unwired: 2 in, 3 out]
                }
              }
              n356 = local write "Stato"(w1122) -> ()
            }
          }
          frame "ALIMENTATORE 1 DISABILITA" {
            n357 = while {
              tunnel: [w1154] -> w1146
              shift-right: [w1151] -> _
              shift-left: _ -> [w1150]
              tunnel: w1147 -> [w1149]
              stop <- TRUE stop-if-true
              n358 = local read "Stato"() -> (w1153:string)
              n359 = case shown="\"wait\"" w1153 {
                selector: w1153 -> [w1161 _]
                tunnel: [w1160 "wait"] -> w1152
                tunnel: [w1156 _] -> w1154
                tunnel: [_ TRUE] -> w1151
                tunnel: w1150 -> [w1165 _]
                tunnel: w1149 -> [w1157 w1168]
                frame "wait" {
                  n360 = Unbundle By Name(w1157) -> ("Abilitato"=w1158:bool)
                  n361 = call "Elapsed Time17"("Time Target (s)"=5.0, "Reset"=w1165, "Auto Reset"=FALSE) -> ("Time has Elapsed"=w1162:bool)  [unwired: 9 in, 7 out]
                  n362 = Not(x=w1158) -> (.not. x?=w1156:bool)
                  n363 = Select(t="Default", s=w1162, f=w1161) -> (s? t:f=w1160:string)
                }
                frame "True", Default {
                  n364 = Unbundle By Name(w1168) -> ("Alimentatore 1"=w1166:T27)
                  n365 = Bundle By Name(cluster=w1166, "Abilita.Abilita"=FALSE ("Alimentatore 1.Command.Start")) -> (w1169:T27)
                  n366 = Obtain Queue(name (unnamed)="ALIMENTATORE 1", element data type=T8 {"Message"="", "Message Data"=variant} ("Message Cluster")) -> (queue out=w1171:refnum<queue>)  [unwired: 3 in, 2 out]
                  n367 = Bundle By Name(cluster=cluster{"Status":string, "variant":variant} {"Status"="AGGIORNA COMANDI ALIMENTATORE", "variant"=variant}, "variant"=w1169) -> (w1174:cluster{"Status":string, "variant":variant})
                  n368 = Enqueue Element(queue=w1171, element=w1174) -> ()  [unwired: 2 in, 3 out]
                }
              }
              n369 = local write "Stato"(w1152) -> ()
            }
          }
          frame "ALIMENTATORE 1 MARCIA OFF" {
            n370 = while {
              tunnel: [w1185] -> w1177
              shift-right: [w1182] -> _
              shift-left: _ -> [w1181]
              tunnel: w1178 -> [w1180]
              stop <- TRUE stop-if-true
              n371 = local read "Stato"() -> (w1184:string)
              n372 = case shown="\"wait\"" w1184 {
                selector: w1184 -> [w1192 _]
                tunnel: [w1191 "wait"] -> w1183
                tunnel: [w1187 _] -> w1185
                tunnel: [_ TRUE] -> w1182
                tunnel: w1181 -> [w1196 _]
                tunnel: w1180 -> [w1188 w1200]
                frame "wait" {
                  n373 = Unbundle By Name(w1188) -> ("In marcia"=w1189:bool)
                  n374 = call "Elapsed Time9"("Time Target (s)"=5.0, "Reset"=w1196, "Auto Reset"=FALSE) -> ("Time has Elapsed"=w1193:bool)  [unwired: 9 in, 7 out]
                  n375 = Not(x=w1189) -> (.not. x?=w1187:bool)
                  n376 = Select(t="Default", s=w1193, f=w1192) -> (s? t:f=w1191:string)
                }
                frame "True", Default {
                  n377 = Unbundle By Name(w1200) -> ("Alimentatore 1"=w1198:T27)
                  n378 = Bundle By Name(cluster=w1198, "Start\\stop.Start"=FALSE ("Alimentatore 1.Command.Start"), "Start\\stop.Stop"=TRUE ("Command.Stop")) -> (w1201:T27)
                  n379 = Obtain Queue(name (unnamed)="ALIMENTATORE 1", element data type=T8 {"Message"="", "Message Data"=variant} ("Message Cluster")) -> (queue out=w1203:refnum<queue>)  [unwired: 3 in, 2 out]
                  n380 = Bundle By Name(cluster=cluster{"Status":string, "variant":variant} {"Status"="AGGIORNA COMANDI ALIMENTATORE", "variant"=variant}, "variant"=w1201) -> (w1206:cluster{"Status":string, "variant":variant})
                  n381 = Enqueue Element(queue=w1203, element=w1206) -> ()  [unwired: 2 in, 3 out]
                }
              }
              n382 = local write "Stato"(w1183) -> ()
            }
          }
          frame "FRENO FORZA RIF A 0" {
            n383 = flat-sequence {
              frame #0 {
                n384 = global write "Global Trampa 0.vi" "Forza rif"(TRUE ("Rampa a 0")) -> ()
              }
              frame #1 {
                n385 = call "SET AO.vi"("Cluster SET AO"=T17 [{"AO"=enum."RIF COPPIA FRENO 1", "Value"=0.0}, {"AO"=enum."RIF COPPIA FRENO 2", "Value"=0.0}]) -> ()  [unwired: 10 in, 1 out]
              }
              frame #2 {
                n386 = Wait (ms)(milliseconds to wait=u32 100) -> ()  [unwired: 1 out]
              }
              frame #3 {
                n387 = call "SET AO.vi"("Cluster SET AO"=T17 [{"AO"=enum."RIF VEL FRENO 1", "Value"=0.0}, {"AO"=enum."RIF VEL FRENO 2", "Value"=0.0}]) -> ()  [unwired: 10 in, 1 out]
              }
              frame #4 {
                n388 = Wait (ms)(milliseconds to wait=u32 100) -> ()  [unwired: 1 out]
              }
            }
          }
          frame "ALIMENTATORE 1 SET RIF" {
            n389 = Unbundle By Name(w1220) -> ("V avvio[V]"=w1218:dbl, "F avvio[Hz]"=w1217:dbl)
            n390 = while {
              tunnel: [w1227] -> w1216
              tunnel: w1219 -> [w1224]
              tunnel: w1218 -> [w1223]
              tunnel: w1217 -> [w1222]
              stop <- TRUE stop-if-true
              n391 = local read "Stato"() -> (w1226:string)
              n392 = case shown="\"True\", Default" w1226 {
                selector: w1226 -> [w1232 _]
                tunnel: [w1232 "wait"] -> w1225
                tunnel: [w1231 _] -> w1227
                tunnel: w1224 -> [w1233 w1238]
                tunnel: w1223 -> [_ w1235]
                tunnel: w1222 -> [_ w1234]
                frame "wait" {
                  n393 = Unbundle By Name(w1233) -> ("Fine rampa RIF1"=w1230:bool, "Fine rampa RIF2"=w1229:bool)
                  n394 = And(x=w1230, y=w1229) -> (x .and. y?=w1231:bool)
                }
                frame "True", Default {
                  n395 = Unbundle By Name(w1238) -> ("Alimentatore 1"=w1236:T27)
                  n396 = Bundle By Name(cluster=w1236, "RIF 1"=w1235, "RIF 2"=w1234) -> (w1237:T27)
                  n397 = Obtain Queue(name (unnamed)="ALIMENTATORE 1", element data type=T8 {"Message"="", "Message Data"=variant} ("Message Cluster")) -> (queue out=w1240:refnum<queue>)  [unwired: 3 in, 2 out]
                  n398 = Bundle By Name(cluster=cluster{"Status":string, "variant":variant} {"Status"="AGGIORNA COMANDI ALIMENTATORE", "variant"=variant}, "variant"=w1237) -> (w1243:cluster{"Status":string, "variant":variant})
                  n399 = Enqueue Element(queue=w1240, element=w1243) -> ()  [unwired: 2 in, 3 out]
                }
              }
              n400 = local write "Stato"(w1225) -> ()
            }
          }
          frame "ALIMENTATORE 1 SET RIF RIDOTTO" {
            n401 = Unbundle By Name(w1253) -> ("V avvio[V]"=w1252:dbl, "%V ridotta"=w1251:dbl, "F avvio[Hz]"=w1246:dbl)
            n402 = Multiply(x=w1252, y=w1251) -> (x*y=w1250:dbl)
            n403 = Divide(x=w1250, y=100.0) -> (x/y=w1247:dbl)
            n404 = while {
              tunnel: [w1260] -> w1245
              tunnel: w1248 -> [w1257]
              tunnel: w1247 -> [w1256]
              tunnel: w1246 -> [w1255]
              stop <- TRUE stop-if-true
              n405 = local read "Stato"() -> (w1259:string)
              n406 = case shown="\"True\", Default" w1259 {
                selector: w1259 -> [w1265 _]
                tunnel: [w1265 "wait"] -> w1258
                tunnel: [w1264 _] -> w1260
                tunnel: w1257 -> [w1266 w1271]
                tunnel: w1256 -> [_ w1268]
                tunnel: w1255 -> [_ w1267]
                frame "wait" {
                  n407 = Unbundle By Name(w1266) -> ("Fine rampa RIF1"=w1263:bool, "Fine rampa RIF2"=w1262:bool)
                  n408 = And(x=w1263, y=w1262) -> (x .and. y?=w1264:bool)
                }
                frame "True", Default {
                  n409 = Unbundle By Name(w1271) -> ("Alimentatore 1"=w1269:T27)
                  n410 = Bundle By Name(cluster=w1269, "RIF 1"=w1268, "RIF 2"=w1267) -> (w1270:T27)
                  n411 = Obtain Queue(name (unnamed)="ALIMENTATORE 1", element data type=T8 {"Message"="", "Message Data"=variant} ("Message Cluster")) -> (queue out=w1273:refnum<queue>)  [unwired: 3 in, 2 out]
                  n412 = Bundle By Name(cluster=cluster{"Status":string, "variant":variant} {"Status"="AGGIORNA COMANDI ALIMENTATORE", "variant"=variant}, "variant"=w1270) -> (w1276:cluster{"Status":string, "variant":variant})
                  n413 = Enqueue Element(queue=w1273, element=w1276) -> ()  [unwired: 2 in, 3 out]
                }
              }
              n414 = local write "Stato"(w1258) -> ()
            }
          }
          frame "ALIMENTATORE 1 SET RIF A 0" {
            n415 = while {
              tunnel: [w1284] -> w1278
              tunnel: w1279 -> [w1281]
              stop <- TRUE stop-if-true
              n416 = local read "Stato"() -> (w1283:string)
              n417 = case shown="\"wait\"" w1283 {
                selector: w1283 -> [w1293 _ _]
                tunnel: [w1293 "wait1" "wait"] -> w1282
                tunnel: [w1286 _ _] -> w1284
                tunnel: w1281 -> [w1294 w1298 _]
                frame "wait" {
                  n418 = Unbundle By Name(w1294) -> ("Fine rampa RIF1"=w1292:bool, "Fine rampa RIF2"=w1291:bool)
                  n419 = And(x=w1292, y=w1291) -> (x .and. y?=w1290:bool)
                  n420 = Not(x=w1290) -> (.not. x?=w1289:bool)
                  n421 = call "Elapsed Time22"("Time Target (s)"=2.0, "Reset"=w1289, "Auto Reset"=FALSE) -> ("Time has Elapsed"=w1286:bool)  [unwired: 9 in, 7 out]
                }
                frame "True", Default {
                  w1295 = 0.0 ("Voltage [V]")
                  n422 = Unbundle By Name(w1298) -> ("Alimentatore 1"=w1296:T27)
                  n423 = Bundle By Name(cluster=w1296, "RIF 1"=w1295, "RIF 2"=w1295) -> (w1297:T27)
                  n424 = Obtain Queue(name (unnamed)="ALIMENTATORE 1", element data type=T8 {"Message"="", "Message Data"=variant} ("Message Cluster")) -> (queue out=w1300:refnum<queue>)  [unwired: 3 in, 2 out]
                  n425 = Bundle By Name(cluster=cluster{"Status":string, "variant":variant} {"Status"="AGGIORNA COMANDI ALIMENTATORE", "variant"=variant}, "variant"=w1297) -> (w1303:cluster{"Status":string, "variant":variant})
                  n426 = Enqueue Element(queue=w1300, element=w1303) -> ()  [unwired: 2 in, 3 out]
                }
                frame "wait1" {
                  n427 = Wait (ms)(milliseconds to wait=u32 1000) -> ()  [unwired: 1 out]
                }
              }
              n428 = local write "Stato"(w1282) -> ()
            }
          }
          frame "ALIMENTATORE 1 RESET ALLARMI" {
            n429 = local read "Stato"() -> (w1309:string)
            n430 = while {
              tunnel: w1309 -> [w1313]
              tunnel: [w1312] -> w1308
              tunnel: [w1311] -> w1307
              stop <- TRUE stop-if-true
              n431 = case shown="\"Wait\"" w1313 {
                selector: w1313 -> [_ _ w1320]
                tunnel: ["Wait" "Reset off" w1320] -> w1312
                tunnel: [_ _ TRUE] -> w1311
                frame "Reset on", Default {
                  n432 = call "Set DO.vi"("Cluster SET DO"=T13 [{"DO"=enum."*Reset allarmi", "Value"=TRUE}]) -> ()  [unwired: 10 in, 1 out]
                }
                frame "Wait" {
                  n433 = Wait (ms)(milliseconds to wait=u32 1000) -> ()  [unwired: 1 out]
                }
                frame "Reset off" {
                  n434 = call "Set DO.vi"("Cluster SET DO"=T13 [{"DO"=enum."*Reset allarmi", "Value"=FALSE}]) -> ()  [unwired: 10 in, 1 out]
                }
              }
            }
            n435 = local write "Stato"(w1308) -> ()
          }
          frame "ALIMENTATORE 1 SCORTA 2" {
          }
          frame "ALIMENTATORE 1 SCORTA 3" {
          }
          frame "TELERUTTORI CHIUDI POTENZA" {
            n436 = local read "Stato"() -> (w1326:string)
            n437 = call "Procedura abilitazione potenza.vi"("All Data"=w1327, "Impostazioni elettriche in"=w1329, "Stato"=w1326) -> ("This VI"=→"Vi chiudi teler pot":refnum<vi>, "Fine step"=w1328:bool, "stato out"=w1325:string)  [unwired: 6 in]
            n438 = local write "Stato"(w1325) -> ()
          }
          frame "TELERUTTORI APRI POTENZA" {
            n439 = Unbundle By Name(w1336) -> ("COLLEGAMENTO"=w1339:T10, "LINEA ELETTRICA"=w1337:T62)
            n440 = Unbundle By Name(w1335) -> ("MISURE ALL.INTERFACCIA.DI (logici)"=w1338:T63)
            n441 = while {
              shift-right: [w1348] -> _
              shift-left: _ -> [w1347]
              tunnel: w1339 -> [w1346]
              tunnel: w1338 -> [w1345]
              tunnel: w1337 -> [w1344]
              tunnel: [w1343] -> w1334
              tunnel: w1332 -> [w1342]
              tunnel: w1331 -> [w1341]
              stop <- TRUE stop-if-true
              n442 = local read "Stato"() -> (w1350:string)
              n443 = case shown="\"impulso\"" w1350 {
                selector: w1350 -> [_ w1376 _ w1413 w1446 w1449]
                tunnel: ["impulso" w1375 "wait" ("t") w1416 w1446 w1449] -> w1349
                tunnel: [TRUE _ TRUE _ _ _] -> w1348
                tunnel: w1347 -> [_ w1379 _ w1422 _ _]
                tunnel: w1346 -> [w1355 _ w1390 w1418 _ _]
                tunnel: w1345 -> [_ _ _ w1410 _ _]
                tunnel: w1344 -> [_ _ _ _ _ _]
                tunnel: [_ _ _ _ TRUE TRUE] -> w1343
                tunnel: w1342 -> [w1354 _ _ _ _ _]
                tunnel: w1341 -> [_ _ w1381 _ _ _]
                frame "True", Default {
                  n444 = case shown="\"AC TRIFASE + FRENO\"" w1355 {
                    frame "AC TRIFASE + FRENO" {
                      n445 = call "Set DO.vi"("Cluster SET DO"=T13 [{"DO"=enum."*Stop potenza AC", "Value"=TRUE}]) -> ()  [unwired: 10 in, 1 out]
                    }
                    frame "AC TRIFASE" {
                      n446 = call "Set DO.vi"("Cluster SET DO"=T13 [{"DO"=enum."*Stop potenza AC", "Value"=TRUE}]) -> ()  [unwired: 10 in, 1 out]
                    }
                    frame "DC CON ECCITAZIONE" {
                      n447 = call "Set DO.vi"("Cluster SET DO"=T13 [{"DO"=enum."*Stop potenza DC", "Value"=TRUE}]) -> ()  [unwired: 10 in, 1 out]
                    }
                    frame "DC CON ECCITAZIONE + FRENO" {
                      n448 = call "Set DO.vi"("Cluster SET DO"=T13 [{"DO"=enum."*Stop potenza DC", "Value"=TRUE}]) -> ()  [unwired: 10 in, 1 out]
                    }
                    frame "AC MONOFASE" {
                      n449 = call "Set DO.vi"("Cluster SET DO"=T13 [{"DO"=enum."*Stop potenza AC", "Value"=TRUE}]) -> ()  [unwired: 10 in, 1 out]
                    }
                    frame "SOLO FRENO" {
                      n450 = call "Set DO.vi"("Cluster SET DO"=T13 [{"DO"=enum."*Stop potenza AC", "Value"=TRUE}]) -> ()  [unwired: 10 in, 1 out]
                    }
                    frame "CARICO RESISTIVO" {
                    }
                    frame "GENERICO" {
                      n451 = call "Set DO.vi"("Cluster SET DO"=T13 [{"DO"=enum."*Stop potenza AC", "Value"=TRUE}]) -> ()  [unwired: 10 in, 1 out]
                    }
                    frame "SOLO ACQUISITORE" {
                    }
                    frame "SCORTA 4" {
                    }
                    frame "SCORTA 5" {
                    }
                    frame "SCORTA 6" {
                    }
                    frame "DC NO ECCITAZIONE" {
                      n452 = call "Set DO.vi"("Cluster SET DO"=T13 [{"DO"=enum."*Stop potenza DC", "Value"=TRUE}]) -> ()  [unwired: 10 in, 1 out]
                    }
                    frame "DC NO ECCITAZIONE + FRENO" {
                      n453 = call "Set DO.vi"("Cluster SET DO"=T13 [{"DO"=enum."*Stop potenza DC", "Value"=TRUE}]) -> ()  [unwired: 10 in, 1 out]
                    }
                    frame "FRENO TRASC + AFE" {
                      n454 = call "Set DO.vi"("Cluster SET DO"=T13 [{"DO"=enum."Apri potenza AFE", "Value"=TRUE}]) -> ()  [unwired: 10 in, 1 out]
                    }
                  }
                  n455 = Bundle By Name(cluster=w1354, "Abilita.Abilita"=FALSE ("Stato comandi freno.Abilita.Abilita")) -> (w1358:T26)
                  n456 = Bundle By Name(cluster=cluster{"Status":string, "variant":variant} {"Status"="AGGIORNA COMANDI FRENO", "variant"=variant}, "variant"=w1358) -> (w1361:cluster{"Status":string, "variant":variant})
                  n457 = Obtain Queue(name (unnamed)="FRENI", element data type=T8 {"Message"="", "Message Data"=variant} ("Message Cluster")) -> (queue out=w1353:refnum<queue>)  [unwired: 3 in, 2 out]
                  n458 = Flush Queue(queue=w1353) -> (queue out=w1352:refnum<queue>)  [unwired: 1 in, 2 out]
                  n459 = Enqueue Element(queue=w1352, element=w1361) -> ()  [unwired: 2 in, 3 out]
                }
                frame "impulso" {
                  n460 = call "Elapsed Time12"("Time Target (s)"=1.0, "Reset"=w1379, "Auto Reset"=FALSE) -> ("Time has Elapsed"=w1377:bool)  [unwired: 9 in, 7 out]
                  n461 = Select(t="Stop potenza 2", s=w1377, f=w1376) -> (s? t:f=w1375:string)
                }
                frame "Stop potenza 2" {
                  n462 = case shown="\"AC TRIFASE + FRENO\"" w1390 {
                    frame "AC TRIFASE + FRENO" {
                      n463 = call "Set DO.vi"("Cluster SET DO"=T13 [{"DO"=enum."*Stop potenza AC", "Value"=FALSE}]) -> ()  [unwired: 10 in, 1 out]
                    }
                    frame "AC TRIFASE" {
                      n464 = call "Set DO.vi"("Cluster SET DO"=T13 [{"DO"=enum."*Stop potenza AC", "Value"=FALSE}]) -> ()  [unwired: 10 in, 1 out]
                    }
                    frame "DC CON ECCITAZIONE" {
                      n465 = call "Set DO.vi"("Cluster SET DO"=T13 [{"DO"=enum."*Stop potenza DC", "Value"=FALSE}]) -> ()  [unwired: 10 in, 1 out]
                    }
                    frame "DC CON ECCITAZIONE + FRENO" {
                      n466 = call "Set DO.vi"("Cluster SET DO"=T13 [{"DO"=enum."*Stop potenza DC", "Value"=FALSE}]) -> ()  [unwired: 10 in, 1 out]
                    }
                    frame "AC MONOFASE" {
                      n467 = call "Set DO.vi"("Cluster SET DO"=T13 [{"DO"=enum."*Stop potenza AC", "Value"=FALSE}]) -> ()  [unwired: 10 in, 1 out]
                    }
                    frame "SOLO FRENO" {
                      n468 = call "Set DO.vi"("Cluster SET DO"=T13 [{"DO"=enum."*Stop potenza AC", "Value"=FALSE}]) -> ()  [unwired: 10 in, 1 out]
                    }
                    frame "CARICO RESISTIVO" {
                    }
                    frame "GENERICO" {
                      n469 = call "Set DO.vi"("Cluster SET DO"=T13 [{"DO"=enum."*Stop potenza AC", "Value"=FALSE}]) -> ()  [unwired: 10 in, 1 out]
                    }
                    frame "SOLO ACQUISITORE" {
                    }
                    frame "SCORTA 4" {
                    }
                    frame "SCORTA 5" {
                    }
                    frame "SCORTA 6" {
                    }
                    frame "DC NO ECCITAZIONE" {
                      n470 = call "Set DO.vi"("Cluster SET DO"=T13 [{"DO"=enum."*Stop potenza DC", "Value"=FALSE}]) -> ()  [unwired: 10 in, 1 out]
                    }
                    frame "DC NO ECCITAZIONE + FRENO" {
                      n471 = call "Set DO.vi"("Cluster SET DO"=T13 [{"DO"=enum."*Stop potenza DC", "Value"=FALSE}]) -> ()  [unwired: 10 in, 1 out]
                    }
                    frame "FRENO TRASC + AFE" {
                      n472 = call "Set DO.vi"("Cluster SET DO"=T13 [{"DO"=enum."Apri potenza AFE", "Value"=FALSE}]) -> ()  [unwired: 10 in, 1 out]
                    }
                  }
                  n473 = Unbundle By Name(w1381) -> ("Alimentatore 1"=w1386:T27)
                  n474 = Bundle By Name(cluster=w1386, "Abilita.Abilita"=FALSE ("Alimentatore 1.Command.Start")) -> (w1387:T27)
                  n475 = Obtain Queue(name (unnamed)="ALIMENTATORE 1", element data type=T8 {"Message"="", "Message Data"=variant} ("Message Cluster")) -> (queue out=w1388:refnum<queue>)  [unwired: 3 in, 2 out]
                  n476 = Bundle By Name(cluster=cluster{"Status":string, "variant":variant} {"Status"="AGGIORNA COMANDI ALIMENTATORE", "variant"=variant}, "variant"=w1387) -> (w1389:cluster{"Status":string, "variant":variant})
                  n477 = Enqueue Element(queue=w1388, element=w1389) -> ()  [unwired: 2 in, 3 out]
                }
                frame "wait" {
                  n478 = case shown="\"AC TRIFASE + FRENO\"" w1418 {
                    tunnel: [w1424 w1426 w1428 w1430 w1431 w1433 w1435 w1437 _ _ _ _ w1439 w1441 w1443] -> w1417
                    tunnel: w1410 -> [w1423 w1425 w1427 w1429 w1432 w1434 w1436 w1438 _ _ _ _ w1440 w1442 w1444]
                    frame "AC TRIFASE + FRENO" {
                      n479 = Unbundle By Name(w1423) -> ("Start alimentazione AC"=w1424:bool)
                    }
                    frame "DC CON ECCITAZIONE" {
                      n480 = Unbundle By Name(w1425) -> ("Start alimentazione DC"=w1426:bool)
                    }
                    frame "DC CON ECCITAZIONE + FRENO" {
                      n481 = Unbundle By Name(w1427) -> ("Start alimentazione DC"=w1428:bool)
                    }
                    frame "AC TRIFASE" {
                      n482 = Unbundle By Name(w1429) -> ("Start alimentazione AC"=w1430:bool)
                    }
                    frame "AC MONOFASE" {
                      n483 = Unbundle By Name(w1432) -> ("Start alimentazione AC"=w1431:bool)
                    }
                    frame "SOLO FRENO" {
                      n484 = Unbundle By Name(w1434) -> ("DI (logici) aggiuntivi impianto.Solo freno abilitato"=w1433:bool)
                    }
                    frame "CARICO RESISTIVO" {
                      n485 = Unbundle By Name(w1436) -> ("DI (logici) aggiuntivi impianto.Carico resistivo abilitato"=w1435:bool)
                    }
                    frame "GENERICO" {
                      n486 = Unbundle By Name(w1438) -> ("Start alimentazione AC"=w1437:bool)
                    }
                    frame "SOLO ACQUISITORE" {
                    }
                    frame "SCORTA 4" {
                    }
                    frame "SCORTA 5" {
                    }
                    frame "SCORTA 6" {
                    }
                    frame "DC NO ECCITAZIONE" {
                      n487 = Unbundle By Name(w1440) -> ("Potenza DC abilitata"=w1439:bool)
                    }
                    frame "DC NO ECCITAZIONE + FRENO" {
                      n488 = Unbundle By Name(w1442) -> ("Potenza DC abilitata"=w1441:bool)
                    }
                    frame "FRENO TRASC + AFE" {
                      n489 = Unbundle By Name(w1444) -> ("DI (logici) aggiuntivi impianto.Start potenza AFE"=w1443:bool)
                    }
                  }
                  n490 = call "Elapsed Time13"("Time Target (s)"=5.0, "Reset"=w1422, "Auto Reset"=FALSE) -> ("Time has Elapsed"=w1414:bool)  [unwired: 9 in, 7 out]
                  n491 = Unbundle By Name(w1410) -> ("FRENO 1 abilitato"=w1409:bool, "FRENO 2 abilitato"=w1408:bool, "ALIM 1 abilitato"=w1407:bool, "ALIM 2 abilitato"=w1406:bool)
                  n492 = Select(t="KO", s=w1414, f=w1413) -> (s? t:f=w1412:string)
                  n493 = Compound Arithmetic op=OR(w1409, w1408, w1407, w1406) -> (w1405:bool)
                  n494 = Not(x=w1405) -> (.not. x?=w1403:bool)
                  n495 = Not(x=w1417) -> (.not. x?=w1415:bool)
                  n496 = And(x=w1403, y=w1415) -> (x .and. y?=w1404:bool)
                  n497 = Select(t="OK", s=w1404, f=w1412) -> (s? t:f=w1416:string)
                }
                frame "OK" {
                }
                frame "KO" {
                  n498 = global write "Global allarmi procedure.vi" "Allarme Start potenza"(TRUE ("Allarme Abilita potenza")) -> ()
                }
              }
              n499 = local write "Stato"(w1349) -> ()
            }
            n500 = global write "Global prova in corso.vi" "prova in corso?"(FALSE ("prova in corso?")) -> ()
          }
          frame "TELERUTTORI ABILITA POTENZA" {
            n501 = Unbundle By Name(w1453) -> ("banco selezionato"=w1452:i8)
            n502 = local read "Stato"() -> (w1451:string)
            n503 = case shown="1" w1452 {
              tunnel: w1457 -> [w1464 w1468]
              tunnel: w1456 -> [w1463 w1467]
              tunnel: [w1462 w1466] -> w1455
              tunnel: [w1461 w1465] -> w1454
              tunnel: w1451 -> [w1460 w1470]
              tunnel: [w1459 w1469] -> w1450
              frame 0, Default {
                n504 = call "procedura configura potenza.vi"("All Data"=w1463, "Impostazioni elettriche in"=w1464, "Stato"=w1460) -> ("This VI"=w1461:refnum<vi>, "Boolean"=w1462:bool, "t"=w1459:string)  [unwired: 6 in]
              }
              frame 1 {
                n505 = call "procedura configura potenza BANCO 2.vi"("All Data"=w1467, "Impostazioni elettriche in"=w1468, "Stato"=w1470) -> ("This VI"=w1465:refnum<vi>, "Boolean"=w1466:bool, "stato"=w1469:string)  [unwired: 6 in]
              }
            }
            "Vi abilita pot" <- w1454
            n506 = local write "Stato"(w1450) -> ()
          }
          frame "TELERUTTORI DISABILITA POTENZA" {
            n507 = Unbundle By Name(w1472) -> ("banco selezionato"=w1471:i8)
            n508 = case shown="1" w1471 {
              tunnel: w1474 -> [w1477 w1500]
              tunnel: [w1476 w1499] -> w1473
              frame 0, Default {
                n509 = while {
                  shift-right: [w1481] -> _
                  shift-left: "Disabilita" -> [w1482]
                  tunnel: w1477 -> [w1480]
                  tunnel: [w1479] -> w1476
                  stop <- TRUE stop-if-true
                  n510 = case shown="\"Attendi\"" w1482 {
                    selector: w1482 -> [w1489 w1496 _]
                    tunnel: [w1488 w1496 "Attendi"] -> w1481
                    tunnel: w1480 -> [w1494 _ _]
                    tunnel: [_ TRUE _] -> w1479
                    frame "Attendi" {
                      n511 = Unbundle By Name(w1494) -> ("MISURE ALL.INTERFACCIA.DI (logici).ALIM 1 abilitato"=w1493:bool, "MISURE ALL.INTERFACCIA.DI (logici).FRENO 1 abilitato"=w1492:bool, "MISURE ALL.INTERFACCIA.DI (logici).Potenza trifase abilitata"=w1491:bool, "MISURE ALL.INTERFACCIA.DI (logici).Teleruttore WT abilitato"=w1486:bool, "MISURE ALL.INTERFACCIA.DI (logici).FRENO 2 abilitato"=w1485:bool, "MISURE ALL.INTERFACCIA.DI (logici).ALIM 1 abilitato"=w1484:bool)
                      n512 = Compound Arithmetic op=OR(w1493, w1492, w1491, w1486, w1485, w1484) -> (w1490:bool)
                      n513 = Select(t=w1489, s=w1490, f="Fine") -> (s? t:f=w1488:string)
                    }
                    frame "Fine" {
                    }
                    frame "Disabilita", Default {
                      n514 = call "Set DO.vi"("Cluster SET DO"=T13 [{"DO"=enum."B1 Seleziona linea 1", "Value"=FALSE}, {"DO"=enum."B1 Seleziona linea 2", "Value"=FALSE}, {"DO"=enum."*Abilita potenza trifase", "Value"=FALSE}, {"DO"=enum."*Abilita potenza monofase", "Value"=FALSE}, {"DO"=enum."*ABILITA freno 1", "Value"=FALSE}, {"DO"=enum."*ABILITA alimentatore 1", "Value"=FALSE}]) -> ()  [unwired: 10 in, 1 out]
                    }
                  }
                }
              }
              frame 1 {
                n515 = while {
                  shift-right: [w1504] -> _
                  shift-left: "Disabilita" -> [w1505]
                  tunnel: w1500 -> [w1503]
                  tunnel: [w1502] -> w1499
                  stop <- TRUE stop-if-true
                  n516 = case shown="\"Attendi\"" w1505 {
                    selector: w1505 -> [w1512 w1519 _]
                    tunnel: [w1511 w1519 "Attendi"] -> w1504
                    tunnel: w1503 -> [w1517 _ _]
                    tunnel: [_ TRUE _] -> w1502
                    frame "Attendi" {
                      n517 = Unbundle By Name(w1517) -> ("MISURE ALL.INTERFACCIA.DI (logici).ALIM 2 abilitato"=w1516:bool, "MISURE ALL.INTERFACCIA.DI (logici).FRENO 2 abilitato"=w1515:bool, "MISURE ALL.INTERFACCIA.DI (logici).Potenza trifase abilitata"=w1514:bool, "MISURE ALL.INTERFACCIA.DI (logici).Teleruttore WT abilitato"=w1509:bool, "MISURE ALL.INTERFACCIA.DI (logici).FRENO 1 abilitato"=w1508:bool, "MISURE ALL.INTERFACCIA.DI (logici).ALIM 1 abilitato"=w1507:bool)
                      n518 = Compound Arithmetic op=OR(w1516, w1515, w1514, w1509, w1508, w1507) -> (w1513:bool)
                      n519 = Select(t=w1512, s=w1513, f="Fine") -> (s? t:f=w1511:string)
                    }
                    frame "Fine" {
                    }
                    frame "Disabilita", Default {
                      n520 = call "Set DO.vi"("Cluster SET DO"=T13 [{"DO"=enum."B2 Seleziona linea 1", "Value"=FALSE}, {"DO"=enum."B2 Seleziona linea 2", "Value"=FALSE}, {"DO"=enum."B2 Seleziona linea 3", "Value"=FALSE}, {"DO"=enum."B2 Seleziona linea 4", "Value"=FALSE}, {"DO"=enum."*Abilita potenza trifase", "Value"=FALSE}, {"DO"=enum."*ABILITA freno 2", "Value"=FALSE}, {"DO"=enum."*ABILITA alimentatore 2", "Value"=FALSE}]) -> ()  [unwired: 10 in, 1 out]
                    }
                  }
                }
              }
            }
          }
          frame "TELERUTTORI MISURA RESISTENZA RESISTOMAT" {
            # "se equilibrio termico termina tutto"
            n521 = local read "RESISTOMAT"() -> (w1523:T3)
            n522 = local read "Stato"() -> (w1525:string)
            n523 = call "Misura resistomat.vi"("All Data"=w1529, "RESISTOMAT"=w1523, "Stato alimentatore 1"=w1527, "Stato comandi freno"=w1528, "Stato"=w1525) -> ("termina tutto?"=w1522:bool, "fine"=w1526:bool, "t"=w1524:string)  [unwired: 4 in]
            n524 = local write "Stato"(w1524) -> ()
          }
          frame "FINE" {
            w1534 = T5[] [] items=["FINE", "FRENO ABILITA", "FRENO DISABILITA", "FRENO MARCIA ON", "FRENO MARCIA OFF", "FRENO SET RIF PARTENZA", "FRENO FORZA RIF FERMATA", "FRENO SET RIF FERMATA", "FRENO SET RIF A 0", "FRENO FORZA RIF A 0", "FRENO SET CONTROLLO COPPIA", "FRENO SET CONTROLLO VELOCITA'", "FRENO SET SENSO ROTAZIONE", "FRENO SET SENS ROT SEGNO COPPIA", "FRENO CONFIG", "ALIMENTATORE 1 ABILITA", "ALIMENTATORE 1 DISABILITA", "ALIMENTATORE 1 MARCIA ON", "ALIMENTATORE 1 MARCIA OFF", "ALIMENTATORE 1 SET RIF", "ALIMENTATORE 1 SET RIF RIDOTTO", "ALIMENTATORE 1 SET RIF A 0", "ALIMENTATORE 1 RESET ALLARMI", "ALIMENTATORE 1 SCORTA 2", "ALIMENTATORE 1 SCORTA 3", "ALIMENTATORE 2 ABILITA", "ALIMENTATORE 2 DISABILITA", "ALIMENTATORE 2 MARCIA ON", "ALIMENTATORE 2 MARCIA OFF", "ALIMENTATORE 2 SET RIF", "ALIMENTATORE 2 SET RIF RIDOTTO", "ALIMENTATORE 2 SET RIF A 0", "ALIMENTATORE 2 SCORTA 1", "ALIMENTATORE 2 SCORTA 2", "ALIMENTATORE 2 SCORTA 3", "TELERUTTORI CHIUDI POTENZA", "TELERUTTORI APRI POTENZA", "TELERUTTORI ABILITA POTENZA", "TELERUTTORI DISABILITA POTENZA", "TELERUTTORI MISURA RESISTENZA RESISTOMAT", "TELERUTTORI MISURA RESISTENZA RES METER", "PROCEDURA ROTORE BLOCCATO 1", "ATTENDI FERMATA MOTORE", "SEGNALA INIZIO AVVIO", "SEGNALA FINE AVVIO", "SEGNALA INIZIO FERMATA", "SEGNALA FINE FERMATA", "START PROFILO", "ATTENDI FINE RAMPA"]  # empty
            n525 = global write "Global FINE AVVIO.vi" "STOP AFE ALTERNATORI"(FALSE ("AVVISO AVVIO IN CORSO")) -> ()
            n526 = global write "Global FINE AVVIO.vi" "START AFE ALTERNATORI"(FALSE ("AVVISO AVVIO IN CORSO")) -> ()
            n527 = global write "Global FINE AVVIO.vi" "AVVISO AVVIO IN CORSO"(FALSE ("AVVISO AVVIO IN CORSO")) -> ()
          }
          frame "ALIMENTATORE 2 MARCIA ON" {
          }
          frame "ALIMENTATORE 2 MARCIA OFF" {
          }
          frame "ALIMENTATORE 2 SET RIF" {
          }
          frame "ALIMENTATORE 2 SET RIF RIDOTTO" {
          }
          frame "ALIMENTATORE 2 SET RIF A 0" {
          }
          frame "ALIMENTATORE 2 SCORTA 1" {
          }
          frame "ALIMENTATORE 2 SCORTA 2" {
          }
          frame "ALIMENTATORE 2 SCORTA 3" {
          }
          frame "TELERUTTORI MISURA RESISTENZA RES METER" {
            n528 = local read "Rami misura"() -> (w1543:i32)
            n529 = local read "Stato"() -> (w1545:string)
            n530 = call "Misura freddo res meter.vi"("#rami misura"=w1543, "Stato alimentatore 1"=w1548, "Stato"=w1545, "Stato comandi freno"=w1547) -> ("Fine"=w1546:bool, "t"=w1544:string)  [unwired: 6 in]
            n531 = local write "Stato"(w1544) -> ()
          }
          frame "ALIMENTATORE 2 ABILITA" {
          }
          frame "ALIMENTATORE 2 DISABILITA" {
          }
          frame "SEGNALA FINE AVVIO" {
            n532 = global write "Global prova in corso.vi" "prova in corso?"(TRUE ("prova in corso?")) -> ()
            n533 = global write "Global FINE AVVIO.vi" "FINE AVVIO"(TRUE ("FINE AVVIO")) -> ()
            n534 = global write "Global_bypass_ResMeter.vi" "Bypass res meter"(FALSE ("Bypass res meter")) -> ()
          }
          frame "SEGNALA INIZIO FERMATA" {
            n535 = global write "Global FINE AVVIO.vi" "AVVISO FERMATA IN CORSO"(TRUE ("AVVISO FERMATA IN CORSO")) -> ()
            n536 = global write "Global FINE AVVIO.vi" "FINE FERMATA"(FALSE ("FINE FERMATA")) -> ()
            n537 = global write "Global Trampa 0.vi" "Forza rif"(TRUE ("Rampa a 0")) -> ()
          }
          frame "SEGNALA FINE FERMATA" {
            n538 = global write "Global FINE AVVIO.vi" "AVVISO FERMATA IN CORSO"(FALSE ("AVVISO FERMATA IN CORSO")) -> ()
            n539 = global write "Global FINE AVVIO.vi" "FINE FERMATA"(TRUE ("FINE FERMATA")) -> ()
            n540 = global write "Global Trampa 0.vi" "Forza rif"(FALSE ("Rampa a 0")) -> ()
          }
          frame "SEGNALA INIZIO AVVIO" {
            n541 = global write "Global FINE AVVIO.vi" "AVVISO AVVIO IN CORSO"(TRUE ("AVVISO AVVIO IN CORSO")) -> ()
            n542 = global write "Global FINE AVVIO.vi" "FINE AVVIO"(FALSE ("FINE AVVIO")) -> ()
          }
          frame "PROCEDURA ROTORE BLOCCATO 1" {
            n543 = while {
              tunnel: [w1577] -> w1571
              shift-right: [w1574] -> _
              shift-left: _ -> [w1573]
              stop <- TRUE stop-if-true
              n544 = local read "Stato"() -> (w1576:string)
              n545 = case shown="\"wait\"" w1576 {
                selector: w1576 -> [w1587 _]
                tunnel: [w1586 "wait" ("t")] -> w1575
                tunnel: [w1582 _] -> w1577
                tunnel: [_ TRUE] -> w1574
                tunnel: w1573 -> [w1583 _]
                frame "wait" {
                  n546 = local read "TEMPO PROVA ROT BLOCC"() -> (w1584:dbl)
                  n547 = call "Elapsed Time23"("Time Target (s)"=0.25, "Auto Reset"=TRUE) -> ("Time has Elapsed"=w1579:bool)  [unwired: 10 in, 7 out]
                  n548 = case shown="True" w1579 {
                    frame False {
                    }
                    frame True {
                      n549 = Bundle By Name(cluster=T12 {"Array of elements"=[], "Single element"={"String"="START ACQ", "variant"=variant}, "enque at\nopposite end (F)"=FALSE, "no replications (F)"=FALSE} ("Enqueue cluster"), "Single element.variant"=T20 {"N°Acq"=0, "Periodo"=0.0, "acq in corso"=FALSE, "Acquisizione"=FALSE, "Slide"=2, "Inserisci Acq."=FALSE, "Elimina riga"=FALSE, "Acq auto"=FALSE, "Intervallo"=5.0} ("Acquisizioni")) -> (w1593:T12)
                      n550 = call <userlib>:"SMQ_MANAGER.vi"("Function"=enum16{"INITIALIZE", "ENQUEUE", "STOP ALL"}."ENQUEUE", "Queue name"="READ_DATA_2_Q", "Enqueue cluster"=w1593) -> ()  [unwired: 8 in, 1 out]
                    }
                  }
                  n551 = call "Elapsed Time21"("Time Target (s)"=w1584, "Reset"=w1583, "Auto Reset"=FALSE) -> ("Time has Elapsed"=w1582:bool)  [unwired: 9 in, 7 out]
                  n552 = case shown="True" w1582 {
                    frame False {
                    }
                    frame True {
                      n553 = global write "Global prova in corso.vi" "prova in corso?"(TRUE ("prova in corso?")) -> ()
                    }
                  }
                  n554 = Select(t="Fine", s=w1582, f=w1587) -> (s? t:f=w1586:string)
                }
                frame "Init", Default {
                  n555 = global write "Global prova in corso.vi" "prova in corso?"(TRUE ("prova in corso?")) -> ()
                }
              }
              n556 = local write "Stato"(w1575) -> ()
            }
          }
          frame "ATTENDI FERMATA MOTORE" {
            n557 = Unbundle By Name(w1614) -> ("MISURE ALL.STATO PLC 1.AI plc.RPM freno"=w1607:dbl, "MISURE ALL.STATO PLC 3.AI plc.RPM freno"=w1606:dbl)
            n558 = Unbundle By Name(w1603) -> ("banco selezionato"=w1599:i8)
            n559 = Absolute Value(x=w1607) -> (abs(x)=w1612:dbl)
            n560 = Absolute Value(x=w1606) -> (abs(x)=w1605:dbl)
            n561 = Less?(x=w1605, y=100) -> (x < y?=w1601:bool)
            n562 = Less?(x=w1612, y=300) -> (x < y?=w1602:bool)
            n563 = Build Array(w1602, w1601) -> (w1600:bool[])
            n564 = Index Array(array=w1600, index=w1599) -> (element=w1598:bool)
            n565 = Not(x=w1598) -> (.not. x?=w1610:bool)
            n566 = call "Elapsed Time11"("Time Target (s)"=2.0, "Reset"=w1610, "Auto Reset"=FALSE) -> ("Time has Elapsed"=w1609:bool)  [unwired: 9 in, 7 out]
          }
          frame "START PROFILO" {
            n567 = Obtain Queue(name (unnamed)="GESTORE PROFILI", element data type=T8 {"Message"="", "Message Data"=variant} ("Message Cluster")) -> (queue out=w1618:refnum<queue>, error out=w1617:errorcluster)  [unwired: 3 in, 1 out]
            n568 = Enqueue Element(queue=w1618, element=cluster{"Status":string, "variant":variant} {"Status"="START PROFILO", "variant"=variant}, error in (no error)=w1617) -> ()  [unwired: 1 in, 3 out]
          }
          frame "FRENO FORZA RIF FERMATA" {
            n569 = flat-sequence {
              frame #0 {
                n570 = global write "Global Trampa 0.vi" "Forza rif"(TRUE ("Rampa a 0")) -> ()
              }
              frame #1 {
                # "SANTERNO: RIF BASSO. la resistenza di frenatura\nè collegata all'alimentatore, che sembra non frenare\nse abilitato ma non fuori marcia. (in questo punto è \ngià fuori marcia). Se alzo troppo il riferimento di frenatura\nil freno va in allarme di overvoltage.\nSi ferma comunque in tempo accettabili anche con\nrif bassi"
                # "rif in %"
                n571 = call "SET AO.vi"("Cluster SET AO"=T17 [{"AO"=enum."RIF COPPIA FRENO 1", "Value"=0.15}, {"AO"=enum."RIF COPPIA FRENO 2", "Value"=5.0}]) -> ()  [unwired: 10 in, 1 out]
              }
            }
          }
        }
        n572 = property on="OPERAZIONE IN CORSO" class="Enum (strict)"() -> ("RingText.Text"=w514:string)  [unwired: 2 in, 2 out]
        n573 = local read "Stato"() -> (w512:string)
        n574 = local read "PROCEDURA"() -> (w519:string)
        n575 = Concatenate Strings(w519, " IN CORSO....", w514, "  (" ("string"), w512, ")" ("string")) -> (w516:string)
        n576 = feedback-in #1(w516) -> ()
        n577 = feedback #1() -> (w517:string)  [unwired: 1 in]
        n578 = case shown="False" w507 {
          tunnel: [w539 w547] -> w532
          tunnel: w526 -> [w538 _]
          tunnel: w521 -> [w537 _]
          tunnel: w509 -> [w536 _]
          tunnel: [w536 w546] -> w508
          frame False {
            n579 = case shown="False" w538 {
              tunnel: w537 -> [w540 w544]
              tunnel: [w540 w543] -> w539
              frame False {
              }
              frame True {
                n580 = Delete From Array(array=w544, length=1, index=0) -> (array with subset deleted=w543:T5[])  [unwired: 1 out]
                "Stato" <- "Default" ("Stato")
              }
            }
          }
          frame True {
            w546 = T5[][] [] items=["FINE", "FRENO ABILITA", "FRENO DISABILITA", "FRENO MARCIA ON", "FRENO MARCIA OFF", "FRENO SET RIF PARTENZA", "FRENO FORZA RIF FERMATA", "FRENO SET RIF FERMATA", "FRENO SET RIF A 0", "FRENO FORZA RIF A 0", "FRENO SET CONTROLLO COPPIA", "FRENO SET CONTROLLO VELOCITA'", "FRENO SET SENSO ROTAZIONE", "FRENO SET SENS ROT SEGNO COPPIA", "FRENO CONFIG", "ALIMENTATORE 1 ABILITA", "ALIMENTATORE 1 DISABILITA", "ALIMENTATORE 1 MARCIA ON", "ALIMENTATORE 1 MARCIA OFF", "ALIMENTATORE 1 SET RIF", "ALIMENTATORE 1 SET RIF RIDOTTO", "ALIMENTATORE 1 SET RIF A 0", "ALIMENTATORE 1 RESET ALLARMI", "ALIMENTATORE 1 SCORTA 2", "ALIMENTATORE 1 SCORTA 3", "ALIMENTATORE 2 ABILITA", "ALIMENTATORE 2 DISABILITA", "ALIMENTATORE 2 MARCIA ON", "ALIMENTATORE 2 MARCIA OFF", "ALIMENTATORE 2 SET RIF", "ALIMENTATORE 2 SET RIF RIDOTTO", "ALIMENTATORE 2 SET RIF A 0", "ALIMENTATORE 2 SCORTA 1", "ALIMENTATORE 2 SCORTA 2", "ALIMENTATORE 2 SCORTA 3", "TELERUTTORI CHIUDI POTENZA", "TELERUTTORI APRI POTENZA", "TELERUTTORI ABILITA POTENZA", "TELERUTTORI DISABILITA POTENZA", "TELERUTTORI MISURA RESISTENZA RESISTOMAT", "TELERUTTORI MISURA RESISTENZA RES METER", "PROCEDURA ROTORE BLOCCATO 1", "ATTENDI FERMATA MOTORE", "SEGNALA INIZIO AVVIO", "SEGNALA FINE AVVIO", "SEGNALA INIZIO FERMATA", "SEGNALA FINE FERMATA", "START PROFILO", "ATTENDI FINE RAMPA"]
            w547 = T5[] [] items=["FINE", "FRENO ABILITA", "FRENO DISABILITA", "FRENO MARCIA ON", "FRENO MARCIA OFF", "FRENO SET RIF PARTENZA", "FRENO FORZA RIF FERMATA", "FRENO SET RIF FERMATA", "FRENO SET RIF A 0", "FRENO FORZA RIF A 0", "FRENO SET CONTROLLO COPPIA", "FRENO SET CONTROLLO VELOCITA'", "FRENO SET SENSO ROTAZIONE", "FRENO SET SENS ROT SEGNO COPPIA", "FRENO CONFIG", "ALIMENTATORE 1 ABILITA", "ALIMENTATORE 1 DISABILITA", "ALIMENTATORE 1 MARCIA ON", "ALIMENTATORE 1 MARCIA OFF", "ALIMENTATORE 1 SET RIF", "ALIMENTATORE 1 SET RIF RIDOTTO", "ALIMENTATORE 1 SET RIF A 0", "ALIMENTATORE 1 RESET ALLARMI", "ALIMENTATORE 1 SCORTA 2", "ALIMENTATORE 1 SCORTA 3", "ALIMENTATORE 2 ABILITA", "ALIMENTATORE 2 DISABILITA", "ALIMENTATORE 2 MARCIA ON", "ALIMENTATORE 2 MARCIA OFF", "ALIMENTATORE 2 SET RIF", "ALIMENTATORE 2 SET RIF RIDOTTO", "ALIMENTATORE 2 SET RIF A 0", "ALIMENTATORE 2 SCORTA 1", "ALIMENTATORE 2 SCORTA 2", "ALIMENTATORE 2 SCORTA 3", "TELERUTTORI CHIUDI POTENZA", "TELERUTTORI APRI POTENZA", "TELERUTTORI ABILITA POTENZA", "TELERUTTORI DISABILITA POTENZA", "TELERUTTORI MISURA RESISTENZA RESISTOMAT", "TELERUTTORI MISURA RESISTENZA RES METER", "PROCEDURA ROTORE BLOCCATO 1", "ATTENDI FERMATA MOTORE", "SEGNALA INIZIO AVVIO", "SEGNALA FINE AVVIO", "SEGNALA INIZIO FERMATA", "SEGNALA FINE FERMATA", "START PROFILO", "ATTENDI FINE RAMPA"] ("empty")
          }
        }
        n581 = Empty Array?(array=w532) -> (empty?=w530:bool)
        n582 = Not Equal?(x=w516, y=w517) -> (x != y?=w515:bool)
        n583 = case shown="False" w515 {
          tunnel: w516 -> [_ w549]
          tunnel: w507 -> [_ w548]
          frame False {
          }
          frame True {
            n584 = case shown="False" w548 {
              tunnel: w549 -> [w550 _]
              frame False {
                n585 = Bundle By Name(cluster=T12 {"Array of elements"=[], "Single element"={"String"="AGGIORNA STATUS", "variant"=variant}, "enque at\nopposite end (F)"=FALSE, "no replications (F)"=FALSE} ("Enqueue cluster"), "Single element.variant"=w550) -> (w554:T12)
                n586 = call <userlib>:"SMQ_MANAGER.vi"("Function"=enum16{"INITIALIZE", "ENQUEUE", "STOP ALL"}."ENQUEUE", "Queue name"="MAIN_Q", "Enqueue cluster"=w554) -> ()  [unwired: 8 in, 1 out]
              }
              frame True {
                n587 = Bundle By Name(cluster=T12 {"Array of elements"=[], "Single element"={"String"="AGGIORNA STATUS", "variant"=variant}, "enque at\nopposite end (F)"=FALSE, "no replications (F)"=FALSE} ("Enqueue cluster"), "Single element.variant"="PROVA TERMICA TERMINATA AUTOMATICAMENTE") -> (w559:T12)
                n588 = call <userlib>:"SMQ_MANAGER.vi"("Function"=enum16{"INITIALIZE", "ENQUEUE", "STOP ALL"}."ENQUEUE", "Queue name"="MAIN_Q", "Enqueue cluster"=w559) -> ()  [unwired: 8 in, 1 out]
              }
            }
          }
        }
        n589 = case shown="False" w530 {
          tunnel: w531 -> [w561 w564]
          tunnel: [_ TRUE] -> w529
          frame False {
            n590 = Enqueue Element(queue=w561, element=cluster{"Status":string, "variant":variant} {"Status"="ESEGUI", "variant"=variant}) -> ()  [unwired: 2 in, 3 out]
          }
          frame True {
            n591 = Enqueue Element(queue=w564, element=cluster{"Status":string, "variant":variant} {"Status"="ESTRAI PROCEDURA", "variant"=variant}) -> ()  [unwired: 2 in, 3 out]
          }
        }
      }
      frame "AGGIORNA INFO" {
        n592 = Variant To Data(type=T21 {"Scelta wattmetro"={"Wattmetro"=enum."No Selection"}, "SET RPM"=0.0, "SET TEMP"=0.0, "Array banchi"=[{"Nome"="BANCO1", "Tors. scala1"=0, "Tors. scala2"=1, "rpm"=0, "TAMB"=1, "Indici Temperature"=[1, 2, 3], "Indice freno"=0, "alimentatore trifase"=0, "alimentatore monofase"=0, "alimentatore dc arm"=0, "alimentatore dc ecc"=0, "alimentatore dc mp"=0}], "Array valvole linee avvio/fermata"=[], "banco selezionato"=0, "Nomi valvole prop sistema"=[], "canale-- sensore"=[], "Attriti B1"=[], "Attriti B2"=[], "Collegamento elettrico"={"ALIMENTAZIONE ELETTRICA"=enum."AC TRIFASE + FRENO", "ID"=3, "#rami freddo\\eq term resmeter"=1, "#rami riscaldamento resmeter"=1, "#rami freddo\\eq term resistomat"=1, "#rami riscaldamento resistomat"=1, "CALCOLI"=enum."AC TRIFASE"}, "lingua"=0, "Costanti collaudo"={"P [bar]"=0.0, "T amb. [°C]"=0.0, "Umidità [%]"=0.0, "T acqua [°C] 2"=0.0}, "OPZIONI MISURE RES"={"MISURA A FREDDO"=enum."ENTRAMBI", "MISURA EQ. TERMICO"=enum."RESISTOMAT", "MISURA DT PROVA IN CORSO"=enum."RESISTOMAT - CON FERMATE", "MISURE PRIMA E DOPO"=enum."RESISTOMAT", "STRUMENTI PRESENTI"=enum."ENTRAMBI"}, "Dati targa motore"={"Vnom"=0.0, "Fnom"=0.0, "Inom"=0.0, "Cnom"=0.0, "Npoli"=0.0, "Scorta 1"=0.0, "Scorta 2"=0.0, "Scorta 3"=0.0}} ("Cluster INFO"), Variant=w1634) -> (data=w1627:T21)  [unwired: 1 in, 1 out]
      }
    }
    "Matrice procedure" <- w34
    "Operazioni in corso" <- w29
  }
  n593 = while {
    tunnel: w7 -> [w1637]
    stop <- w1636 stop-if-true
    n594 = event shown="[2] \"AGGIUNGI PROCEDURA  START\": Value Change" {
      selector: _ -> [_ _ _ _ _]
      dyn-events: _ -> [_ _ _ _ _]
      timeout: _ -> [_ _ _ _ _]
      tunnel: w1637 -> [_ w1640 w1646 w1650 w1654]
      tunnel: [_ TRUE _ _ _] -> w1636
      event Timeout {
        n595 = event-data() -> ()  [unwired: 1 in, 3 out]
      }
      event "EXIT": Value Change {
        n596 = event-data() -> ()  [unwired: 1 in, 6 out]
        n597 = Enqueue Element(queue=w1640, element=T8 {"Message"="EXIT", "Message Data"=variant}) -> ()  [unwired: 2 in, 3 out]
      }
      event "AGGIUNGI PROCEDURA \nSTART": Value Change {
        n598 = event-data() -> ()  [unwired: 1 in, 6 out]
        n599 = Bundle By Name(cluster=cluster{"PROCEDURE":T4, "Variant":variant} {"PROCEDURE"=enum."START", "Variant"=variant}, "Variant"="Cluster") -> (w1642:cluster{"PROCEDURE":T4, "Variant":variant})
        n600 = Bundle By Name(cluster=cluster{"Status":string, "variant":variant} {"Status"="AGGIUNGI PROCEDURA", "variant"=variant}, "variant"=w1642) -> (w1644:cluster{"Status":string, "variant":variant})
        n601 = Enqueue Element At Opposite End(queue=w1646, element=w1644) -> ()  [unwired: 2 in, 3 out]
      }
      event "AGGIUNGI PROCEDURA \nSTOP": Value Change {
        n602 = event-data() -> ()  [unwired: 1 in, 6 out]
        n603 = Bundle By Name(cluster=cluster{"Status":string, "variant":variant} {"Status"="AGGIUNGI PROCEDURA", "variant"=variant}, "variant"=cluster{"PROCEDURE":T4, "Variant":variant} {"PROCEDURE"=enum."STOP AUTOMATICO", "Variant"=variant}) -> (w1648:cluster{"Status":string, "variant":variant})
        n604 = Enqueue Element At Opposite End(queue=w1650, element=w1648) -> ()  [unwired: 2 in, 3 out]
      }
      event "AGGIUNGI PROCEDURA Abilita potenza": Value Change {
        n605 = event-data() -> ()  [unwired: 1 in, 6 out]
        n606 = Bundle By Name(cluster=cluster{"PROCEDURE":T4, "Variant":variant} {"PROCEDURE"=enum."ABILITA POTENZA", "Variant"=variant}, "Variant"="Cluster Colleg/LInea Elettrica") -> (w1652:cluster{"PROCEDURE":T4, "Variant":variant})
        n607 = Bundle By Name(cluster=cluster{"Status":string, "variant":variant} {"Status"="AGGIUNGI PROCEDURA", "variant"=variant}, "variant"=w1652) -> (w1655:cluster{"Status":string, "variant":variant})
        n608 = Enqueue Element At Opposite End(queue=w1654, element=w1655) -> ()  [unwired: 2 in, 3 out]
      }
    }
  }
  n609 = global write "Global FINE AVVIO.vi" "STOP AFE ALTERNATORI"(w1) -> ()
  n610 = global write "Global FINE AVVIO.vi" "START AFE ALTERNATORI"(w1) -> ()
